vi "Main_Marvin Remake.vi"() -> ()   [LabVIEW 2017]
uses:
  Marvin ATP Remake 6.5.18 - Copy/PCAN_Driver/ControlCAN.llb/DevType.ctl
  Marvin ATP Remake 1.5.18/PCAN_Driver/ControlCAN.llb/CAN Channel.ctl
  Marvin ATP Remake 6.5.18 - Copy/PCAN_Driver/ControlCAN.llb/VCI_INIT_CONFIG.ctl
  Marvin ATP Remake 6.5.18 - Copy/PCAN_Driver/ControlCAN.llb/InitFlag.ctl
  Marvin ATP Remake 6.5.18 - Copy/PCAN_Driver/ControlCAN.llb/Fliter.ctl
  Marvin ATP Remake 6.5.18 - Copy/PCAN_Driver/ControlCAN.llb/Mode.ctl
  <vilib>/Utility/miscctls.llb/LVRowAndColumnTypeDef.ctl
  <vilib>/Utility/sysdir.llb/System Directory Type.ctl
  <vilib>/Utility/config.llb/Read Key (String).vi
  <vilib>/Utility/config.llb/Write Key (String).vi
  <vilib>/Utility/cursorutil.llb/Set Cursor (Icon Pict).vi
  Marvin CAN Bus 3.5.18/PCAN_Driver/ControlCAN.lvlib
  <vilib>/Utility/config.llb/NI_LVConfig.lvlib
panel:
  out "DSP Board S/N":string
  out "POWER Board S/N":string caption="DRIVER Board S/N"
  out "TesterVersion":string
  out "ClosePanel":bool=TRUE
  out "UUT SN Report":string
  out "Automation":bool
  out "Test Failed":bool
  out "AuxiOFFResult":bool
  out "AuxiONResult":bool
  out "SensCalResult":bool
  out "VisualInspectionResult":bool
  out "BurnResult":bool
  out "BurnSpeed":bool
  out "BurnTemp":bool
  out "BurnDC":bool
  out "TempControlResult":bool
  out "MotorTempResult":bool
  out "StopTimeResult":bool
  out "SpeedResult":bool=TRUE
  out "VenableDirectionResult":bool
  out "VenableResult":bool
  out "ComTestResult":bool=TRUE
  out "UUT SoftwareVer":string
  out "Next SN":i32
  in  "SetSN":bool
  out "Current SN":i32
  out "Cal":dbl
  out "AO[1]Meas":dbl
  out "FullSpeed2 Speed":dbl
  out "FullSpeed2 Current":dbl
  out "FullSpeed1 Current":dbl
  out "FullSpeed1 Speed":dbl
  out "MaxBurnInTempVal":dbl
  in  "Stop Burn-in":bool
  out "VISA Tester":refnum<visa-resource-name>
  out "UUT":u8
  out "CAN Status":bool
  in  "Channel 2":T1 caption="Channel" items=["Channel 1", "Channel 2"]
  out "Config_CANAT":T7 {"DevType" items=["USB-CAN"=3, "USB-CAN2"=4]; "CanIndex" items=["通道1", "通道2"]; "VCI_INIT_CONFIG"."Fliter" items=["接收所有类型"=3, "只接收标准帧"=4, "只接收扩展帧"=7]; "VCI_INIT_CONFIG"."Mode" items=["正常工作", "自测模式（环回）", "仅侦听模式"]; "VCI_INIT_CONFIG"."InitFlag" items=["使用Flash参数", "使用界面设置参数"]}
  out "Array":u64[][](array[numeric]) format="%016x"
  out "Motor Phase Current RMS":dbl
  out "Ambient Temperature":dbl
  out "Speed error":bool
  out "Commutation err":bool
  out "Under voltage/Over voltage":bool
  out "Derated drive temp":bool
  out "Motor Over temperature":bool
  out "Motor Sensor temp Fauilre":bool
  out "Drive Over temperature":bool
  out "Drive Sensor temp Failure":bool
  out "Ambient Over temp":bool
  out "Ambient Sensor temp":bool
  out "DC Voltage":dbl
  out "DC Current":dbl
  out "Power transistor Heat sink Temp.":dbl
  out "Motor Stator Temp.":dbl
  out "Motor Speed RPM":dbl
  out "ECS State":u16
  out "UUT":string="EBAY"
  in  "Logger Path":path
  in  "Report":bool
  in  "Start":bool
  in  "ATR":string[][](table)=[["Test Communication", "-", "-", "-", "-", ""], ["Set S/N", "-", "-", "-", "-", ""], ["Set Board Number", "-", "-", "-", "-", ""], [" ", "", "", "", "", ""], ["Test Communication", "-", "-", "-", "-", ""], ["Get S/N", "-", "-", "-", "", ""], ["Get Board Number", "-", "-", "-", "", ""], ["Get FW", "-", "-", "-", "", ""], ["Enable Motor", "", "", "", "", ""], ["Small position command", "", "", "", "", ""], ["Measure delta", "", "", "", "", ""], ["Velocity command", "", "", "", "", ""]]
  in  "Settings":bool
  in  "Refresh Button":bool
  out "Status":bool
  in  "VISA Marvin":refnum<visa-resource-name>="COM6"
  in  "Serial Com":bool
  in  "Help Button":bool
  out "Pannel User Message":string
  in  "Stop Button":bool
  # "Marvin"
  # "REDLER TECHNOLOGIES LTD"
  # "ver 1.2p"
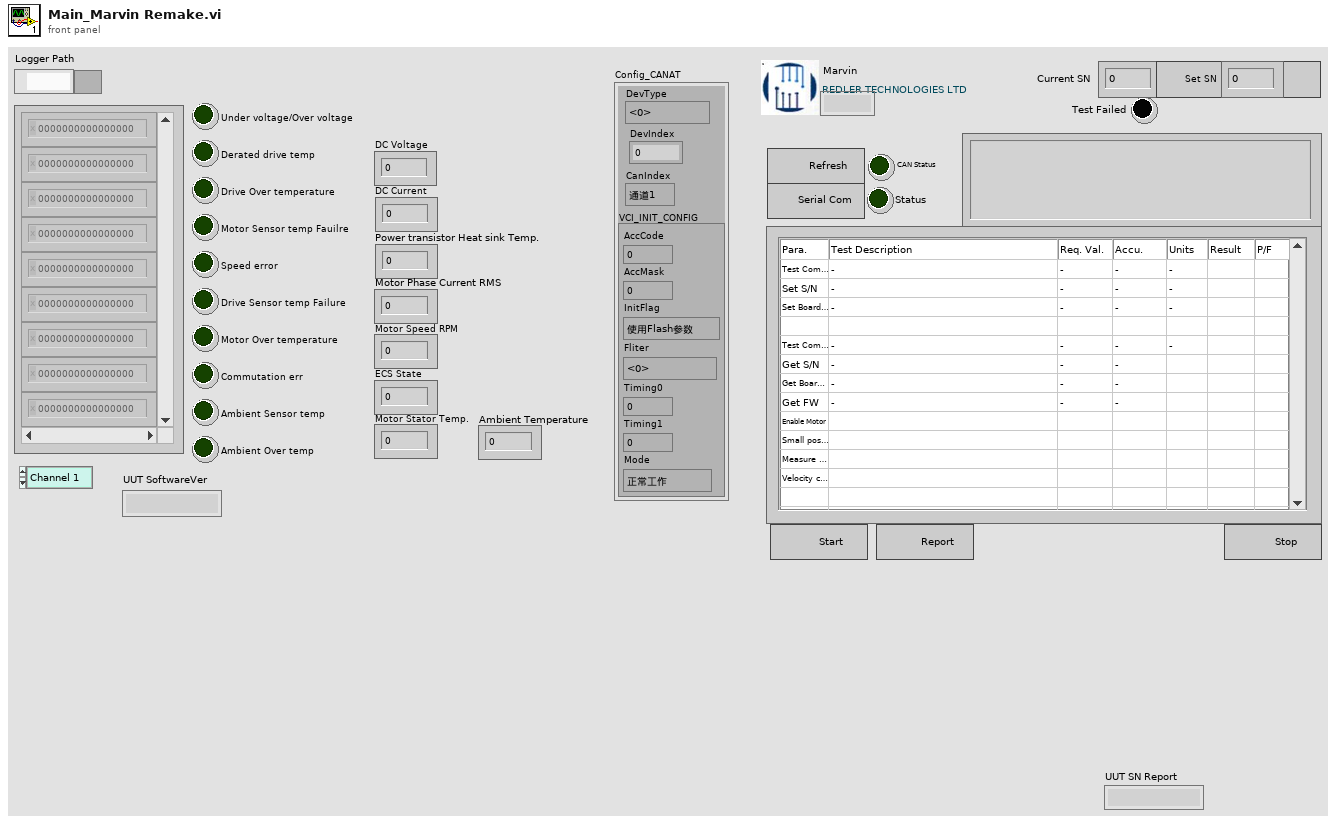
[diagram p1: front panel]
types:
  T1 = typedef "ControlCAN.lvlib/CAN Channel.ctl" = u32
  T2 = typedef "ControlCAN.lvlib/DevType.ctl" = u32
  T3 = typedef "ControlCAN.lvlib/VCI_INIT_CONFIG.ctl" = cluster{"AccCode":u32, "AccMask":u32, "InitFlag":T4, "Fliter":T5, "Timing0":u8, "Timing1":u8, "Mode":T6}
  T4 = typedef "ControlCAN.lvlib/InitFlag.ctl" = u32
  T5 = typedef "ControlCAN.lvlib/Fliter.ctl" = u8
  T6 = typedef "ControlCAN.lvlib/Mode.ctl" = u8
  T7 = cluster{"DevType":T2, "DevIndex":u32, "CanIndex":T1, "VCI_INIT_CONFIG":T3}
  T8 = cluster{"VISA":refnum<visa-resource-name>, "Array Test":enum16{"Auxiliary", "Temp Sens Cal", "Com Test", "Enable Test", "Speed Command", "Stop Time", "Temp Control", "Burn in", "Visual Inspec", "Empty"}[]}
  T9 = cluster{"ID":u32, "MSGTYPE":u8, "LEN":u8, "aDATA":u8[]}[]
  T10 = enum16{"Erase ATR Table", "Stop", "MainProgram", "Initialize"}
  T11 = typedef "NI_LVConfig.lvlib/Config Data RefNum.ctl" = refnum<k1>
  T12 = enum16{"K15", "K16", "K17", "Venable", "Firmeware", "Fan", "Power", "120C", "110C", "100C", "90C", "80C", "70C", "60C", "50C", "40C", "30C", "25C", "20C", "10C", "0C"}
  T13 = enum16{"Stop", "Result", "FullSpeed2", "MD[1]=1", "FullSpeed1", "MD[1]=0"}
  T14 = enum8{"Term1", "Term2", "Current", "Fan", "TempCPU"}
  T15 = enum16{"Stop", "AO[1]=Meas.", "TA[5]", "AO[1]=0", "Start"}
  T16 = enum16{"Stop", "BurnIn", "Ambient Temp", "MotorSpeed", "DC Current Measure", "Start"}
  T17 = enum16{"Auxiliary", "Temp Sens Cal", "Com Test", "Enable Test", "Speed Command", "Stop Time", "Temp Control", "Burn in", "Visual Inspec", "Empty"}[]
  T18 = enum16{"K15", "K16", "K17", "Venable", "Firmeware", "Fan", "Power", "120C", "110C", "100C", "90C", "80C", "70C", "60C", "50C", "40C", "30C", "25C", "20C", "10C", "0C"}[]
  T19 = enum32{"6000", "11500", "15100", "11500-2", "6000-2"}[]
  T20 = enum8{"Enabled", "Disabled", "Disabled and Grayed Out"}
  T21 = typedef "LVRowAndColumnTypeDef.ctl" = cluster{"Row":i32, "Column":i32}
  T22 = enum32{"Invalid", "Standard", "Closed", "Hidden", "Minimized", "Maximized"}
  T23 = cluster{"ID":u32, "MSGTYPE":u8, "LEN":u8, "aDATA":u8[]}
  T24 = enum16{"Auxiliary", "Temp Sens Cal", "Com Test", "Enable Test", "Speed Command", "Stop Time", "Temp Control", "Burn in", "Visual Inspec", "Empty"}
  T25 = enum16{"open", "replace", "create", "open or create", "replace or create", "replace or create with confirmation"}
  T26 = typedef "ControlCAN.lvlib/VCI_CAN_OBJ.ctl" = cluster{"ID":u32, "TimeStamp":u32, "TimeFlag":u8, "SendType":u8, "RemoteFlag":u8, "ExternFlag":u8, "DataLen":u8, "Data":u8[], "Reserved":u8[]}
  T27 = cluster{"Type":enum16{"接收", "发送"}, "Channel":T1, "Time":timestamp, "VCI_CAN_OBJ":T26}[]
  T28 = cluster{"Type":enum16{"接收", "发送"}, "Channel":T1, "Time":timestamp, "VCI_CAN_OBJ":T26}
  T29 = typedef "LVPoint32TypeDef.ctl" = cluster{"Horizontal":i32, "Vertical":i32}
  T30 = enum8{"Term1", "Term2", "Current", "Fan", "TempCPU"}[]
  T31 = typedef "System Directory Type.ctl" = i32
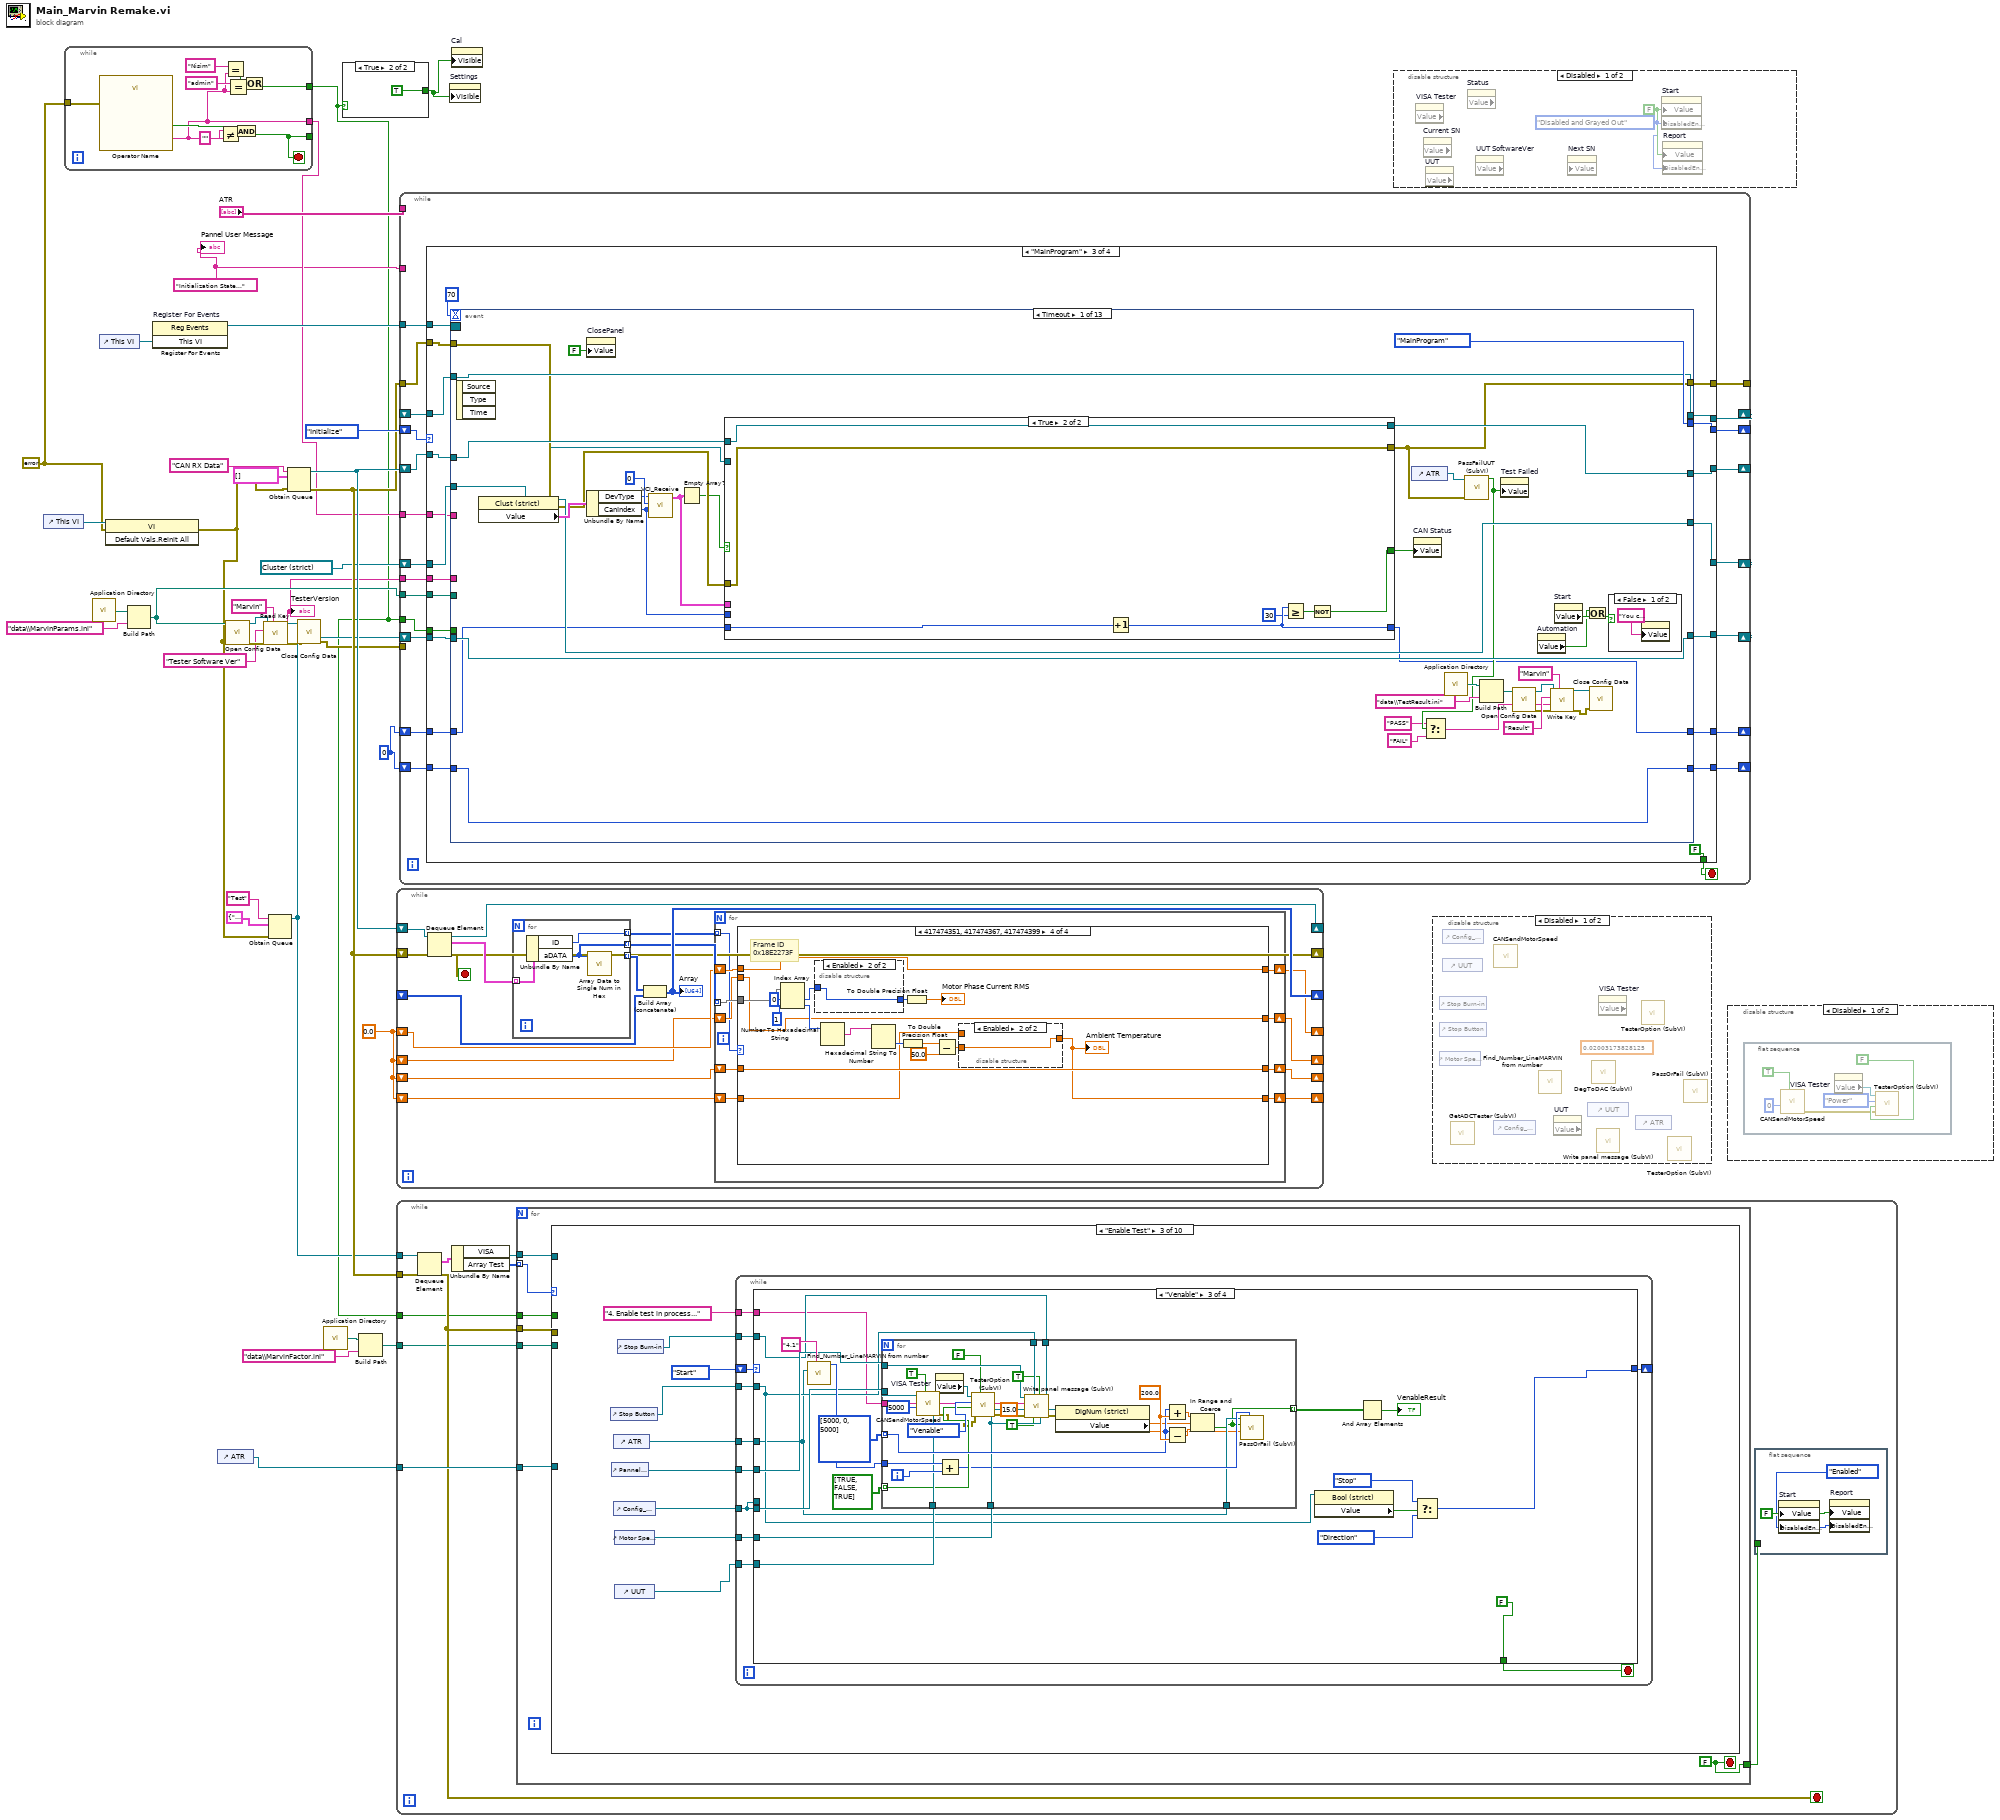
[diagram p0: block diagram]
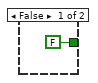
[diagram p2: hidden frame]
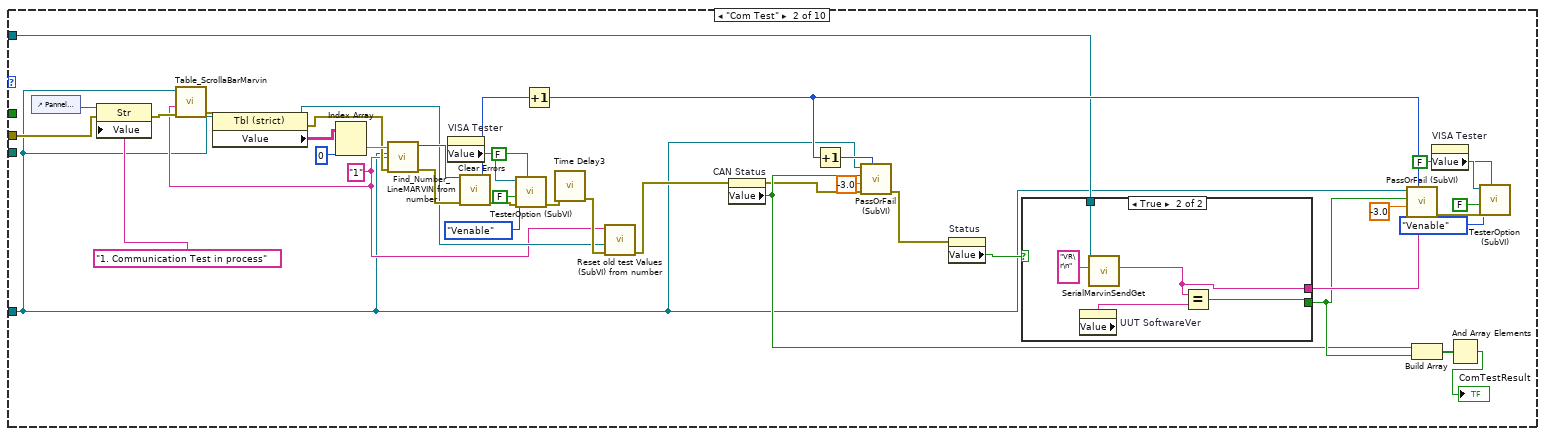
[diagram p7: hidden frame]
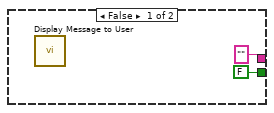
[diagram p8: hidden frame]
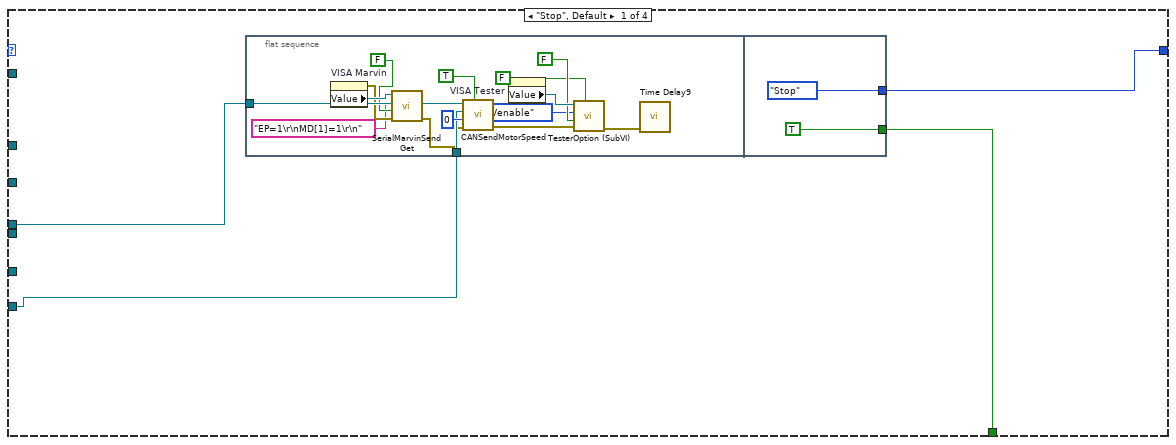
[diagram p9: hidden frame]
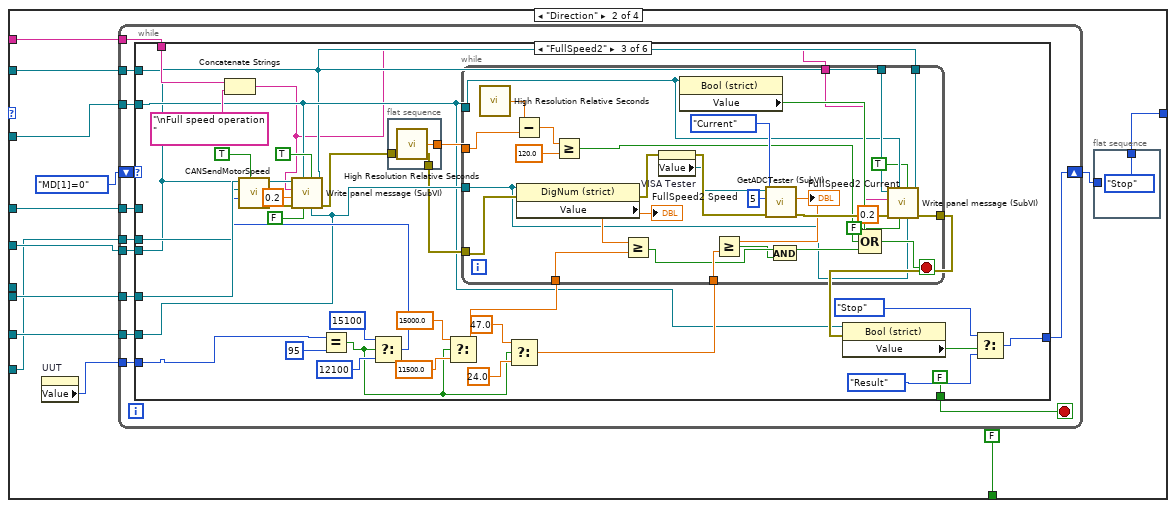
[diagram p10: hidden frame]
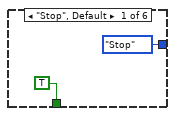
[diagram p11: hidden frame]
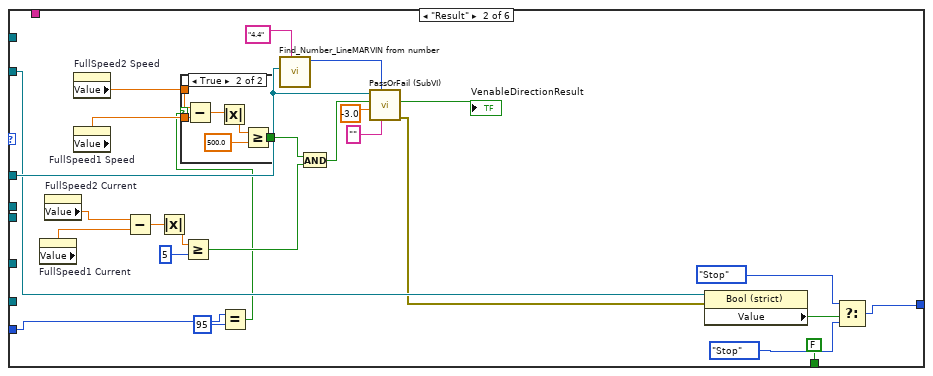
[diagram p12: hidden frame]
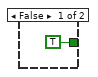
[diagram p13: hidden frame]
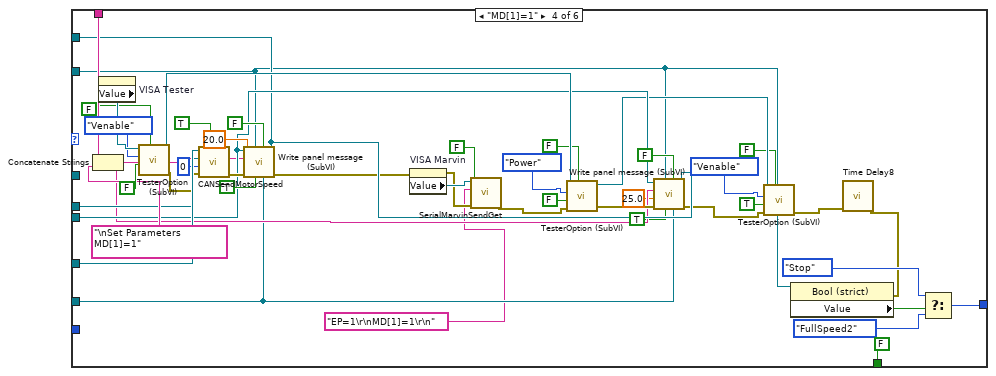
[diagram p14: hidden frame]
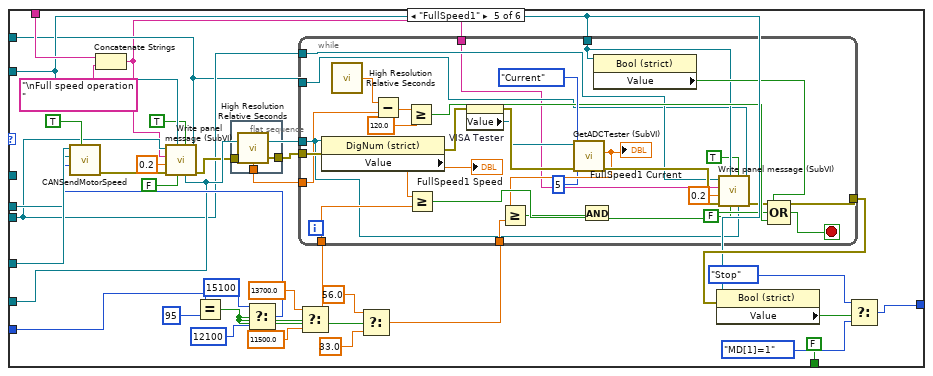
[diagram p15: hidden frame]
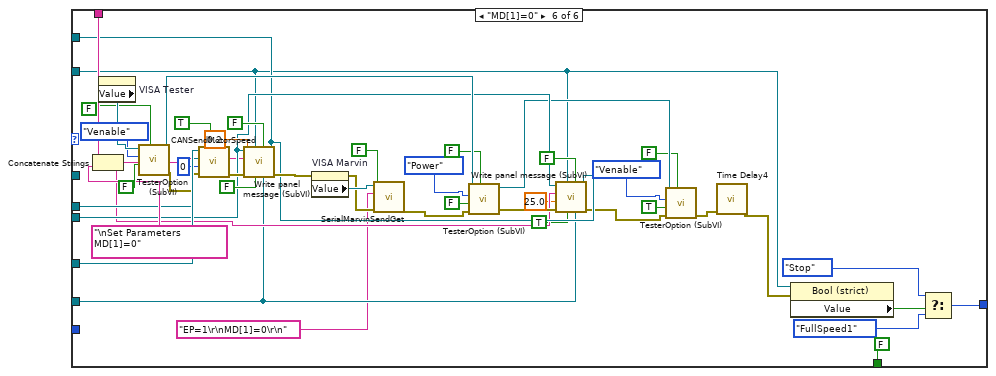
[diagram p16: hidden frame]
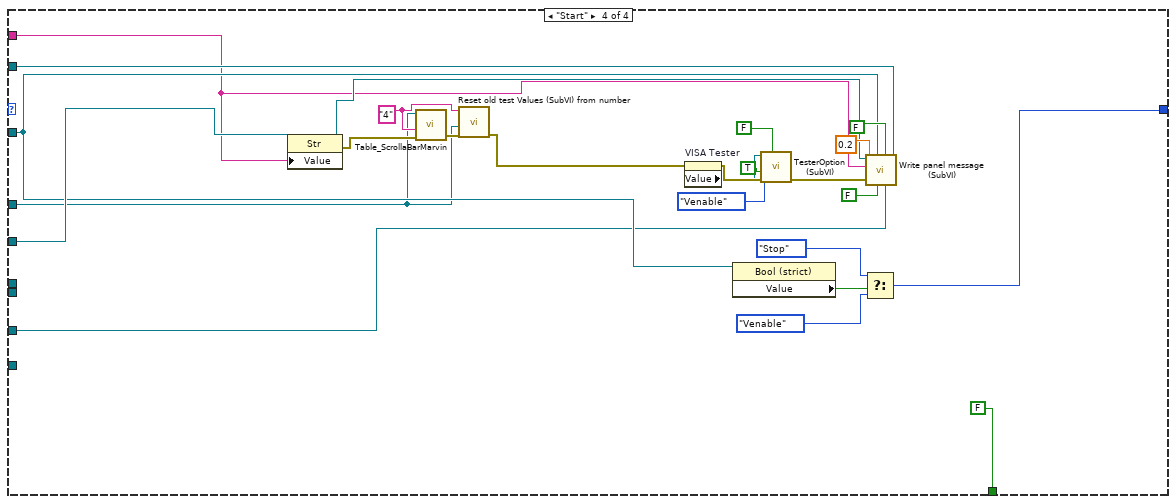
[diagram p17: hidden frame]
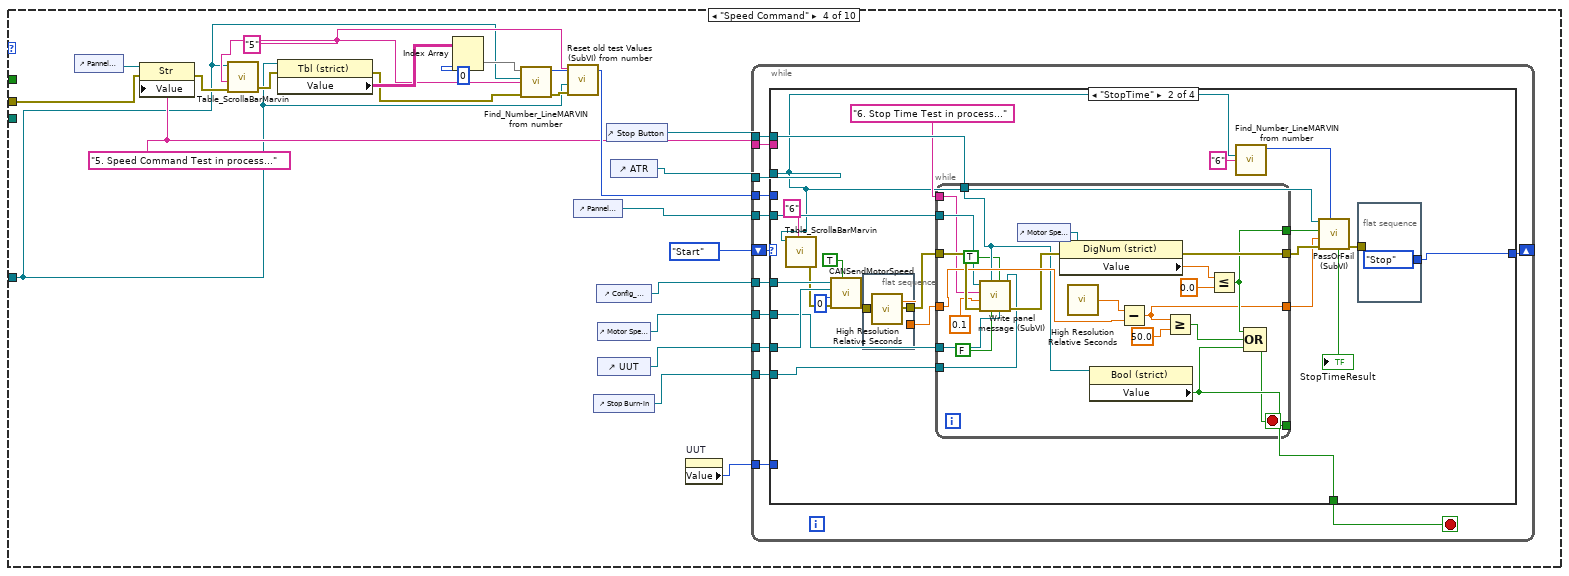
[diagram p18: hidden frame]
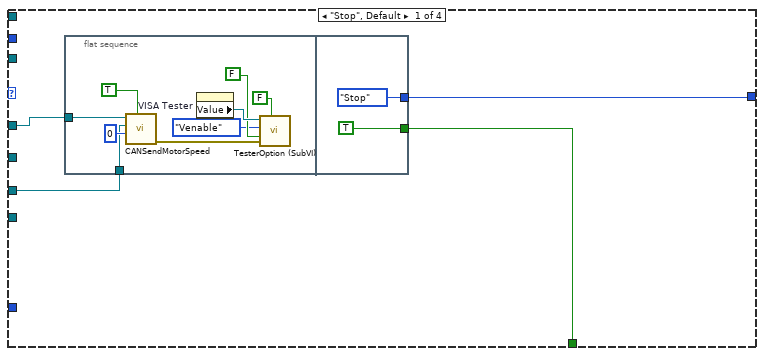
[diagram p19: hidden frame]
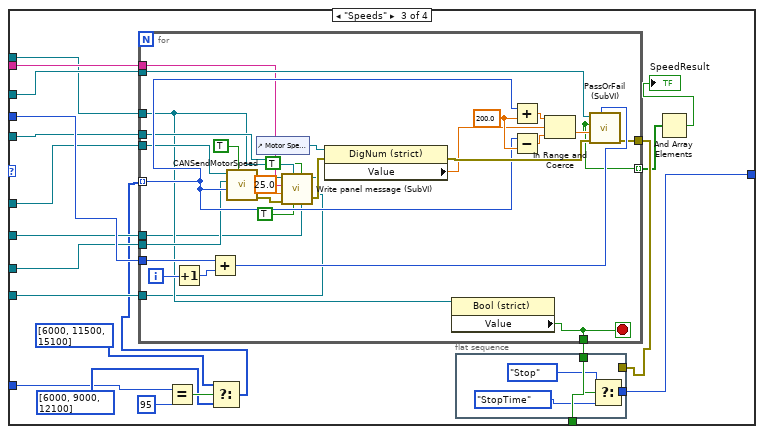
[diagram p20: hidden frame]
diagram:
  w19 = "Initialization State..."
  w1 = 0
  w26 = 0.0
  w4 = errorcluster {"status"=FALSE, "code"=0, "source"=""} ("error in (no error)")
  n1 = control-ref of="This VI"() -> (w5:refnum<vi>)
  n2 = while {
    tunnel: [w44] -> _
    tunnel: [w40] -> w21
    tunnel: [w41] -> w2
    tunnel: w4 -> [w37]
    stop <- w44 stop-if-true
    n3 = call "Operator Name"("error in (no error)"=w37) -> ("Operator Name"=w40:string, "OK"=w45:bool)  [unwired: 16 in, 1 out]
    n4 = Not Equal?(x=w40, y="") -> (x != y?=w46:bool)
    n5 = Equal?(x="Nisim", y=w40) -> (x = y?=w38:bool)
    n6 = Equal?(x="admin", y=w40) -> (x = y?=w42:bool)
    n7 = And(x=w45, y=w46) -> (x .and. y?=w44:bool)
    n8 = Or(x=w38, y=w42) -> (x .or. y?=w41:bool)
  }
  n9 = call <vilib>:"Application Directory.vi"() -> ("Application Directory"=w25:path)
  n10 = control-ref of="This VI"() -> (w23:refnum<vi>)
  n11 = invoke class="VI" method="Default Vals.Reinit All"(reference=w5, error in=w4) -> (error out=w3:errorcluster)  [unwired: 1 in, 2 out]
  n12 = Build Path(base path=w25, name or relative path="data\\MarvinParams.ini") -> (appended path=w8:path)
  n13 = register-events "Register For Events"(w23) -> (reference out=w22:refnum<event-registration>)  [unwired: 2 in, 1 out]
  n14 = control-ref of="ATR"() -> (w18:refnum<vi>)
  n15 = call <vilib>:"Open Config Data.vi"("error in (no error)"=w3, "configuration file path"=w8) -> ("error out"=w14:errorcluster, "refnum"=w13:T11)  [unwired: 1 in, 7 out]
  n16 = call-poly <vilib>:"Read Key.vi"("section"="Marvin", "error in (no error)"=w14, "key"="Tester Software Ver", "refnum"=w13) -> ("error out"=w11:errorcluster, "value"=w6:string, "refnum out"=w10:T11)  [unwired: 2 in, 3 out]
  "TesterVersion" <- w6
  n17 = Obtain Queue(name (unnamed)="Test", element data type=T8 {"VISA"="COM1", "Array Test"=[]}, error in (no error)=w3) -> (queue out=w30:refnum<queue>)  [unwired: 2 in, 2 out]
  n18 = Obtain Queue(name (unnamed)="CAN RX Data", element data type=T9 [], error in (no error)=w3) -> (queue out=w33:refnum<queue>, error out=w31:errorcluster)  [unwired: 2 in, 1 out]
  n19 = call <vilib>:"Close Config Data.vi"("error in (no error)"=w11, "refnum"=w10) -> ("error out"=w9:errorcluster)  [unwired: 8 in, 1 out]
  n20 = call <vilib>:"Application Directory.vi"() -> ("Application Directory"=w16:path)
  n21 = case shown="True" w2 {
    tunnel: [FALSE TRUE] -> w20
    frame False {
    }
    frame True {
    }
  }
  n22 = Build Path(base path=w16, name or relative path="data\\MarvinFactor.ini") -> (appended path=w15:path)
  n23 = while {
    shift-right: [w65] -> _
    shift-left: w33 -> [w67]
    shift-right: [w63] -> _
    shift-left: _ -> [w64]
    shift-right: [w59] -> _
    shift-left: w31 -> [w59]
    shift-right: [w57] -> _
    shift-left: w26 -> [w58]
    shift-right: [w56] -> _
    shift-left: w26 -> [w55]
    shift-right: [w54] -> _
    shift-left: w26 -> [w53]
    shift-right: [w52] -> _
    shift-left: w26 -> [w51]
    stop <- w66 stop-if-true
    n24 = Dequeue Element(queue=w67, error in (no error)=w59) -> (queue out=w65:refnum<queue>, element=w60:T9, error out=w66:errorcluster)  [unwired: 1 in, 1 out]
    n25 = for {
      tunnel: [w217] -> w62 mode=indexing
      tunnel: w60 -> [w216] mode=indexing
      tunnel: [w215] -> w61 mode=indexing
      tunnel: [w214] -> w50 mode=indexing
      n26 = Unbundle By Name(w216) -> ("ID"=w214:u32, "aDATA"=w215:u8[])
      n27 = call "Array Data to Single Num in Hex.vi"("aDATA"=w215) -> ("Numeric"=w217:u64)  [unwired: 10 in]
    }
    n28 = Build Array (concatenate)(w62, w64) -> (w63:u64[][])
    "Array" <- w63
    n29 = for {
      tunnel: w61 -> [w77] mode=indexing
      shift-right: [w75] -> w57
      shift-left: w58 -> [w76]
      shift-right: [w74] -> w56
      shift-left: w55 -> [w73]
      shift-right: [w72] -> w54
      shift-left: w53 -> [w71]
      shift-right: [w70] -> w52
      shift-left: w51 -> [w69]
      tunnel: w50 -> [w68] mode=indexing
      n30 = case shown="417474351, 417474367, 417474399" w68 {
        tunnel: w77 -> [w110 _ w166 w202]
        tunnel: w76 -> [w86 w151 w155 w191]
        tunnel: [w85 w151 w155 w191] -> w75
        tunnel: [w83 w150 w154 w190] -> w74
        tunnel: w73 -> [w82 w150 w154 w190]
        tunnel: [w80 w149 w153 w189] -> w72
        tunnel: w71 -> [w79 w149 w153 w189]
        tunnel: [w78 w148 w152 w187] -> w70
        tunnel: w69 -> [w78 w148 w152 w186]
        frame 417408815, 417408831, 417408863 {
          # "Frame ID\n0x18E1273F"
          n31 = Index Array(array=w110, index #1=0 ("index"), index #2=1 ("index"), index #3=2 ("index"), index #4=3 ("index"), index #5=4 ("index"), index #6=5 ("index"), index #7=6 ("index"), index #8=7 ("index")) -> (element #1=w94:u8, element #2=w96:u8, element #3=w97:u8, element #4=w101:u8, element #5=w104:u8, element #6=w108:u8, element #7=w109:u8, element #8=w107:u8)
          n32 = Number To Hexadecimal String(2:w107) -> (0:w121:string)  [unwired: 1 in]
          n33 = Join Numbers(hi=w109, lo=w108) -> ((hi.lo)=w128:u16)
          n34 = Join Numbers(hi=w97, lo=w96) -> ((hi.lo)=w98:u16)
          n35 = Number To Hexadecimal String(2:w104) -> (0:w105:string)  [unwired: 1 in]
          n36 = Number To Hexadecimal String(2:w128) -> (0:w127:string)  [unwired: 1 in]
          n37 = Number To Hexadecimal String(2:w94) -> (0:w95:string)  [unwired: 1 in]
          n38 = Number To Hexadecimal String(2:w98) -> (0:w99:string)  [unwired: 1 in]
          n39 = Number To Hexadecimal String(2:w101) -> (0:w102:string)  [unwired: 1 in]
          n40 = Hexadecimal String To Number(string=w121) -> (number=w120:u32)  [unwired: 2 in, 1 out]
          n41 = To Double Precision Float(number=w120) -> (double precision float=→"DC Current":dbl)
          n42 = Hexadecimal String To Number(string=w105) -> (number=w106:u32)  [unwired: 2 in, 1 out]
          n43 = Hexadecimal String To Number(string=w127) -> (number=w126:u32)  [unwired: 2 in, 1 out]
          n44 = Hexadecimal String To Number(string=w95) -> (number=w92:u32)  [unwired: 2 in, 1 out]
          n45 = Hexadecimal String To Number(string=w99) -> (number=w100:u32)  [unwired: 2 in, 1 out]
          n46 = Hexadecimal String To Number(string=w102) -> (number=w103:u32)  [unwired: 2 in, 1 out]
          n47 = To Double Precision Float(number=u32 10 ("y")) -> (double precision float=w124:dbl)
          n48 = To Double Precision Float(number=w126) -> (double precision float=w123:dbl)
          n49 = To Double Precision Float(number=w106) -> (double precision float=w89:dbl)
          n50 = To Double Precision Float(number=w100) -> (double precision float=w87:dbl)
          n51 = To Double Precision Float(number=w103) -> (double precision float=w91:dbl)
          n52 = Divide(x=w123, y=w124) -> (x/y=→"DC Voltage":dbl)
          n53 = To Unsigned Word Integer(number=w92) -> (unsigned 16bit integer=→"ECS State":u16)
          n54 = disable-structure shown="Enabled" {
            disable-tunnel: w87 -> [w146 w147]
            disable-tunnel: w86 -> [w145 _]
            disable-tunnel: [w143 w147] -> w85
            frame Disabled {
              n55 = call "Filter (SubVI).vi"("Delta"=5000.0, "NewVal"=w146, "OldVal"=w145) -> ("Val"=w143:dbl)  [unwired: 8 in]
            }
            frame Enabled {
            }
          }
          "Motor Speed RPM" <- w85
          n56 = Subtract(x=w89, y=50.0 ("x")) -> (x-y=w81:dbl)
          n57 = Subtract(x=w91, y=50.0 ("x")) -> (x-y=w84:dbl)
          n58 = disable-structure shown="Enabled" {
            disable-tunnel: w81 -> [w133 w135]
            disable-tunnel: [w130 w135] -> w80
            disable-tunnel: w79 -> [w129 _]
            frame Disabled {
              n59 = Less Than 0?(x=w133) -> (x < 0?=w134:bool)
              n60 = Select(t=w129, s=w134, f=w133) -> (s? t:f=w132:dbl)
              n61 = call "Filter (SubVI).vi"("Delta"=100.0, "NewVal"=w132, "OldVal"=w129) -> ("Val"=w130:dbl)  [unwired: 8 in]
            }
            frame Enabled {
            }
          }
          "Power transistor Heat sink Temp." <- w80
          n62 = disable-structure shown="Enabled" {
            disable-tunnel: w84 -> [w139 w142]
            disable-tunnel: [w138 w142] -> w83
            disable-tunnel: w82 -> [w137 _]
            frame Disabled {
              n63 = Less Than 0?(x=w139) -> (x < 0?=w141:bool)
              n64 = Select(t=w137, s=w141, f=w139) -> (s? t:f=w140:dbl)
              n65 = call "Filter (SubVI).vi"("Delta"=130.0, "NewVal"=w140, "OldVal"=w137) -> ("Val"=w138:dbl)  [unwired: 8 in]
            }
            frame Enabled {
            }
          }
          "Motor Stator Temp." <- w83
        }
        frame Default {
        }
        frame 417539887, 417539903, 417539935 {
          # "Framde ID\n0x18E3273F"
          n66 = control-ref of="UUT"() -> (w156:refnum<vi>)
          n67 = property on="Property Node" class="DigNum (strict)"(reference=w156) -> ("Value"=w157:u8)  [unwired: 1 in, 2 out]
          n68 = Index Array(array=w166, index #1=0 ("index"), index #2=1 ("index")) -> (element #1=w164:u8, element #2=w159:u8)
          n69 = Number To Boolean Array(number=w164) -> (Boolean array=w163:bool[])
          n70 = Number To Boolean Array(number=w159) -> (Boolean array=w161:bool[])
          n71 = Boolean To (0,1)(Boolean=w161) -> (0, 1=w158:i16[])
          n72 = Boolean To (0,1)(Boolean=w163) -> (0, 1=w162:i16[])
          n73 = case shown="95" w157 {
            tunnel: w158 -> [_ w167]
            frame 0, Default {
            }
            frame 95 {
              n74 = for {
                tunnel: w167 -> [w172] mode=indexing
                i -> [w168]
                stop <- w170 stop-if-true
                n75 = Not Equal To 0?(x=w172) -> (x != 0?=w171:bool)
                n76 = case shown="0, Default" w168 {
                  tunnel: w171 -> [w173 w174]
                  frame 0, Default {
                    "Ambient Sensor temp" <- w173
                  }
                  frame 1 {
                    "Ambient Over temp" <- w174
                  }
                }
                n77 = Equal?(x=w168, y=1.0) -> (x = y?=w170:bool)
              }
            }
          }
          n78 = for {
            tunnel: w162 -> [w176] mode=indexing
            i -> [w177]
            n79 = Not Equal To 0?(x=w176) -> (x != 0?=w175:bool)
            n80 = case shown="2" w177 {
              tunnel: w175 -> [w178 w179 w180 w181 w182 w183 w184 w185]
              frame 0, Default {
                "Drive Sensor temp Failure" <- w178
              }
              frame 1 {
                "Drive Over temperature" <- w179
              }
              frame 2 {
                "Motor Sensor temp Fauilre" <- w180
              }
              frame 3 {
                "Motor Over temperature" <- w181
              }
              frame 4 {
                "Derated drive temp" <- w182
              }
              frame 5 {
                "Under voltage/Over voltage" <- w183
              }
              frame 6 {
                "Commutation err" <- w184
              }
              frame 7 {
                "Speed error" <- w185
              }
            }
          }
        }
        frame 417474351, 417474367, 417474399 {
          # "Frame ID\n0x18E2273F"
          n81 = Index Array(array=w202, index #1=0 ("index"), index #2=1 ("index")) -> (element #1=w199:u8, element #2=w196:u8)
          n82 = disable-structure shown="Enabled" {
            disable-tunnel: [w212 w213] -> w200
            disable-tunnel: w199 -> [w211 w213]
            frame Disabled {
              n83 = Number To Hexadecimal String(2:w211) -> (0:w210:string)  [unwired: 1 in]
              n84 = Hexadecimal String To Number(string=w210) -> (number=w212:u32)  [unwired: 2 in, 1 out]
            }
            frame Enabled {
            }
          }
          n85 = Number To Hexadecimal String(2:w196) -> (0:w194:string)  [unwired: 1 in]
          n86 = Hexadecimal String To Number(string=w194) -> (number=w195:u32)  [unwired: 2 in, 1 out]
          n87 = To Double Precision Float(number=w195) -> (double precision float=w193:dbl)
          n88 = To Double Precision Float(number=w200) -> (double precision float=→"Motor Phase Current RMS":dbl)
          n89 = Subtract(x=w193, y=50.0) -> (x-y=w188:dbl)
          n90 = disable-structure shown="Enabled" {
            disable-tunnel: w188 -> [w207 w209]
            disable-tunnel: [w204 w209] -> w187
            disable-tunnel: w186 -> [w203 _]
            frame Disabled {
              n91 = Less Than 0?(x=w207) -> (x < 0?=w208:bool)
              n92 = Select(t=w203, s=w208, f=w207) -> (s? t:f=w206:dbl)
              n93 = call "Filter (SubVI).vi"("Delta"=65.0, "NewVal"=w206, "OldVal"=w203) -> ("Val"=w204:dbl)  [unwired: 8 in]
            }
            frame Enabled {
            }
          }
          "Ambient Temperature" <- w187
        }
      }
    }
  }
  n94 = while {
    tunnel: w18 -> [w227]
    tunnel: w31 -> [w225]
    tunnel: w30 -> [w226]
    tunnel: w15 -> [w219]
    tunnel: w2 -> [w218]
    stop <- w221 stop-if-true
    n95 = Dequeue Element(queue=w226, error in (no error)=w225) -> (element=w224:T8, error out=w221:errorcluster)  [unwired: 1 in, 2 out]
    n96 = Unbundle By Name(w224) -> ("VISA"=w223:refnum<visa-resource-name>, "Array Test"=w222:T17)
    n97 = for {
      tunnel: w222 -> [w233] mode=indexing
      tunnel: w223 -> [w236]
      tunnel: w227 -> [w235]
      tunnel: w221 -> [w234]
      tunnel: [w232] -> w220
      tunnel: w219 -> [w231]
      tunnel: w218 -> [w230]
      stop <- w232 stop-if-true
      w232 = FALSE
      n98 = case shown="\"Enable Test\"" w233 {
        tunnel: w236 -> [_ w261 _ _ w849 _ _ _ w1451 _]
        tunnel: w235 -> [_ w237 _ w684 w845 w993 _ w1424 w1446 w1657]
        tunnel: w234 -> [_ w265 _ w699 w855 w1005 _ w1412 w1456 w1669]
        tunnel: w231 -> [_ _ _ _ _ w1007 _ _ _ _]
        tunnel: w230 -> [_ _ _ _ _ _ w1173 _ _ _]
        frame "Empty", Default {
        }
        frame "Com Test" {
          w244 = "1" ("Test Paragraph")
          n99 = control-ref of="Pannel User Message"() -> (w266:refnum<vi>)
          n100 = property class="Str"(reference=w266, error in=w265, "Value"="1. Communication Test in process") -> (error out=w264:errorcluster)  [unwired: 1 out]
          n101 = call "Table_ScrollaBarMarvin.vi"("error in"=w264, "Line to focus"=w244, "TableIn"=w237) -> ("error out"=w267:errorcluster)  [unwired: 1 in, 2 out]
          n102 = property class="Tbl (strict)"(reference=w237, error in=w267) -> (reference out=w245:refnum<vi>, error out=w274:errorcluster, "Value"=w275:string[][])
          n103 = Index Array(array=w275, index (col)=0 ("disabled index (col)")) -> (element=w276:string[])  [unwired: 1 in]
          n104 = call "Find_Number_LineMARVIN from number.vi"("Test Paragraph"=w244, "error in"=w274, "TableIn"=w237, "Row Headers[]"=w276) -> ("error out"=w272:errorcluster, "Line number"=w271:i32)  [unwired: 1 in, 2 out]
          n105 = property on="VISA Tester" class="VISAName"() -> ("Value"=w255:refnum<visa-resource-name>)  [unwired: 2 in, 2 out]
          n106 = call <vilib>:"Clear Errors.vi"("error in (no error)"=w272) -> ("error out"=w257:errorcluster)  [unwired: 5 in, 1 out]
          n107 = call "TesterOption (SubVI).vi"("2 Options"=FALSE, "error in (no error)"=w257, "On/Off"=FALSE, "Tester Option"=T12."Venable", "VISA Refnum in"=w255) -> ("error out"=w256:errorcluster)  [unwired: 5 in, 1 out]
          n108 = Increment(x=w271) -> (x+1=w270:i32)
          n109 = call "Time Delay3"("error in (no error)"=w256) -> ("error out"=w268:errorcluster)  [unwired: 10 in]
          n110 = call "Reset old test Values (SubVI) from number.vi"("error in"=w268, "Atr in"=w245, "Test Paragraph"=w244) -> ("error out"=w239:errorcluster)  [unwired: 8 in]
          n111 = property on="CAN Status" class="Bool (strict)"(error in=w239) -> (error out=w238:errorcluster, "Value"=w240:bool)  [unwired: 1 in, 1 out]
          n112 = Increment(x=w270) -> (x+1=w269:i32)
          n113 = call "PassOrFail (SubVI).vi"("index (row)"=w269, "error in (no error)"=w238, "Data in"=-3.0, "Pass?Fail"=w240, "Table in"=w237) -> ("error out"=w260:errorcluster)  [unwired: 6 in]
          n114 = property on="Status" class="Bool (strict)"(error in=w260) -> ("Value"=w262:bool)  [unwired: 1 in, 2 out]
          n115 = case shown="True" w262 {
            tunnel: w261 -> [_ w283]
            tunnel: [FALSE w280] -> w242
            tunnel: ["" ("read buffer") w279] -> w259
            frame False {
              n116 = call "Display Message to User"() -> ()  [unwired: 10 in, 2 out]
            }
            frame True {
              n117 = property on="UUT SoftwareVer" class="Str"() -> ("Value"=w281:string)  [unwired: 2 in, 2 out]
              n118 = call "SerialMarvinSendGet.vi"("write buffer"="VR\r\n", "VISA resource name"=w283) -> ("read buffer"=w279:string)  [unwired: 8 in, 1 out]
              n119 = Equal?(x=w279, y=w281) -> (x = y?=w280:bool)
            }
          }
          n120 = call "PassOrFail (SubVI).vi"("String Res"=w259, "index (row)"=w270, "Data in"=-3.0, "Pass?Fail"=w242, "Table in"=w237) -> ("error out"=w251:errorcluster)  [unwired: 6 in]
          n121 = Build Array(w240, w242) -> (w243:bool[])
          n122 = property on="VISA Tester" class="VISAName"() -> ("Value"=w250:refnum<visa-resource-name>)  [unwired: 2 in, 2 out]
          n123 = And Array Elements(Boolean array=w243) -> (logical AND=→"ComTestResult":bool)
          n124 = call "TesterOption (SubVI).vi"("2 Options"=FALSE, "error in (no error)"=w251, "On/Off"=FALSE, "Tester Option"=T12."Venable", "VISA Refnum in"=w250) -> ()  [unwired: 5 in, 2 out]
        }
        frame "Enable Test" {
          n125 = control-ref of="Stop Button"() -> (w286:refnum<vi>)
          n126 = control-ref of="Pannel User Message"() -> (w288:refnum<vi>)
          n127 = control-ref of="ATR"() -> (w287:refnum<vi>)
          n128 = control-ref of="Config_CANAT"() -> (w289:refnum<vi>)
          n129 = control-ref of="Motor Speed RPM"() -> (w290:refnum<vi>)
          n130 = control-ref of="UUT"() -> (w291:refnum<vi>)
          n131 = control-ref of="Stop Burn-in"() -> (w292:refnum<vi>)
          n132 = while {
            shift-right: [w297] -> _
            shift-left: enum16{"Stop", "Direction", "Venable", "Start"}."Start" -> [w303]
            tunnel: w286 -> [w302]
            tunnel: w287 -> [w301]
            tunnel: w288 -> [w300]
            tunnel: w289 -> [w293]
            tunnel: w290 -> [w299]
            tunnel: w291 -> [w294]
            tunnel: w292 -> [w296]
            tunnel: "4. Enable test in process..." ("Strin") -> [w295]
            stop <- w298 stop-if-true
            n133 = case shown="\"Venable\"" w303 {
              tunnel: w302 -> [_ w335 w616 w664]
              tunnel: w301 -> [_ w330 w614 w659]
              tunnel: w300 -> [_ w333 w618 w670]
              tunnel: w293 -> [_ w336 w621 _]
              tunnel: w299 -> [_ w332 w619 w662]
              tunnel: w294 -> [w304 w326 w620 _]
              tunnel: [w307 FALSE FALSE FALSE] -> w298
              tunnel: [w305 w329 w615 w668] -> w297
              tunnel: w296 -> [_ w334 w617 w663]
              tunnel: w295 -> [_ w331 w613 w661]
              tunnel: w293 -> [w306 _ _ _]
              frame "Stop", Default {
                n134 = flat-sequence {
                  tunnel: w304 -> [w318]
                  tunnel: w306 -> [w317]
                  tunnel: [TRUE] -> w307
                  tunnel: [enum16{"Stop", "Direction", "Venable", "Start"}."Stop"] -> w305
                  frame #0 {
                    n135 = property on="VISA Marvin" class="VISAName"() -> (error out=w311:errorcluster, "Value"=w312:refnum<visa-resource-name>)  [unwired: 2 in, 1 out]
                    n136 = call "SerialMarvinSendGet.vi"("error in (no error)"=w311, "Clear Log"=FALSE, "write buffer"="EP=1\r\nMD[1]=1\r\n", "VISA resource name"=w312) -> ("error out"=w308:errorcluster)  [unwired: 6 in, 1 out]
                    n137 = call "CANSendMotorSpeed.vi"("Remote"=TRUE, "error in (no error)"=w308, "Motor Speed RPM"=u16 0, "UUT"=w318, "CAN Cluster in"=w317) -> ("error out"=w321:errorcluster)  [unwired: 6 in]
                    n138 = property on="VISA Tester" class="VISAName"() -> ("Value"=w322:refnum<visa-resource-name>)  [unwired: 2 in, 2 out]
                    n139 = call "TesterOption (SubVI).vi"("2 Options"=FALSE, "error in (no error)"=w321, "On/Off"=FALSE, "Tester Option"=T12."Venable", "VISA Refnum in"=w322) -> ("error out"=w313:errorcluster)  [unwired: 5 in, 1 out]
                    n140 = call "Time Delay9"("error in (no error)"=w313) -> ()  [unwired: 10 in, 1 out]
                  }
                  frame #1 {
                  }
                }
              }
              frame "Direction" {
                n141 = property on="UUT" class="DigNum (strict)"() -> ("Value"=w325:u8)  [unwired: 2 in, 2 out]
                n142 = while {
                  shift-right: [w349] -> w328
                  shift-left: T13."MD[1]=0" -> [w350]
                  tunnel: w336 -> [w347]
                  tunnel: w326 -> [w346]
                  tunnel: w335 -> [w345]
                  tunnel: w334 -> [w344]
                  tunnel: w333 -> [w343]
                  tunnel: w332 -> [w342]
                  tunnel: w331 -> [w341]
                  tunnel: w330 -> [w340]
                  tunnel: w325 -> [w339]
                  stop <- w348 stop-if-true
                  n143 = case shown="\"FullSpeed2\"" w350 {
                    tunnel: [T13."Stop" w374 w416 w496 w529 w609] -> w349
                    tunnel: [TRUE FALSE FALSE FALSE FALSE FALSE] -> w348
                    tunnel: w347 -> [_ _ w414 w490 w527 w603]
                    tunnel: w346 -> [_ _ w410 w469 w523 w581]
                    tunnel: w345 -> [_ w361 w389 w460 w505 w571]
                    tunnel: w344 -> [_ _ w387 w470 w503 w582]
                    tunnel: w343 -> [_ _ w388 w471 w504 w583]
                    tunnel: w342 -> [_ _ w405 w458 w519 w577]
                    tunnel: w341 -> [_ _ w400 w479 w517 w591]
                    tunnel: w340 -> [_ w365 _ _ _ _]
                    tunnel: w339 -> [_ w353 w385 _ w498 _]
                    frame "Stop", Default {
                    }
                    frame "Result" {
                      n144 = property on="FullSpeed1 Current" class="DigNum (strict)"() -> ("Value"=w369:dbl)  [unwired: 2 in, 2 out]
                      n145 = property on="FullSpeed2 Current" class="DigNum (strict)"() -> ("Value"=w370:dbl)  [unwired: 2 in, 2 out]
                      n146 = property on="FullSpeed2 Speed" class="DigNum (strict)"() -> ("Value"=w372:dbl)  [unwired: 2 in, 2 out]
                      n147 = property on="FullSpeed1 Speed" class="DigNum (strict)"() -> ("Value"=w371:dbl)  [unwired: 2 in, 2 out]
                      n148 = Subtract(x=w370, y=w369) -> (x-y=w368:dbl)
                      n149 = Absolute Value(x=w368) -> (abs(x)=w357:dbl)
                      n150 = Greater Or Equal?(x=w357, y=u32 5) -> (x >= y?=w363:bool)
                      n151 = Equal?(x=w353, y=u8 95) -> (x = y?=w355:bool)
                      n152 = case shown="True" w355 {
                        tunnel: w372 -> [_ w383]
                        tunnel: w371 -> [_ w382]
                        tunnel: [TRUE w379] -> w364
                        frame False {
                        }
                        frame True {
                          n153 = Subtract(x=w383, y=w382) -> (x-y=w384:dbl)
                          n154 = Absolute Value(x=w384) -> (abs(x)=w381:dbl)
                          n155 = Greater Or Equal?(x=w381, y=500.0) -> (x >= y?=w379:bool)
                        }
                      }
                      n156 = call "Find_Number_LineMARVIN from number.vi"("Test Paragraph"="4.4", "TableIn"=w365) -> ("Line number"=w362:i32)  [unwired: 3 in, 3 out]
                      n157 = And(x=w364, y=w363) -> (x .and. y?=w354:bool)
                      "VenableDirectionResult" <- w354
                      n158 = call "PassOrFail (SubVI).vi"("String Res"="", "index (row)"=w362, "Data in"=-3.0, "Pass?Fail"=w354, "Table in"=w365) -> ("error out"=w360:errorcluster)  [unwired: 6 in]
                      n159 = property class="Bool (strict)"(reference=w361, error in=w360) -> ("Value"=w377:bool)  [unwired: 2 out]
                      n160 = Select(t=T13."Stop", s=w377, f=T13."Stop") -> (s? t:f=w374:T13)
                    }
                    frame "FullSpeed2" {
                      n161 = Concatenate Strings(w400, "\nFull speed operation " ("string")) -> (w386:string)
                      n162 = Equal?(x=w385, y=u8 95) -> (x = y?=w395:bool)
                      n163 = Select(t=u16 15100, s=w395, f=u16 12100 ("y")) -> (s? t:f=w409:u16)
                      n164 = call "CANSendMotorSpeed.vi"("Remote"=TRUE, "Motor Speed RPM"=w409, "UUT"=w410, "CAN Cluster in"=w414) -> ("error out"=w407:errorcluster)  [unwired: 7 in]
                      n165 = call "Write panel message (SubVI).vi"("Stop BurnIn"=w387, 4:"rpm"=w405, 5:"rpm"=TRUE ("rpm"), "PrintTime"=FALSE, "Stop"=w389, "error in (no error)"=w407, "Time to wait"=0.2, "Strin"=w386, "String in"=w388) -> ("error out"=w392:errorcluster)  [unwired: 2 in]
                      n166 = flat-sequence {
                        tunnel: w392 -> [w421]
                        tunnel: [w421] -> w391
                        tunnel: [w420] -> w390
                        frame #0 {
                          n167 = call <vilib>:"High Resolution Relative Seconds.vi"() -> ("relative seconds"=w420:dbl)
                        }
                      }
                      n168 = Select(t=15000.0, s=w395, f=11500.0) -> (s? t:f=w394:dbl)
                      n169 = Select(t=47.0, s=w395, f=24.0) -> (s? t:f=w393:dbl)
                      n170 = while {
                        tunnel: w405 -> [w423]
                        tunnel: w391 -> [w451]
                        tunnel: [w431] -> w402
                        tunnel: w394 -> [w444]
                        tunnel: w393 -> [w443]
                        tunnel: w390 -> [w439]
                        tunnel: w389 -> [w429]
                        tunnel: w388 -> [w430]
                        tunnel: w387 -> [w427]
                        tunnel: w386 -> [w426]
                        stop <- w441 stop-if-true
                        n171 = call <vilib>:"High Resolution Relative Seconds.vi"() -> ("relative seconds"=w440:dbl)
                        n172 = Subtract(x=w440, y=w439) -> (x-y=w438:dbl)
                        n173 = property class="DigNum (strict)"(reference=w423, error in=w451) -> (error out=w450:errorcluster, "Value"=w445:dbl)  [unwired: 1 out]
                        "FullSpeed2 Speed" <- w445
                        n174 = Greater Or Equal?(x=w438, y=120.0) -> (x >= y?=w436:bool)
                        n175 = Greater Or Equal?(x=w445, y=w444) -> (x >= y?=w435:bool)
                        n176 = property on="VISA Tester" class="VISAName"(error in=w450) -> (error out=w449:errorcluster, "Value"=w448:refnum<visa-resource-name>)  [unwired: 1 in, 1 out]
                        n177 = property class="Bool (strict)"(reference=w429) -> ("Value"=w434:bool)  [unwired: 1 in, 2 out]
                        n178 = call "GetADCTester (SubVI).vi"("error in (no error)"=w449, "GetADCTester"=T14."Current", "TimeToGet"=5, "VISA Refnum in"=w448) -> ("error out"=w446:errorcluster, "ADCValOutput Single"=w442:dbl)  [unwired: 5 in, 1 out]
                        "FullSpeed2 Current" <- w442
                        n179 = Greater Or Equal?(x=w442, y=w443) -> (x >= y?=w432:bool)
                        n180 = And(x=w435, y=w432) -> (x .and. y?=w433:bool)
                        n181 = Compound Arithmetic op=OR(w434, w436, w433) -> (w441:bool)
                        n182 = call "Write panel message (SubVI).vi"("Stop BurnIn"=w427, 4:"rpm"=w423, 5:"rpm"=TRUE ("rpm"), "PrintTime"=FALSE, "Stop"=w429, "error in (no error)"=w446, "Time to wait"=0.2, "Strin"=w426, "String in"=w430) -> ("error out"=w431:errorcluster)  [unwired: 2 in]
                      }
                      n183 = property class="Bool (strict)"(reference=w389, error in=w402) -> ("Value"=w419:bool)  [unwired: 2 out]
                      n184 = Select(t=T13."Stop", s=w419, f=T13."Result") -> (s? t:f=w416:T13)
                    }
                    frame "MD[1]=1" {
                      n185 = Concatenate Strings(w479, "\nSet Parameters MD[1]=1" ("Strin")) -> (w468:string)
                      n186 = property on="VISA Tester" class="VISAName"() -> ("Value"=w484:refnum<visa-resource-name>)  [unwired: 2 in, 2 out]
                      n187 = call "TesterOption (SubVI).vi"("2 Options"=FALSE, "On/Off"=FALSE, "Tester Option"=T12."Venable", "VISA Refnum in"=w484) -> ("error out"=w485:errorcluster, "VISA Refnum out"=w475:refnum<visa-resource-name>)  [unwired: 6 in]
                      n188 = call "CANSendMotorSpeed.vi"("Remote"=TRUE, "error in (no error)"=w485, "Motor Speed RPM"=u16 0, "UUT"=w469, "CAN Cluster in"=w490) -> ("error out"=w487:errorcluster)  [unwired: 6 in]
                      n189 = call "Write panel message (SubVI).vi"("Stop BurnIn"=w470, 4:"rpm"=w458, 5:"rpm"=FALSE ("rpm"), "PrintTime"=TRUE, "Stop"=w460, "error in (no error)"=w487, "Time to wait"=20.0, "Strin"=w468, "String in"=w471) -> ("error out"=w457:errorcluster)  [unwired: 2 in]
                      n190 = property on="VISA Marvin" class="VISAName"(error in=w457) -> (error out=w486:errorcluster, "Value"=w492:refnum<visa-resource-name>)  [unwired: 1 in, 1 out]
                      n191 = call "SerialMarvinSendGet.vi"("error in (no error)"=w486, "Clear Log"=FALSE, "write buffer"="EP=1\r\nMD[1]=1\r\n", "VISA resource name"=w492) -> ("error out"=w474:errorcluster)  [unwired: 6 in, 1 out]
                      n192 = call "TesterOption (SubVI).vi"("2 Options"=FALSE, "error in (no error)"=w474, "On/Off"=FALSE, "Tester Option"=T12."Power", "VISA Refnum in"=w475) -> ("error out"=w472:errorcluster, "VISA Refnum out"=w461:refnum<visa-resource-name>)  [unwired: 5 in]
                      n193 = call "Write panel message (SubVI).vi"("Stop BurnIn"=w470, 4:"rpm"=w458, 5:"rpm"=FALSE ("rpm"), "PrintTime"=TRUE, "Stop"=w460, "error in (no error)"=w472, "Time to wait"=25.0, "Strin"=w468, "String in"=w471) -> ("error out"=w462:errorcluster)  [unwired: 2 in]
                      n194 = call "TesterOption (SubVI).vi"("2 Options"=FALSE, "error in (no error)"=w462, "On/Off"=TRUE, "Tester Option"=T12."Venable", "VISA Refnum in"=w461) -> ("error out"=w459:errorcluster)  [unwired: 5 in, 1 out]
                      n195 = call "Time Delay8"("error in (no error)"=w459) -> ("error out"=w455:errorcluster)  [unwired: 10 in]
                      n196 = property class="Bool (strict)"(reference=w460, error in=w455) -> ("Value"=w497:bool)  [unwired: 2 out]
                      n197 = Select(t=T13."Stop", s=w497, f=T13."FullSpeed2") -> (s? t:f=w496:T13)
                    }
                    frame "FullSpeed1" {
                      n198 = Concatenate Strings(w517, "\nFull speed operation " ("string")) -> (w502:string)
                      n199 = Equal?(x=w498, y=u8 95) -> (x = y?=w515:bool)
                      n200 = flat-sequence {
                        tunnel: w508 -> [w534]
                        tunnel: [w534] -> w507
                        tunnel: [w533] -> w506
                        frame #0 {
                          n201 = call <vilib>:"High Resolution Relative Seconds.vi"() -> ("relative seconds"=w533:dbl)
                        }
                      }
                      n202 = Select(t=u16 15100, s=w515, f=u16 12100 ("y")) -> (s? t:f=w522:u16)
                      n203 = call "CANSendMotorSpeed.vi"("Remote"=TRUE, "Motor Speed RPM"=w522, "UUT"=w523, "CAN Cluster in"=w527) -> ("error out"=w520:errorcluster)  [unwired: 7 in]
                      n204 = call "Write panel message (SubVI).vi"("Stop BurnIn"=w503, 4:"rpm"=w519, 5:"rpm"=TRUE ("rpm"), "PrintTime"=FALSE, "Stop"=w505, "error in (no error)"=w520, "Time to wait"=0.2, "Strin"=w502, "String in"=w504) -> ("error out"=w508:errorcluster)  [unwired: 2 in]
                      n205 = Select(t=13700.0, s=w515, f=11500.0) -> (s? t:f=w510:dbl)
                      n206 = Select(t=56.0, s=w515, f=33.0) -> (s? t:f=w509:dbl)
                      n207 = while {
                        tunnel: w519 -> [w536]
                        tunnel: w507 -> [w564]
                        tunnel: [w544] -> w518
                        tunnel: w510 -> [w556]
                        tunnel: w509 -> [w553]
                        tunnel: w506 -> [w551]
                        tunnel: w505 -> [w542]
                        tunnel: w504 -> [w543]
                        tunnel: w503 -> [w540]
                        tunnel: w502 -> [w539]
                        stop <- w558 stop-if-true
                        n208 = property class="DigNum (strict)"(reference=w536, error in=w564) -> (error out=w563:errorcluster, "Value"=w557:dbl)  [unwired: 1 out]
                        "FullSpeed1 Speed" <- w557
                        n209 = call <vilib>:"High Resolution Relative Seconds.vi"() -> ("relative seconds"=w552:dbl)
                        n210 = Subtract(x=w552, y=w551) -> (x-y=w550:dbl)
                        n211 = Greater Or Equal?(x=w550, y=120.0) -> (x >= y?=w548:bool)
                        n212 = Greater Or Equal?(x=w557, y=w556) -> (x >= y?=w555:bool)
                        n213 = property on="VISA Tester" class="VISAName"(error in=w563) -> (error out=w562:errorcluster, "Value"=w561:refnum<visa-resource-name>)  [unwired: 1 in, 1 out]
                        n214 = call "GetADCTester (SubVI).vi"("error in (no error)"=w562, "GetADCTester"=T14."Current", "TimeToGet"=5, "VISA Refnum in"=w561) -> ("error out"=w559:errorcluster, "ADCValOutput Single"=w554:dbl)  [unwired: 5 in, 1 out]
                        "FullSpeed1 Current" <- w554
                        n215 = Greater Or Equal?(x=w554, y=w553) -> (x >= y?=w545:bool)
                        n216 = And(x=w545, y=w555) -> (x .and. y?=w546:bool)
                        n217 = property class="Bool (strict)"(reference=w542) -> ("Value"=w547:bool)  [unwired: 1 in, 2 out]
                        n218 = call "Write panel message (SubVI).vi"("Stop BurnIn"=w540, 4:"rpm"=w536, 5:"rpm"=TRUE ("rpm"), "PrintTime"=FALSE, "Stop"=w542, "error in (no error)"=w559, "Time to wait"=0.2, "Strin"=w539, "String in"=w543) -> ("error out"=w544:errorcluster)  [unwired: 2 in]
                        n219 = Compound Arithmetic op=OR(w547, w546, w548) -> (w558:bool)
                      }
                      n220 = property class="Bool (strict)"(reference=w505, error in=w518) -> ("Value"=w532:bool)  [unwired: 2 out]
                      n221 = Select(t=T13."Stop", s=w532, f=T13."MD[1]=1") -> (s? t:f=w529:T13)
                    }
                    frame "MD[1]=0" {
                      n222 = Concatenate Strings(w591, "\nSet Parameters MD[1]=0" ("Strin")) -> (w580:string)
                      n223 = property on="VISA Tester" class="VISAName"() -> ("Value"=w597:refnum<visa-resource-name>)  [unwired: 2 in, 2 out]
                      n224 = call "TesterOption (SubVI).vi"("2 Options"=FALSE, "On/Off"=FALSE, "Tester Option"=T12."Venable", "VISA Refnum in"=w597) -> ("error out"=w598:errorcluster, "VISA Refnum out"=w587:refnum<visa-resource-name>)  [unwired: 6 in]
                      n225 = call "CANSendMotorSpeed.vi"("Remote"=TRUE, "error in (no error)"=w598, "Motor Speed RPM"=u16 0, "UUT"=w581, "CAN Cluster in"=w603) -> ("error out"=w600:errorcluster)  [unwired: 6 in]
                      n226 = call "Write panel message (SubVI).vi"("Stop BurnIn"=w582, 4:"rpm"=w577, 5:"rpm"=FALSE ("rpm"), "PrintTime"=FALSE, "Stop"=w571, "error in (no error)"=w600, "Time to wait"=0.2, "Strin"=w580, "String in"=w583) -> ("error out"=w594:errorcluster)  [unwired: 2 in]
                      n227 = property on="VISA Marvin" class="VISAName"(error in=w594) -> (error out=w599:errorcluster, "Value"=w605:refnum<visa-resource-name>)  [unwired: 1 in, 1 out]
                      n228 = call "SerialMarvinSendGet.vi"("error in (no error)"=w599, "Clear Log"=FALSE, "write buffer"="EP=1\r\nMD[1]=0\r\n", "VISA resource name"=w605) -> ("error out"=w586:errorcluster)  [unwired: 6 in, 1 out]
                      n229 = call "TesterOption (SubVI).vi"("2 Options"=FALSE, "error in (no error)"=w586, "On/Off"=FALSE, "Tester Option"=T12."Power", "VISA Refnum in"=w587) -> ("error out"=w584:errorcluster, "VISA Refnum out"=w572:refnum<visa-resource-name>)  [unwired: 5 in]
                      n230 = call "Write panel message (SubVI).vi"("Stop BurnIn"=w582, 4:"rpm"=w577, 5:"rpm"=FALSE ("rpm"), "PrintTime"=TRUE, "Stop"=w571, "error in (no error)"=w584, "Time to wait"=25.0, "Strin"=w580, "String in"=w583) -> ("error out"=w573:errorcluster)  [unwired: 2 in]
                      n231 = call "TesterOption (SubVI).vi"("2 Options"=FALSE, "error in (no error)"=w573, "On/Off"=TRUE, "Tester Option"=T12."Venable", "VISA Refnum in"=w572) -> ("error out"=w570:errorcluster)  [unwired: 5 in, 1 out]
                      n232 = call "Time Delay4"("error in (no error)"=w570) -> ("error out"=w566:errorcluster)  [unwired: 10 in]
                      n233 = property class="Bool (strict)"(reference=w571, error in=w566) -> ("Value"=w610:bool)  [unwired: 2 out]
                      n234 = Select(t=T13."Stop", s=w610, f=T13."FullSpeed1") -> (s? t:f=w609:T13)
                    }
                  }
                }
                n235 = flat-sequence {
                  tunnel: [enum16{"Stop", "Direction", "Venable", "Start"}."Stop"] -> w329
                  tunnel: w328 -> [_]
                  frame #0 {
                  }
                }
              }
              frame "Venable" {
                n236 = call "Find_Number_LineMARVIN from number.vi"("Test Paragraph"="4.1", "TableIn"=w614) -> ("Line number"=w622:i32)  [unwired: 3 in, 3 out]
                n237 = for {
                  tunnel: u16[] [5000, 0, 5000] -> [w652] mode=indexing
                  tunnel: bool[] [TRUE, FALSE, TRUE] -> [w647] mode=indexing
                  tunnel: w622 -> [w653]
                  tunnel: w621 -> [w651]
                  tunnel: w620 -> [w650]
                  tunnel: w619 -> [w638]
                  tunnel: w618 -> [w642]
                  tunnel: w616 -> [w641]
                  tunnel: w617 -> [w640]
                  tunnel: w614 -> [w634]
                  tunnel: w613 -> [w632]
                  tunnel: [w631] -> w612 mode=indexing
                  i -> [w654]
                  w656 = 200.0 ("y")
                  n238 = call "CANSendMotorSpeed.vi"("Remote"=TRUE, "Motor Speed RPM"=u16 5000, "UUT"=w650, "CAN Cluster in"=w651) -> ("error out"=w646:errorcluster)  [unwired: 7 in]
                  n239 = property on="VISA Tester" class="VISAName"() -> ("Value"=w645:refnum<visa-resource-name>)  [unwired: 2 in, 2 out]
                  n240 = Add(x=w653, y=w654) -> (x+y=w635:i32)
                  n241 = call "TesterOption (SubVI).vi"("2 Options"=FALSE, "error in (no error)"=w646, "On/Off"=w647, "Tester Option"=T12."Venable", "VISA Refnum in"=w645) -> ("error out"=w644:errorcluster)  [unwired: 5 in, 1 out]
                  n242 = call "Write panel message (SubVI).vi"("Stop BurnIn"=w640, 4:"rpm"=w638, 5:"rpm"=TRUE ("rpm"), "PrintTime"=TRUE, "Stop"=w641, "error in (no error)"=w644, "Time to wait"=15.0, "Strin"=w632, "String in"=w642) -> ("error out"=w643:errorcluster)  [unwired: 2 in]
                  n243 = property class="DigNum (strict)"(reference=w638, error in=w643) -> ("Value"=w633:dbl)  [unwired: 2 out]
                  n244 = Add(x=w652, y=w656) -> (x+y=w658:dbl)
                  n245 = Subtract(x=w652, y=w656) -> (x-y=w657:dbl)
                  n246 = In Range and Coerce(upper limit=w658, x=w633, lower limit=w657) -> (In Range?=w631:bool)  [unwired: 1 out]
                  n247 = call "PassOrFail (SubVI).vi"("index (row)"=w635, "Data in"=w633, "Pass?Fail"=w631, "Table in"=w634) -> ()  [unwired: 7 in, 1 out]
                }
                n248 = property class="Bool (strict)"(reference=w616) -> ("Value"=w629:bool)  [unwired: 1 in, 2 out]
                n249 = And Array Elements(Boolean array=w612) -> (logical AND=→"VenableResult":bool)
                n250 = Select(t=enum16{"Stop", "Direction", "Venable", "Start"}."Stop", s=w629, f=enum16{"Stop", "Direction", "Venable", "Start"}."Direction") -> (s? t:f=w615:enum16{"Stop", "Direction", "Venable", "Start"})
              }
              frame "Start" {
                w678 = "4" ("Test Paragraph")
                n251 = property class="Str"(reference=w670, "Value"=w661) -> (reference out=w679:refnum<vi>, error out=w667:errorcluster)  [unwired: 1 in]
                n252 = call "Table_ScrollaBarMarvin.vi"("error in"=w667, "Line to focus"=w678, "TableIn"=w659) -> ("error out"=w675:errorcluster)  [unwired: 1 in, 2 out]
                n253 = call "Reset old test Values (SubVI) from number.vi"("error in"=w675, "Atr in"=w659, "Test Paragraph"=w678) -> ("error out"=w674:errorcluster)  [unwired: 8 in]
                n254 = property on="VISA Tester" class="VISAName"(error in=w674) -> (error out=w673:errorcluster, "Value"=w672:refnum<visa-resource-name>)  [unwired: 1 in, 1 out]
                n255 = property class="Bool (strict)"(reference=w664) -> ("Value"=w683:bool)  [unwired: 1 in, 2 out]
                n256 = call "TesterOption (SubVI).vi"("2 Options"=FALSE, "error in (no error)"=w673, "On/Off"=TRUE, "Tester Option"=T12."Venable", "VISA Refnum in"=w672) -> ("error out"=w671:errorcluster)  [unwired: 5 in, 1 out]
                n257 = Select(t=enum16{"Stop", "Direction", "Venable", "Start"}."Stop", s=w683, f=enum16{"Stop", "Direction", "Venable", "Start"}."Venable") -> (s? t:f=w668:enum16{"Stop", "Direction", "Venable", "Start"})
                n258 = call "Write panel message (SubVI).vi"("Stop BurnIn"=w663, 4:"rpm"=w662, 5:"rpm"=FALSE ("rpm"), "PrintTime"=FALSE, "Stop"=w664, "error in (no error)"=w671, "Time to wait"=0.2, "Strin"=w661, "String in"=w679) -> ()  [unwired: 2 in, 1 out]
              }
            }
          }
        }
        frame "Speed Command" {
          w688 = "5. Speed Command Test in process..." ("Value")
          w685 = "5" ("Test Paragraph")
          n259 = control-ref of="Pannel User Message"() -> (w700:refnum<vi>)
          n260 = property class="Str"(reference=w700, error in=w699, "Value"=w688) -> (error out=w698:errorcluster)  [unwired: 1 out]
          n261 = call "Table_ScrollaBarMarvin.vi"("error in"=w698, "Line to focus"=w685, "TableIn"=w684) -> ("error out"=w701:errorcluster)  [unwired: 1 in, 2 out]
          n262 = property class="Tbl (strict)"(reference=w684, error in=w701) -> (error out=w703:errorcluster, "Value"=w704:string[][])  [unwired: 1 out]
          n263 = Index Array(array=w704, index (col)=0 ("disabled index (col)")) -> (element=w705:string[])  [unwired: 1 in]
          n264 = call "Find_Number_LineMARVIN from number.vi"("Test Paragraph"=w685, "error in"=w703, "TableIn"=w684, "Row Headers[]"=w705) -> ("error out"=w686:errorcluster, "Line number"=w689:i32)  [unwired: 1 in, 2 out]
          n265 = call "Reset old test Values (SubVI) from number.vi"("error in"=w686, "Atr in"=w684, "Test Paragraph"=w685) -> ()  [unwired: 8 in, 1 out]
          n266 = control-ref of="Pannel User Message"() -> (w693:refnum<vi>)
          n267 = control-ref of="Stop Burn-in"() -> (w697:refnum<vi>)
          n268 = control-ref of="Config_CANAT"() -> (w694:refnum<vi>)
          n269 = control-ref of="Motor Speed RPM"() -> (w695:refnum<vi>)
          n270 = control-ref of="UUT"() -> (w696:refnum<vi>)
          n271 = control-ref of="Stop Button"() -> (w691:refnum<vi>)
          n272 = control-ref of="ATR"() -> (w692:refnum<vi>)
          n273 = property on="UUT" class="DigNum (strict)"() -> ("Value"=w687:u8)  [unwired: 2 in, 2 out]
          n274 = while {
            shift-right: [w717] -> _
            shift-left: enum16{"Stop", "StopTime", "Speeds", "Start"}."Start" -> [w718]
            tunnel: w691 -> [w716]
            tunnel: w692 -> [w715]
            tunnel: w693 -> [w714]
            tunnel: w694 -> [w713]
            tunnel: w695 -> [w712]
            tunnel: w696 -> [w711]
            tunnel: w697 -> [w710]
            tunnel: w689 -> [w709]
            tunnel: w688 -> [w708]
            tunnel: w687 -> [w706]
            stop <- w707 stop-if-true
            n275 = case shown="\"StopTime\"" w718 {
              tunnel: [w722 w751 w792 w836] -> w717
              tunnel: w716 -> [_ w746 w796 w834]
              tunnel: w715 -> [_ w734 w800 _]
              tunnel: w714 -> [_ w747 w797 _]
              tunnel: w713 -> [w720 w749 w799 _]
              tunnel: w712 -> [_ w744 w794 _]
              tunnel: w711 -> [w721 w748 w791 _]
              tunnel: w710 -> [_ w745 w795 _]
              tunnel: w709 -> [_ _ w801 _]
              tunnel: w708 -> [_ _ w798 _]
              tunnel: [w719 w750 w793 FALSE ("Value")] -> w707
              tunnel: w706 -> [_ _ w784 _]
              frame "Stop", Default {
                n276 = flat-sequence {
                  tunnel: w721 -> [w725]
                  tunnel: w720 -> [w724]
                  tunnel: [enum16{"Stop", "StopTime", "Speeds", "Start"}."Stop"] -> w722
                  tunnel: [TRUE] -> w719
                  frame #0 {
                    n277 = call "CANSendMotorSpeed.vi"("Remote"=TRUE, "Motor Speed RPM"=u16 0, "UUT"=w725, "CAN Cluster in"=w724) -> ("error out"=w730:errorcluster)  [unwired: 7 in]
                    n278 = property on="VISA Tester" class="VISAName"() -> ("Value"=w731:refnum<visa-resource-name>)  [unwired: 2 in, 2 out]
                    n279 = call "TesterOption (SubVI).vi"("2 Options"=FALSE, "error in (no error)"=w730, "On/Off"=FALSE, "Tester Option"=T12."Venable", "VISA Refnum in"=w731) -> ()  [unwired: 5 in, 2 out]
                  }
                  frame #1 {
                  }
                }
              }
              frame "StopTime" {
                n280 = call "Table_ScrollaBarMarvin.vi"("Line to focus"="6", "TableIn"=w734) -> ("error out"=w737:errorcluster)  [unwired: 2 in, 2 out]
                n281 = call "CANSendMotorSpeed.vi"("Remote"=TRUE, "error in (no error)"=w737, "Motor Speed RPM"=u16 0, "UUT"=w748, "CAN Cluster in"=w749) -> ("error out"=w755:errorcluster)  [unwired: 6 in]
                n282 = flat-sequence {
                  tunnel: [w781] -> w754
                  tunnel: w755 -> [w780]
                  tunnel: [w780] -> w756
                  frame #0 {
                    n283 = call <vilib>:"High Resolution Relative Seconds.vi"() -> ("relative seconds"=w781:dbl)
                  }
                }
                n284 = while {
                  tunnel: [w776] -> w750
                  tunnel: w747 -> [w774]
                  tunnel: w746 -> [w773]
                  tunnel: w745 -> [w771]
                  tunnel: w744 -> [w770]
                  tunnel: "6. Stop Time Test in process..." ("Value") -> [w758]
                  tunnel: [w766] -> w735
                  tunnel: w756 -> [w778]
                  tunnel: [w767] -> w742
                  tunnel: w754 -> [w777]
                  tunnel: [w765] -> w738
                  stop <- w757 stop-if-true
                  n285 = call "Write panel message (SubVI).vi"("Stop BurnIn"=w771, 4:"rpm"=w770, 5:"rpm"=TRUE ("rpm"), "PrintTime"=FALSE, "Stop"=w773, "error in (no error)"=w778, "Time to wait"=0.1, "Strin"=w758, "String in"=w774) -> ("error out"=w775:errorcluster)  [unwired: 2 in]
                  n286 = control-ref of="Motor Speed RPM"() -> (w764:refnum<vi>)
                  n287 = property class="DigNum (strict)"(reference=w764, error in=w775) -> (error out=w767:errorcluster, "Value"=w763:dbl)  [unwired: 1 out]
                  n288 = call <vilib>:"High Resolution Relative Seconds.vi"() -> ("relative seconds"=w761:dbl)
                  n289 = property class="Bool (strict)"(reference=w773) -> ("Value"=w776:bool)  [unwired: 1 in, 2 out]
                  n290 = Subtract(x=w761, y=w777) -> (x-y=w765:dbl)
                  n291 = Greater Or Equal?(x=w765, y=50.0) -> (x >= y?=w759:bool)
                  n292 = Less Or Equal?(x=w763, y=0.0) -> (x <= y?=w766:bool)
                  n293 = Compound Arithmetic op=OR(w766, w759, w776) -> (w757:bool)
                }
                "StopTimeResult" <- w735
                n294 = call "Find_Number_LineMARVIN from number.vi"("Test Paragraph"="6", "TableIn"=w734) -> ("Line number"=w739:i32)  [unwired: 3 in, 3 out]
                n295 = call "PassOrFail (SubVI).vi"("index (row)"=w739, "error in (no error)"=w742, "Data in"=w738, "Pass?Fail"=w735, "Table in"=w734) -> ("error out"=w741:errorcluster)  [unwired: 6 in]
                n296 = flat-sequence {
                  tunnel: [enum16{"Stop", "StopTime", "Speeds", "Start"}."Stop"] -> w751
                  tunnel: w741 -> [_]
                  frame #0 {
                  }
                }
              }
              frame "Speeds" {
                n297 = Equal?(x=w784, y=u8 95) -> (x = y?=w789:bool)
                n298 = Select(t=u16[] [6000, 11500, 15100], s=w789, f=u16[] [6000, 9000, 12100]) -> (s? t:f=w786:u16[])
                n299 = for {
                  tunnel: w786 -> [w827] mode=indexing
                  tunnel: w801 -> [w820]
                  tunnel: w800 -> [w819]
                  tunnel: w791 -> [w818]
                  tunnel: w799 -> [w817]
                  tunnel: w798 -> [w816]
                  tunnel: w797 -> [w815]
                  tunnel: w796 -> [w814]
                  tunnel: w795 -> [w812]
                  tunnel: w794 -> [w810]
                  tunnel: [w808] -> w793
                  tunnel: [w807] -> w785
                  tunnel: [w806] -> w783 mode=indexing
                  i -> [w826]
                  stop <- w808 stop-if-true
                  w828 = 200.0 ("y")
                  n300 = Increment(x=w826) -> (x+1=w825:i32)
                  n301 = Add(x=w820, y=w825) -> (x+y=w821:i32)
                  n302 = call "CANSendMotorSpeed.vi"("Remote"=TRUE, "Motor Speed RPM"=w827, "UUT"=w818, "CAN Cluster in"=w817) -> ("error out"=w832:errorcluster)  [unwired: 7 in]
                  n303 = control-ref of="Motor Speed RPM"() -> (w833:refnum<vi>)
                  n304 = call "Write panel message (SubVI).vi"("Stop BurnIn"=w812, 4:"rpm"=w810, 5:"rpm"=TRUE ("rpm"), "PrintTime"=TRUE, "Stop"=w814, "error in (no error)"=w832, "Time to wait"=25.0 ("Delay Time (sec)"), "Strin"=w816, "String in"=w815) -> ("error out"=w824:errorcluster)  [unwired: 2 in]
                  n305 = property class="DigNum (strict)"(reference=w833, error in=w824) -> (error out=w831:errorcluster, "Value"=w809:dbl)  [unwired: 1 out]
                  n306 = property class="Bool (strict)"(reference=w814) -> ("Value"=w808:bool)  [unwired: 1 in, 2 out]
                  n307 = Add(x=w827, y=w828) -> (x+y=w830:dbl)
                  n308 = Subtract(x=w827, y=w828) -> (x-y=w829:dbl)
                  n309 = In Range and Coerce(upper limit=w830, x=w809, lower limit=w829) -> (In Range?=w806:bool)  [unwired: 1 out]
                  n310 = call "PassOrFail (SubVI).vi"("index (row)"=w821, "error in (no error)"=w831, "Data in"=w809, "Pass?Fail"=w806, "Table in"=w819) -> ("error out"=w807:errorcluster)  [unwired: 6 in]
                }
                n311 = flat-sequence {
                  tunnel: w793 -> [w805]
                  tunnel: [w803] -> w792
                  tunnel: w785 -> [_]
                  frame #0 {
                    n312 = Select(t=enum16{"Stop", "StopTime", "Speeds", "Start"}."Stop", s=w805, f=enum16{"Stop", "StopTime", "Speeds", "Start"}."StopTime") -> (s? t:f=w803:enum16{"Stop", "StopTime", "Speeds", "Start"})
                  }
                }
                n313 = And Array Elements(Boolean array=w783) -> (logical AND=→"SpeedResult":bool)
              }
              frame "Start" {
                n314 = property on="VISA Tester" class="VISAName"() -> ("Value"=w844:refnum<visa-resource-name>)  [unwired: 2 in, 2 out]
                n315 = call "TesterOption (SubVI).vi"("2 Options"=FALSE, "On/Off"=TRUE, "Tester Option"=T12."Venable", "VISA Refnum in"=w844) -> ("error out"=w835:errorcluster)  [unwired: 6 in, 1 out]
                n316 = property class="Bool (strict)"(reference=w834, error in=w835) -> ("Value"=w840:bool)  [unwired: 2 out]
                n317 = Select(t=enum16{"Stop", "StopTime", "Speeds", "Start"}."Stop", s=w840, f=enum16{"Stop", "StopTime", "Speeds", "Start"}."Speeds") -> (s? t:f=w836:enum16{"Stop", "StopTime", "Speeds", "Start"})
              }
            }
          }
        }
        frame "Stop Time" {
          w848 = "3. Motor Temperature test in process..." ("Value")
          w846 = "3" ("Test Paragraph")
          n318 = control-ref of="Pannel User Message"() -> (w856:refnum<vi>)
          n319 = property class="Str"(reference=w856, error in=w855, "Value"=w848) -> (error out=w854:errorcluster)  [unwired: 1 out]
          n320 = call "Table_ScrollaBarMarvin.vi"("error in"=w854, "Line to focus"=w846, "TableIn"=w845) -> ("error out"=w858:errorcluster)  [unwired: 1 in, 2 out]
          n321 = property class="Tbl (strict)"(reference=w845, error in=w858) -> (reference out=w851:refnum<vi>, error out=w860:errorcluster, "Value"=w861:string[][])
          n322 = Index Array(array=w861, index (col)=0 ("disabled index (col)")) -> (element=w862:string[])  [unwired: 1 in]
          n323 = call "Find_Number_LineMARVIN from number.vi"("Test Paragraph"=w846, "error in"=w860, "TableIn"=w845, "Row Headers[]"=w862) -> ("error out"=w857:errorcluster, "Line number"=w850:i32)  [unwired: 1 in, 2 out]
          n324 = call "Reset old test Values (SubVI) from number.vi"("error in"=w857, "Atr in"=w845, "Test Paragraph"=w846) -> ("error out"=w847:errorcluster)  [unwired: 8 in]
          n325 = property on="Status" class="Bool (strict)"(error in=w847) -> (error out=w852:errorcluster, "Value"=w853:bool)  [unwired: 1 in, 1 out]
          n326 = case shown="True" w853 {
            selector: w853 -> [w866 _]
            tunnel: w852 -> [w868 _]
            tunnel: w851 -> [w865 _]
            tunnel: w850 -> [w864 w871]
            tunnel: w849 -> [_ w876]
            tunnel: w848 -> [_ w872]
            frame False {
              n327 = flat-sequence {
                tunnel: w868 -> [w869]
                tunnel: [w869] -> w867
                frame #0 {
                  n328 = One Button Dialog(message="Please establish RS connection.") -> ()  [unwired: 1 in, 1 out]
                }
              }
              n329 = Increment(x=w864) -> (x+1=w863:i32)
              n330 = call "PassOrFail (SubVI).vi"("index (row)"=w863, "error in (no error)"=w867, "Pass?Fail"=w866, "Table in"=w865) -> ()  [unwired: 7 in, 1 out]
            }
            frame True {
              n331 = control-ref of="Stop Burn-in"() -> (w878:refnum<vi>)
              n332 = control-ref of="Pannel User Message"() -> (w880:refnum<vi>)
              n333 = control-ref of="Config_CANAT"() -> (w874:refnum<vi>)
              n334 = control-ref of="ATR"() -> (w881:refnum<vi>)
              n335 = control-ref of="Motor Speed RPM"() -> (w882:refnum<vi>)
              n336 = control-ref of="UUT"() -> (w873:refnum<vi>)
              n337 = control-ref of="Stop Button"() -> (w879:refnum<vi>)
              n338 = property on="VISA Tester" class="VISAName"() -> ("Value"=w875:refnum<visa-resource-name>)  [unwired: 2 in, 2 out]
              n339 = while {
                shift-right: [w886] -> _
                shift-left: T15."Start" -> [w896]
                tunnel: w878 -> [w895]
                tunnel: w879 -> [w894]
                tunnel: w880 -> [w893]
                tunnel: w881 -> [w892]
                tunnel: w882 -> [w891]
                tunnel: w876 -> [w890]
                tunnel: w875 -> [w889]
                tunnel: w874 -> [w888]
                tunnel: w873 -> [w887]
                tunnel: w872 -> [w884]
                tunnel: w871 -> [w883]
                stop <- w885 stop-if-true
                n340 = case shown="\"Start\"" w896 {
                  tunnel: w895 -> [_ w919 w978]
                  tunnel: w894 -> [_ w911 w980]
                  tunnel: w893 -> [_ w920 w982]
                  tunnel: w892 -> [_ w909 _]
                  tunnel: w891 -> [_ w918 w977]
                  tunnel: w890 -> [_ w923 _]
                  tunnel: w889 -> [w899 w922 w971]
                  tunnel: w888 -> [_ _ w988]
                  tunnel: w887 -> [_ _ w987]
                  tunnel: [w897 w912 w973] -> w886
                  tunnel: [w898 FALSE FALSE] -> w885
                  tunnel: w884 -> [_ w921 _]
                  tunnel: w883 -> [_ w908 _]
                  frame "Stop", Default {
                    n341 = flat-sequence {
                      tunnel: w899 -> [w900]
                      tunnel: [TRUE] -> w898
                      tunnel: [T15."Stop"] -> w897
                      frame #0 {
                        n342 = call "TesterOption (SubVI).vi"("2 Options"=FALSE, "On/Off"=FALSE, "Tester Option"=T12."Venable", "VISA Refnum in"=w900) -> ()  [unwired: 6 in, 2 out]
                      }
                      frame #1 {
                      }
                    }
                  }
                  frame "TA[5]" {
                    w924 = T18 [enum."60C", enum."90C", enum."120C"] items=["K15", "K16", "K17", "Venable", "Firmeware", "Fan", "Power", "120C", "110C", "100C", "90C", "80C", "70C", "60C", "50C", "40C", "30C", "25C", "20C", "10C", "0C"]
                    n343 = for {
                      tunnel: w924 -> [w948] mode=indexing
                      tunnel: w923 -> [w947]
                      tunnel: w922 -> [w946]
                      tunnel: w921 -> [w945]
                      tunnel: w920 -> [w944]
                      tunnel: w911 -> [w943]
                      tunnel: w919 -> [w942]
                      tunnel: w918 -> [w941]
                      tunnel: dbl[] [60.0, 90.0, 120.0] -> [w931] mode=indexing
                      tunnel: [w930] -> w910
                      tunnel: w909 -> [w937]
                      tunnel: w908 -> [w936]
                      tunnel: [w925] -> w907 mode=indexing
                      i -> [w934]
                      w929 = 3.0 ("y")
                      n344 = for {
                        N: 5 -> [_]
                        tunnel: w948 -> [w950]
                        tunnel: w947 -> [w966]
                        tunnel: w946 -> [w962]
                        tunnel: w945 -> [w960]
                        tunnel: w944 -> [w959]
                        tunnel: w943 -> [w958]
                        tunnel: w942 -> [w956]
                        tunnel: w941 -> [w953]
                        tunnel: [w952] -> w940 mode=indexing
                        tunnel: [w951] -> w938
                        n345 = call "TesterOption (SubVI).vi"("2 Options"=FALSE, "On/Off"=TRUE, "Tester Option"=w950, "VISA Refnum in"=w962) -> ("error out"=w963:errorcluster)  [unwired: 6 in, 1 out]
                        n346 = call "Write panel message (SubVI).vi"("Stop BurnIn"=w956, 4:"rpm"=w953, 5:"rpm"=FALSE ("rpm"), "PrintTime"=FALSE, "Stop"=w958, "error in (no error)"=w963, "Time to wait"=1.0, "Strin"=w960, "String in"=w959) -> ("error out"=w961:errorcluster)  [unwired: 2 in]
                        n347 = call "SerialMarvinSendGet.vi"("error in (no error)"=w961, "write buffer"="TA[2]\r\n", "VISA resource name"=w966) -> ("error out"=w951:errorcluster, "read buffer"=w964:string)  [unwired: 7 in]
                        n348 = Fract/Exp String To Number(string=w964) -> (number=w952:dbl)  [unwired: 3 in, 1 out]
                      }
                      n349 = Increment(x=w934) -> (x+1=w933:i32)
                      n350 = Add Array Elements(numeric array=w940) -> (sum=w939:dbl)
                      n351 = Add(x=w931, y=w929) -> (x+y=w928:dbl)
                      n352 = Subtract(x=w931, y=w929) -> (x-y=w927:dbl)
                      n353 = Divide(x=w939, y=5.0) -> (x/y=w926:dbl)
                      n354 = In Range and Coerce(upper limit=w928, x=w926, lower limit=w927) -> (In Range?=w925:bool)  [unwired: 1 out]
                      n355 = Add(x=w936, y=w933) -> (x+y=w935:i32)
                      n356 = call "PassOrFail (SubVI).vi"("index (row)"=w935, "error in (no error)"=w938, "Data in"=w926, "Pass?Fail"=w925, "Table in"=w937) -> ("error out"=w930:errorcluster)  [unwired: 6 in]
                    }
                    n357 = property class="Bool (strict)"(reference=w911, error in=w910) -> ("Value"=w916:bool)  [unwired: 2 out]
                    n358 = Select(t=T15."Stop", s=w916, f=T15."Stop") -> (s? t:f=w912:T15)
                    n359 = And Array Elements(Boolean array=w907) -> (logical AND=→"MotorTempResult":bool)
                  }
                  frame "Start" {
                    n360 = call "Write panel message (SubVI).vi"("Stop BurnIn"=w978, 4:"rpm"=w977, 5:"rpm"=FALSE ("rpm"), "PrintTime"=FALSE, "Stop"=w980, "Time to wait"=0.1, "Strin"="3. Motor Temperature test in process...\nInitialization state...", "String in"=w982) -> ("error out"=w983:errorcluster)  [unwired: 3 in]
                    n361 = call "TesterOption (SubVI).vi"("2 Options"=FALSE, "error in (no error)"=w983, "On/Off"=FALSE, "Tester Option"=T12."Venable", "VISA Refnum in"=w971) -> ("error out"=w985:errorcluster)  [unwired: 5 in, 1 out]
                    n362 = call "CANSendMotorSpeed.vi"("Remote"=TRUE, "error in (no error)"=w985, "Motor Speed RPM"=u16 0, "UUT"=w987, "CAN Cluster in"=w988) -> ("error out"=w970:errorcluster)  [unwired: 6 in]
                    n363 = property class="Bool (strict)"(reference=w980, error in=w970) -> ("Value"=w992:bool)  [unwired: 2 out]
                    n364 = Select(t=T15."Stop", s=w992, f=T15."TA[5]") -> (s? t:f=w973:T15)
                  }
                }
              }
            }
          }
        }
        frame "Temp Control" {
          w1011 = "7. Temperature control test in process..." ("Value")
          w1009 = "7" ("Test Paragraph")
          n365 = control-ref of="Pannel User Message"() -> (w1022:refnum<vi>)
          n366 = call <vilib>:"Open Config Data.vi"("error in (no error)"=w1005, "create file if necessary (T)"=FALSE, "configuration file path"=w1007) -> ("error out"=w1008:errorcluster, "refnum"=w1004:T11)  [unwired: 7 out]
          n367 = property class="Str"(reference=w1022, error in=w1005, "Value"=w1011) -> (error out=w1021:errorcluster)  [unwired: 1 out]
          n368 = call-poly <vilib>:"Read Key.vi"("section"="Marvin", "error in (no error)"=w1008, "default value"="10", "key"="Temp Algorithm", "refnum"=w1004) -> ("error out"=w1000:errorcluster, "value"=w998:string, "refnum out"=w999:T11)  [unwired: 1 in, 3 out]
          n369 = Decimal String To Number(string=w998) -> (number=w996:i32)  [unwired: 2 in, 1 out]
          n370 = Less Or Equal To 0?(x=w996) -> (x <= 0?=w997:bool)
          n371 = Select(t=10, s=w997, f=w996) -> (s? t:f=w995:i32)
          n372 = call <vilib>:"Close Config Data.vi"("error in (no error)"=w1000, "refnum"=w999) -> ()  [unwired: 8 in, 2 out]
          n373 = control-ref of="Pannel User Message"() -> (w1016:refnum<vi>)
          n374 = control-ref of="Motor Speed RPM"() -> (w1014:refnum<vi>)
          n375 = control-ref of="Stop Button"() -> (w1018:refnum<vi>)
          n376 = control-ref of="ATR"() -> (w1017:refnum<vi>)
          n377 = control-ref of="Config_CANAT"() -> (w1015:refnum<vi>)
          n378 = control-ref of="UUT"() -> (w1013:refnum<vi>)
          n379 = control-ref of="Stop Burn-in"() -> (w1012:refnum<vi>)
          n380 = call "Table_ScrollaBarMarvin.vi"("error in"=w1021, "Line to focus"=w1009, "TableIn"=w993) -> ("error out"=w1020:errorcluster)  [unwired: 1 in, 2 out]
          n381 = call "Reset old test Values (SubVI) from number.vi"("error in"=w1020, "Atr in"=w993, "Test Paragraph"=w1009) -> ("error out"=w1010:errorcluster)  [unwired: 8 in]
          n382 = while {
            tunnel: w1010 -> [w1035]
            shift-right: [w1033] -> _
            shift-left: enum16{"Stop", "Algorithm", "Start"}."Start" -> [w1034]
            tunnel: w1018 -> [w1032]
            tunnel: w1017 -> [w1031]
            tunnel: w1016 -> [w1030]
            tunnel: w1015 -> [w1029]
            tunnel: w1014 -> [w1028]
            tunnel: w1013 -> [w1027]
            tunnel: w1012 -> [w1025]
            tunnel: w1011 -> [w1024]
            tunnel: w995 -> [w1023]
            stop <- w1026 stop-if-true
            n383 = case shown="\"Algorithm\"" w1034 {
              tunnel: w1035 -> [_ _ w1172]
              tunnel: [w1036 w1057 w1161] -> w1033
              tunnel: w1032 -> [_ w1068 w1165]
              tunnel: w1031 -> [_ w1064 _]
              tunnel: w1030 -> [_ w1069 _]
              tunnel: w1029 -> [w1039 _ w1146]
              tunnel: w1028 -> [_ w1065 _]
              tunnel: w1027 -> [w1038 _ w1145]
              tunnel: [w1037 FALSE FALSE] -> w1026
              tunnel: w1025 -> [_ w1067 _]
              tunnel: w1024 -> [_ w1066 _]
              tunnel: w1023 -> [_ w1051 _]
              frame "Stop", Default {
                n384 = flat-sequence {
                  tunnel: w1039 -> [w1044]
                  tunnel: w1038 -> [w1042]
                  tunnel: [TRUE] -> w1037
                  tunnel: [enum16{"Stop", "Algorithm", "Start"}."Stop"] -> w1036
                  frame #0 {
                    n385 = call "CANSendMotorSpeed.vi"("Remote"=TRUE, "Motor Speed RPM"=u16 0, "UUT"=w1042, "CAN Cluster in"=w1044) -> ("error out"=w1040:errorcluster)  [unwired: 7 in]
                    n386 = property on="VISA Tester" class="VISAName"() -> ("Value"=w1048:refnum<visa-resource-name>)  [unwired: 2 in, 2 out]
                    n387 = call "TesterOption (SubVI).vi"("2 Options"=FALSE, "error in (no error)"=w1040, "On/Off"=FALSE, "Tester Option"=T12."Venable", "VISA Refnum in"=w1048) -> ()  [unwired: 5 in, 2 out]
                  }
                  frame #1 {
                  }
                  frame #2 {
                  }
                }
              }
              frame "Algorithm" {
                w1052 = T19 [enum."6000", enum."11500", enum."15100", enum."11500-2", enum."6000-2"] items=["6000", "11500", "15100", "11500-2", "6000-2"]
                # "Speed Goal"
                # "Speed Ind"
                # "Temp Goal"
                # "50 Deg"
                n388 = for {
                  tunnel: w1069 -> [w1097]
                  tunnel: w1068 -> [w1096]
                  tunnel: w1067 -> [w1095]
                  tunnel: w1066 -> [w1094]
                  tunnel: w1065 -> [w1093]
                  tunnel: w1064 -> [w1080]
                  tunnel: string[] ["7.1", "7.3", "7.5", "7.7", "7.9"] -> [w1078] mode=indexing
                  shift-right: [w1090] -> _
                  shift-left: 1202.0 ("Rt") -> [w1091]
                  tunnel: dbl[] [68.0, 68.0, 88.0, 80.0, 60.0] -> [w1089] mode=indexing
                  tunnel: dbl[] [6000.0, 11500.0, 15100.0, 11500.0, 6000.0] -> [w1088] mode=indexing
                  tunnel: dbl[] [6000.0, 6400.0, 11700.0, 14600.0, 11000.0] -> [w1087] mode=indexing
                  tunnel: [w1076] -> w1058
                  tunnel: [w1075] -> w1054 mode=indexing
                  tunnel: [w1074] -> w1055 mode=indexing
                  tunnel: w1052 -> [w1073] mode=indexing
                  tunnel: w1051 -> [w1072]
                  stop <- w1092 stop-if-true
                  n389 = call <vilib>:"High Resolution Relative Seconds.vi"() -> ("relative seconds"=w1086:dbl)
                  n390 = while {
                    tunnel: w1097 -> [w1126]
                    tunnel: w1096 -> [w1118]
                    tunnel: w1095 -> [w1125]
                    tunnel: w1094 -> [w1104]
                    tunnel: w1093 -> [w1127]
                    shift-right: [w1123] -> w1090
                    shift-left: w1091 -> [w1122]
                    tunnel: w1073 -> [w1124]
                    tunnel: w1089 -> [w1121]
                    tunnel: w1088 -> [w1120]
                    tunnel: w1087 -> [w1119]
                    tunnel: w1086 -> [w1115]
                    tunnel: [w1110] -> w1081
                    tunnel: [w1109] -> w1074
                    tunnel: [w1108] -> w1079
                    tunnel: [w1107] -> w1075
                    tunnel: [w1106] -> w1077
                    tunnel: w1072 -> [w1098]
                    stop <- w1116 stop-if-true
                    n391 = call "DegToDAC (SubVI).vi"("R2"=0.0, "Rt"=w1122) -> ("error out"=w1134:errorcluster, "output array"=w1135:u8[])  [unwired: 8 in]
                    n392 = call <vilib>:"High Resolution Relative Seconds.vi"() -> ("relative seconds"=w1114:dbl)
                    n393 = property on="VISA Tester" class="VISAName"() -> ("Value"=w1137:refnum<visa-resource-name>)  [unwired: 2 in, 2 out]
                    n394 = Byte Array To String(unsigned byte array=w1135) -> (string=w1136:string)
                    n395 = Subtract(x=w1115, y=w1114) -> (x-y=w1113:dbl)
                    n396 = VISA Write(VISA resource name=w1137, write buffer=w1136, error in (no error)=w1134) -> (error out=w1133:errorcluster)  [unwired: 2 out]
                    n397 = Greater Or Equal?(x=w1113, y=120.0) -> (x >= y?=w1111:bool)
                    n398 = call <vilib>:"Clear Errors.vi"("error in (no error)"=w1133) -> ("error out"=w1132:errorcluster)  [unwired: 5 in, 1 out]
                    n399 = control-ref of="Ambient Temperature"() -> (w1105:refnum<vi>)
                    n400 = property class="DigNum (strict)"(reference=w1105) -> ("Value"=w1103:dbl)  [unwired: 1 in, 2 out]
                    n401 = property class="Bool (strict)"(reference=w1118) -> ("Value"=w1117:bool)  [unwired: 1 in, 2 out]
                    n402 = Number To Fractional String(number=w1103, precision (6)=i16 2) -> (F-format string=w1100:string)  [unwired: 2 in]
                    n403 = Concatenate Strings(w1104, "\nAmbient  Temp. [C]: " ("string"), w1100) -> (w1099:string)
                    n404 = call "Write panel message (SubVI).vi"("Stop BurnIn"=w1125, 4:"rpm"=w1127, 5:"rpm"=TRUE ("rpm"), "PrintTime"=TRUE, "Stop"=w1118, "error in (no error)"=w1132, "Time to wait"=3.0, "Strin"=w1099, "String in"=w1126) -> ("error out"=w1131:errorcluster)  [unwired: 2 in]
                    n405 = call "TempAlgoTest (SubVI).vi"("Temp"=w1105, "Speed Ind"=w1119, "Motor Speed RPM"=w1127, "Round"=w1124, "Temp Up In"=w1122, "error in (no error)"=w1131, "String in"=w1126, "Temp Goal"=w1121, "Stop"=w1118, "Speed Goal"=w1120, "Stop BurnIn"=w1125, "AD Resistor Step"=w1098, "Strin"=w1099) -> (14:"Speed Pass/Fail"=w1109:bool, "Temp  Pass/Fail"=w1108:dbl, "Temp Up Out"=w1123:dbl, 17:"Speed Pass/Fail"=w1110:dbl, "Temp Pass/Fail"=w1107:bool, "error out"=w1106:errorcluster)  [unwired: 1 in]
                    n406 = Compound Arithmetic op=OR(w1111, w1109, w1117) -> (w1116:bool)
                  }
                  n407 = property class="Bool (strict)"(reference=w1096) -> ("Value"=w1092:bool)  [unwired: 1 in, 2 out]
                  n408 = call "Find_Number_LineMARVIN from number.vi"("Test Paragraph"=w1078, "error in"=w1077, "TableIn"=w1080) -> ("error out"=w1082:errorcluster, "Line number"=w1085:i32)  [unwired: 2 in, 2 out]
                  n409 = Increment(x=w1085) -> (x+1=w1084:i32)
                  n410 = call "PassOrFail (SubVI).vi"("index (row)"=w1084, "error in (no error)"=w1082, "Data in"=w1079, "Pass?Fail"=w1075, "Table in"=w1080) -> ("error out"=w1083:errorcluster)  [unwired: 6 in]
                  n411 = call "PassOrFail (SubVI).vi"("index (row)"=w1085, "error in (no error)"=w1083, "Data in"=w1081, "Pass?Fail"=w1074, "Table in"=w1080) -> ("error out"=w1076:errorcluster)  [unwired: 6 in]
                }
                n412 = Build Array (concatenate)(w1055, w1054) -> (w1056:bool[])
                n413 = flat-sequence {
                  tunnel: w1058 -> [_]
                  tunnel: [enum16{"Stop", "Algorithm", "Start"}."Stop"] -> w1057
                  frame #0 {
                  }
                }
                n414 = And Array Elements(Boolean array=w1056) -> (logical AND=→"TempControlResult":bool)
              }
              frame "Start" {
                n415 = call <vilib>:"Clear Errors.vi"("error in (no error)"=w1172) -> ("error out"=w1147:errorcluster)  [unwired: 5 in, 1 out]
                n416 = call "CANSendMotorSpeed.vi"("Remote"=TRUE, "error in (no error)"=w1147, "Motor Speed RPM"=u16 0, "UUT"=w1145, "CAN Cluster in"=w1146) -> ("error out"=w1142:errorcluster)  [unwired: 6 in]
                n417 = call "Time Delay15"("error in (no error)"=w1142) -> ("error out"=w1141:errorcluster)  [unwired: 10 in]
                n418 = call "DegToDAC (SubVI).vi"("error in (no error)"=w1141, "R2"=0.0, "Rt"=1202.0) -> ("error out"=w1152:errorcluster, "output array"=w1153:u8[])  [unwired: 7 in]
                n419 = property on="VISA Tester" class="VISAName"() -> ("Value"=w1155:refnum<visa-resource-name>)  [unwired: 2 in, 2 out]
                n420 = Byte Array To String(unsigned byte array=w1153) -> (string=w1154:string)
                n421 = VISA Write(VISA resource name=w1155, write buffer=w1154, error in (no error)=w1152) -> (error out=w1144:errorcluster)  [unwired: 2 out]
                n422 = call "Time Delay16"("error in (no error)"=w1144) -> ("error out"=w1143:errorcluster)  [unwired: 10 in]
                n423 = property on="VISA Tester" class="VISAName"() -> ("Value"=w1171:refnum<visa-resource-name>)  [unwired: 2 in, 2 out]
                n424 = call "TesterOption (SubVI).vi"("On/Off 2"=TRUE, "Tester Option 2"=T12."Venable", "2 Options"=TRUE, "error in (no error)"=w1143, "On/Off"=TRUE, "Tester Option"=T12."K16", "VISA Refnum in"=w1171) -> ("error out"=w1157:errorcluster)  [unwired: 3 in, 1 out]
                n425 = call "Time Delay12"("error in (no error)"=w1157) -> ("error out"=w1156:errorcluster)  [unwired: 10 in]
                n426 = call "CANSendMotorSpeed.vi"("Remote"=FALSE, "error in (no error)"=w1156, "Motor Speed RPM"=u16 0, "UUT"=w1145, "CAN Cluster in"=w1146) -> ("error out"=w1140:errorcluster)  [unwired: 6 in]
                n427 = call "Time Delay17"("error in (no error)"=w1140) -> ("error out"=w1139:errorcluster)  [unwired: 10 in]
                n428 = property class="Bool (strict)"(reference=w1165, error in=w1139) -> ("Value"=w1164:bool)  [unwired: 2 out]
                n429 = Select(t=enum16{"Stop", "Algorithm", "Start"}."Stop", s=w1164, f=enum16{"Stop", "Algorithm", "Start"}."Algorithm") -> (s? t:f=w1161:enum16{"Stop", "Algorithm", "Start"})
              }
            }
          }
        }
        frame "Burn in" {
          n430 = control-ref of="Stop Button"() -> (w1177:refnum<vi>)
          n431 = control-ref of="Pannel User Message"() -> (w1180:refnum<vi>)
          n432 = control-ref of="ATR"() -> (w1176:refnum<vi>)
          n433 = control-ref of="Config_CANAT"() -> (w1179:refnum<vi>)
          n434 = control-ref of="UUT"() -> (w1178:refnum<vi>)
          n435 = control-ref of="Stop Burn-in"() -> (w1175:refnum<vi>)
          n436 = property on="UUT" class="DigNum (strict)"() -> ("Value"=w1174:u8)  [unwired: 2 in, 2 out]
          n437 = while {
            tunnel: w1180 -> [w1192]
            tunnel: w1176 -> [w1191]
            tunnel: w1179 -> [w1190]
            tunnel: w1178 -> [w1189]
            tunnel: w1177 -> [w1188]
            shift-right: [w1187] -> _
            shift-left: T16."Start" -> [w1194]
            shift-right: [w1193] -> _
            shift-left: _ -> [w1185]
            tunnel: w1175 -> [w1184]
            tunnel: w1174 -> [w1183]
            tunnel: w1173 -> [w1182]
            stop <- w1186 stop-if-true
            n438 = case shown="\"DC Current Measure\"" w1194 {
              tunnel: [w1197 w1233 w1300 w1329 w1362 w1398] -> w1193
              tunnel: w1192 -> [_ w1225 _ _ _ w1397]
              tunnel: w1191 -> [_ w1228 w1273 w1316 w1348 w1370]
              tunnel: w1190 -> [_ w1224 _ _ _ w1396]
              tunnel: w1189 -> [_ w1221 _ _ _ w1376]
              tunnel: w1188 -> [_ _ w1302 w1331 w1366 w1390]
              tunnel: [w1195 T16."Stop" w1303 w1332 w1367 w1386] -> w1187
              tunnel: [w1196 FALSE FALSE FALSE FALSE FALSE] -> w1186
              tunnel: w1185 -> [w1197 w1233 w1300 w1329 w1362 _]
              tunnel: w1184 -> [_ _ _ _ _ w1381]
              tunnel: w1183 -> [_ w1213 w1264 w1308 w1340 w1375]
              tunnel: w1182 -> [_ w1206 _ _ _ _]
              frame "Stop", Default {
                n439 = flat-sequence {
                  tunnel: [TRUE] -> w1196
                  tunnel: [T16."Stop"] -> w1195
                  frame #0 {
                    n440 = property on="VISA Tester" class="VISAName"() -> ("Value"=w1202:refnum<visa-resource-name>)  [unwired: 2 in, 2 out]
                    n441 = call "TesterOption (SubVI).vi"("2 Options"=FALSE, "On/Off"=FALSE, "Tester Option"=T12."Venable", "VISA Refnum in"=w1202) -> ("error out"=w1199:errorcluster)  [unwired: 6 in, 1 out]
                    n442 = property on="Stop Burn-in" class="Bool (strict)"(error in=w1199, "Visible"=FALSE) -> ()  [unwired: 1 in, 2 out]
                  }
                  frame #1 {
                  }
                }
              }
              frame "BurnIn" {
                w1217 = FALSE ("Stop Burn-in")
                n443 = control-ref of="Motor Speed RPM"() -> (w1227:refnum<vi>)
                n444 = control-ref of="Stop Button"() -> (w1226:refnum<vi>)
                n445 = property on="Stop Burn-in" class="Bool (strict)"("Visible"=w1206) -> (error out=w1229:errorcluster)  [unwired: 2 in, 1 out]
                n446 = Equal?(x=w1213, y=u8 95) -> (x = y?=w1210:bool)
                n447 = Select(t="8. " ("Test Paragraph"), s=w1210, f="7. " ("Test Paragraph")) -> (s? t:f=w1209:string)
                n448 = Select(t="8.4" ("Test Paragraph"), s=w1210, f="7.4" ("Test Paragraph")) -> (s? t:f=w1214:string)
                n449 = call "Find_Number_LineMARVIN from number.vi"("Test Paragraph"=w1214, "error in"=w1229, "TableIn"=w1228) -> ("error out"=w1231:errorcluster, "Line number"=w1232:i32)  [unwired: 2 in, 2 out]
                n450 = Select(t=u16 15100, s=w1210, f=u16 12100 ("y")) -> (s? t:f=w1219:u16)
                n451 = for {
                  tunnel: w1231 -> [w1252]
                  tunnel: dbl[] [600.0, 600.0, 600.0] -> [w1256] mode=indexing
                  tunnel: w1232 -> [w1261]
                  tunnel: w1228 -> [w1251]
                  tunnel: w1227 -> [w1250]
                  tunnel: w1226 -> [w1249]
                  tunnel: w1225 -> [w1248]
                  tunnel: w1224 -> [w1244]
                  tunnel: w1221 -> [w1243]
                  tunnel: w1219 -> [w1242]
                  tunnel: [w1240] -> w1218
                  tunnel: w1209 -> [w1237]
                  tunnel: [w1236] -> w1208 mode=indexing
                  i -> [w1258]
                  n452 = call "CANSendMotorSpeed.vi"("Remote"=TRUE, "error in (no error)"=w1252, "Motor Speed RPM"=w1242, "UUT"=w1243, "CAN Cluster in"=w1244) -> ("error out"=w1246:errorcluster)  [unwired: 6 in]
                  n453 = control-ref of="Stop Burn-in"() -> (w1247:refnum<vi>)
                  n454 = Concatenate Strings(w1237, "Burn-in test in process..." ("Strin")) -> (w1238:string)
                  n455 = Add(x=w1261, y=w1258) -> (x+y=w1257:i32)
                  n456 = call "Write panel message (SubVI).vi"("Stop BurnIn"=w1247, 4:"rpm"=w1250, 5:"rpm"=TRUE ("rpm"), "PrintTime"=TRUE, "Stop"=w1249, "error in (no error)"=w1246, "Time to wait"=w1256, "Strin"=w1238, "String in"=w1248) -> ("error out"=w1253:errorcluster)  [unwired: 2 in]
                  n457 = control-ref of="Power transistor Heat sink Temp."() -> (w1262:refnum<vi>)
                  n458 = property on="MaxBurnInTempVal" class="DigNum (strict)"() -> ("Value"=w1260:dbl)  [unwired: 2 in, 2 out]
                  n459 = property class="DigNum (strict)"(reference=w1262, error in=w1253) -> (error out=w1241:errorcluster, "Value"=w1259:dbl)  [unwired: 1 out]
                  n460 = Less Or Equal?(x=w1259, y=w1260) -> (x <= y?=w1236:bool)
                  n461 = call "PassOrFail (SubVI).vi"("index (row)"=w1257, "error in (no error)"=w1241, "Data in"=w1259, "Pass?Fail"=w1236, "Table in"=w1251) -> ("error out"=w1240:errorcluster)  [unwired: 6 in]
                }
                n462 = And Array Elements(Boolean array=w1208) -> (logical AND=→"BurnResult":bool)
                n463 = property on="Stop Burn-in" class="Bool (strict)"(error in=w1218, "Value"=w1217, "Visible"=w1217) -> ()  [unwired: 1 in, 2 out]
              }
              frame "Ambient Temp" {
                w1278 = 2 ("disabled index (col)")
                n464 = control-ref of="Power transistor Heat sink Temp."() -> (w1288:refnum<vi>)
                n465 = Equal?(x=w1264, y=u8 95) -> (x = y?=w1267:bool)
                n466 = Select(t="8.3" ("Test Paragraph"), s=w1267, f="7.3" ("Test Paragraph")) -> (s? t:f=w1265:string)
                n467 = call "Find_Number_LineMARVIN from number.vi"("Test Paragraph"=w1265, "TableIn"=w1273) -> ("error out"=w1299:errorcluster, "Line number"=w1279:i32)  [unwired: 3 in, 2 out]
                n468 = property class="DigNum (strict)"(reference=w1288, error in=w1299) -> (error out=w1290:errorcluster, "Value"=w1280:dbl)  [unwired: 1 out]
                n469 = Select(t=25.0 ("y"), s=w1267, f=25.0 ("y")) -> (s? t:f=w1289:dbl)
                n470 = Select(t=13.0 ("y"), s=w1267, f=13.0) -> (s? t:f=w1291:dbl)
                n471 = Add(x=w1289, y=w1291) -> (x+y=w1298:dbl)
                n472 = Subtract(x=w1289, y=w1291) -> (x-y=w1297:dbl)
                n473 = In Range and Coerce(upper limit=w1298, x=w1280, lower limit=w1297) -> (In Range?=w1263:bool)  [unwired: 1 out]
                "BurnTemp" <- w1263
                n474 = call "PassOrFail (SubVI).vi"("index (row)"=w1279, "error in (no error)"=w1290, "Data in"=w1280, "Pass?Fail"=w1263, "Table in"=w1273) -> ("error out"=w1270:errorcluster)  [unwired: 6 in]
                n475 = property class="Tbl (strict)"(reference=w1273, error in=w1270) -> (reference out=w1272:refnum<vi>, error out=w1287:errorcluster, "Value"=w1286:string[][])
                n476 = Add(x=w1280, y=25.0) -> (x+y=w1271:dbl)
                "MaxBurnInTempVal" <- w1271
                n477 = Number To Fractional String(number=w1271, precision (6)=i16 0) -> (F-format string=w1285:string)  [unwired: 2 in]
                n478 = Concatenate Strings("< " ("string"), w1285) -> (w1274:string)
                n479 = Increment(x=w1279) -> (x+1=w1277:i32)
                n480 = Increment(x=w1277) -> (x+1=w1276:i32)
                n481 = Increment(x=w1276) -> (x+1=w1275:i32)
                n482 = Replace Array Subset(array=w1286, new element #1=w1274, index (row) #1=w1277, index (col) #1=w1278, new element #2=w1274, index (row) #2=w1276, index (col) #2=w1278, new element #3=w1274, index (row) #3=w1275, index (col) #3=w1278) -> (w1284:string[][])
                n483 = property class="Tbl (strict)"(reference=w1272, error in=w1287, "Value"=w1284) -> (error out=w1269:errorcluster)  [unwired: 1 out]
                n484 = property class="Bool (strict)"(reference=w1302, error in=w1269) -> ("Value"=w1306:bool)  [unwired: 2 out]
                n485 = Select(t=T16."Stop", s=w1306, f=T16."BurnIn") -> (s? t:f=w1303:T16)
              }
              frame "MotorSpeed" {
                n486 = control-ref of="Motor Speed RPM"() -> (w1314:refnum<vi>)
                n487 = Equal?(x=w1308, y=u8 95) -> (x = y?=w1311:bool)
                n488 = Select(t="8.2" ("Test Paragraph"), s=w1311, f="7.2" ("Test Paragraph")) -> (s? t:f=w1309:string)
                n489 = call "Find_Number_LineMARVIN from number.vi"("Test Paragraph"=w1309, "TableIn"=w1316) -> ("error out"=w1328:errorcluster, "Line number"=w1319:i32)  [unwired: 3 in, 2 out]
                n490 = property class="DigNum (strict)"(reference=w1314, error in=w1328) -> (error out=w1317:errorcluster, "Value"=w1318:dbl)  [unwired: 1 out]
                n491 = Select(t=15100.0 ("y"), s=w1311, f=12100.0 ("y")) -> (s? t:f=w1315:dbl)
                n492 = Select(t=200.0 ("y"), s=w1311, f=200.0) -> (s? t:f=w1320:dbl)
                n493 = Add(x=w1315, y=w1320) -> (x+y=w1327:dbl)
                n494 = Subtract(x=w1315, y=w1320) -> (x-y=w1326:dbl)
                n495 = In Range and Coerce(upper limit=w1327, x=w1318, lower limit=w1326) -> (In Range?=w1307:bool)  [unwired: 1 out]
                "BurnSpeed" <- w1307
                n496 = call "PassOrFail (SubVI).vi"("index (row)"=w1319, "error in (no error)"=w1317, "Data in"=w1318, "Pass?Fail"=w1307, "Table in"=w1316) -> ("error out"=w1313:errorcluster)  [unwired: 6 in]
                n497 = property class="Bool (strict)"(reference=w1331, error in=w1313) -> ("Value"=w1335:bool)  [unwired: 2 out]
                n498 = Select(t=T16."Stop", s=w1335, f=T16."Ambient Temp") -> (s? t:f=w1332:T16)
              }
              frame "DC Current Measure" {
                n499 = property on="VISA Tester" class="VISAName"() -> (error out=w1360:errorcluster, "Value"=w1364:refnum<visa-resource-name>)  [unwired: 2 in, 1 out]
                n500 = call "GetADCTester (SubVI).vi"("error in (no error)"=w1360, "GetADCTester"=T14."Current", "TimeToGet"=10, "VISA Refnum in"=w1364) -> ("error out"=w1361:errorcluster, "ADCValOutput Single"=w1347:dbl)  [unwired: 5 in, 1 out]
                n501 = Equal?(x=w1340, y=u8 95) -> (x = y?=w1344:bool)
                n502 = Select(t="8.1" ("Test Paragraph"), s=w1344, f="7.1" ("Test Paragraph")) -> (s? t:f=w1342:string)
                n503 = call "Find_Number_LineMARVIN from number.vi"("Test Paragraph"=w1342, "error in"=w1361, "TableIn"=w1348) -> ("error out"=w1359:errorcluster, "Line number"=w1349:i32)  [unwired: 2 in, 2 out]
                n504 = Select(t=50.0 ("y"), s=w1344, f=28.0 ("y")) -> (s? t:f=w1351:dbl)
                n505 = Select(t=5.0 ("y"), s=w1344, f=3.0) -> (s? t:f=w1350:dbl)
                n506 = Add(x=w1351, y=w1350) -> (x+y=w1358:dbl)
                n507 = Subtract(x=w1351, y=w1350) -> (x-y=w1357:dbl)
                n508 = In Range and Coerce(upper limit=w1358, x=w1347, lower limit=w1357) -> (In Range?=w1338:bool)  [unwired: 1 out]
                "BurnDC" <- w1338
                n509 = call "PassOrFail (SubVI).vi"("index (row)"=w1349, "error in (no error)"=w1359, "Data in"=w1347, "Pass?Fail"=w1338, "Table in"=w1348) -> ("error out"=w1346:errorcluster)  [unwired: 6 in]
                n510 = property class="Bool (strict)"(reference=w1366, error in=w1346) -> ("Value"=w1337:bool)  [unwired: 2 out]
                n511 = Not(x=w1338) -> (.not. x?=w1336:bool)
                n512 = Or(x=w1336, y=w1337) -> (x .or. y?=w1339:bool)
                n513 = Select(t=T16."Stop", s=w1339, f=T16."MotorSpeed") -> (s? t:f=w1367:T16)
              }
              frame "Start" {
                n514 = Equal?(x=w1375, y=u8 95) -> (x = y?=w1377:bool)
                n515 = Select(t="8" ("Test Paragraph"), s=w1377, f="7" ("Test Paragraph")) -> (s? t:f=w1372:string)
                n516 = Concatenate Strings(w1372, ". Burn-in test in process...\nFull Speed Operation" ("Value")) -> (w1371:string)
                n517 = property class="Str"(reference=w1397, "Value"=w1371) -> (reference out=w1394:refnum<vi>, error out=w1380:errorcluster)  [unwired: 1 in]
                n518 = call "Find_Number_LineMARVIN from number.vi"("Test Paragraph"=w1372, "error in"=w1380, "TableIn"=w1370) -> ("error out"=w1404:errorcluster, "Line number"=w1405:i32)  [unwired: 2 in, 2 out]
                n519 = Select(t=u16 15100 ("y"), s=w1377, f=u16 12100 ("y")) -> (s? t:f=w1411:u16)
                n520 = call "Table_ScrollaBarMarvin.vi"("error in"=w1404, "Line to focus"=w1372, "TableIn"=w1370) -> ("error out"=w1406:errorcluster)  [unwired: 1 in, 2 out]
                n521 = call "Reset old test Values (SubVI) from number.vi"("error in"=w1406, "Atr in"=w1370, "Test Paragraph"=w1372) -> ("error out"=w1407:errorcluster)  [unwired: 8 in]
                n522 = Increment(x=w1405) -> (x+1=w1398:i32)
                n523 = property on="VISA Tester" class="VISAName"(error in=w1407) -> (error out=w1408:errorcluster, "Value"=w1409:refnum<visa-resource-name>)  [unwired: 1 in, 1 out]
                n524 = call "TesterOption (SubVI).vi"("2 Options"=FALSE, "error in (no error)"=w1408, "On/Off"=TRUE, "Tester Option"=T12."Venable", "VISA Refnum in"=w1409) -> ("error out"=w1410:errorcluster)  [unwired: 5 in, 1 out]
                n525 = call "CANSendMotorSpeed.vi"("Remote"=TRUE, "error in (no error)"=w1410, "Motor Speed RPM"=w1411, "UUT"=w1376, "CAN Cluster in"=w1396) -> ("error out"=w1395:errorcluster)  [unwired: 6 in]
                n526 = control-ref of="Motor Speed RPM"() -> (w1384:refnum<vi>)
                n527 = call "Write panel message (SubVI).vi"("Stop BurnIn"=w1381, 4:"rpm"=w1384, 5:"rpm"=TRUE ("rpm"), "PrintTime"=TRUE, "Stop"=w1390, "error in (no error)"=w1395, "Time to wait"=50.0, "Strin"=w1371, "String in"=w1394) -> ("error out"=w1383:errorcluster)  [unwired: 2 in]
                n528 = property class="Bool (strict)"(reference=w1390, error in=w1383) -> ("Value"=w1389:bool)  [unwired: 2 out]
                n529 = Select(t=T16."Stop", s=w1389, f=T16."DC Current Measure") -> (s? t:f=w1386:T16)
              }
            }
          }
        }
        frame "Visual Inspec" {
          n530 = property on="VISA Tester" class="VISAName"() -> ("Value"=w1423:refnum<visa-resource-name>)  [unwired: 2 in, 2 out]
          n531 = call "TesterOption (SubVI).vi"("2 Options"=FALSE, "error in (no error)"=w1412, "On/Off"=FALSE, "Tester Option"=T12."Venable", "VISA Refnum in"=w1423) -> ("error out"=w1419:errorcluster)  [unwired: 5 in, 1 out]
          n532 = local read "UUT"() -> (w1415:u8)
          n533 = Equal?(x=w1415, y=u8 95) -> (x = y?=w1416:bool)
          n534 = case shown="False" w1416 {
            tunnel: w1424 -> [w1428 w1437]
            tunnel: w1419 -> [w1427 w1436]
            tunnel: [w1429 w1440] -> w1418
            tunnel: [w1430 w1439] -> w1414
            frame False {
              # "AHU"
              n535 = for {
                tunnel: string[] ["8.1", "8.2", "9.1", "10.1", "10.2", "10.3", "10.4", "11", "12.1", "13.1", "13.2", "14.1", "14.2", "14.3", "15.1", "16", "17"] ("Array 3") -> [w1434] mode=indexing
                tunnel: w1428 -> [w1433]
                tunnel: w1427 -> [w1432]
                tunnel: [w1431] -> w1426
                n536 = call "Reset old test Values (SubVI) from number.vi"("error in"=w1432, "Atr in"=w1433, "Test Paragraph"=w1434) -> ("error out"=w1431:errorcluster)  [unwired: 8 in]
              }
              n537 = call "VisualInspectionAHUold.vi"("error in (no error)"=w1426, "TableRef"=w1428) -> ("error out"=w1430:errorcluster, "VisualInspectionResult"=w1429:bool)  [unwired: 8 in]
            }
            frame True {
              # "EBAY"
              n538 = for {
                tunnel: string[] ["10.1", "10.2", "11.1", "12.1", "12.2", "12.3", "12.4", "13", "14.1", "15.1", "15.2", "16.1", "16.2", "16.3", "17.1", "18", "19"] ("Array 4") -> [w1444] mode=indexing
                tunnel: w1437 -> [w1443]
                tunnel: w1436 -> [w1442]
                tunnel: [w1441] -> w1435
                n539 = call "Reset old test Values (SubVI) from number.vi"("error in"=w1442, "Atr in"=w1443, "Test Paragraph"=w1444) -> ("error out"=w1441:errorcluster)  [unwired: 8 in]
              }
              n540 = call "VisualInspectionEBAYold.vi"("error in (no error)"=w1435, "TableRef"=w1437) -> ("error out"=w1439:errorcluster, "VisualInspectionResult"=w1440:bool)  [unwired: 8 in]
            }
          }
          "VisualInspectionResult" <- w1418
          n541 = property on="Automation" class="Bool (strict)"(error in=w1414) -> ("Value"=w1413:bool)  [unwired: 1 in, 2 out]
          n542 = case shown="True" w1413 {
            frame False {
            }
            frame True {
              w1445 = TRUE ("Value (Signaling)")
              n543 = property on="SetSN" class="Bool (strict)"("Val(Sgnl)"=w1445, "Value"=w1445) -> ()  [unwired: 2 in, 2 out]
            }
          }
        }
        frame "Temp Sens Cal" {
          w1450 = "2. Temperature sensor calibration test in process..." ("Value")
          w1448 = "2" ("Test Paragraph")
          n544 = control-ref of="Pannel User Message"() -> (w1457:refnum<vi>)
          n545 = property class="Str"(reference=w1457, error in=w1456, "Value"=w1450) -> (error out=w1455:errorcluster)  [unwired: 1 out]
          n546 = call "Table_ScrollaBarMarvin.vi"("error in"=w1455, "Line to focus"=w1448, "TableIn"=w1446) -> ("error out"=w1459:errorcluster)  [unwired: 1 in, 2 out]
          n547 = property class="Tbl (strict)"(reference=w1446, error in=w1459) -> (reference out=w1447:refnum<vi>, error out=w1461:errorcluster, "Value"=w1462:string[][])
          n548 = Index Array(array=w1462, index (col)=0 ("disabled index (col)")) -> (element=w1463:string[])  [unwired: 1 in]
          n549 = call "Find_Number_LineMARVIN from number.vi"("Test Paragraph"=w1448, "error in"=w1461, "TableIn"=w1446, "Row Headers[]"=w1463) -> ("error out"=w1458:errorcluster, "Line number"=w1452:i32)  [unwired: 1 in, 2 out]
          n550 = property on="Status" class="Bool (strict)"(error in=w1458) -> (error out=w1453:errorcluster, "Value"=w1454:bool)  [unwired: 1 in, 1 out]
          n551 = call "Reset old test Values (SubVI) from number.vi"("error in"=w1453, "Atr in"=w1447, "Test Paragraph"=w1448) -> ("error out"=w1449:errorcluster)  [unwired: 8 in]
          n552 = case shown="True" w1454 {
            selector: w1454 -> [w1467 _]
            tunnel: w1449 -> [w1469 _]
            tunnel: w1447 -> [w1466 _]
            tunnel: w1452 -> [w1465 _]
            tunnel: w1451 -> [_ w1476]
            tunnel: w1450 -> [_ w1472]
            frame False {
              n553 = flat-sequence {
                tunnel: w1469 -> [w1470]
                tunnel: [w1470] -> w1468
                frame #0 {
                  n554 = One Button Dialog(message="Please establish RS connection.") -> ()  [unwired: 1 in, 1 out]
                }
              }
              n555 = Increment(x=w1465) -> (x+1=w1464:i32)
              n556 = call "PassOrFail (SubVI).vi"("index (row)"=w1464, "error in (no error)"=w1468, "Pass?Fail"=w1467, "Table in"=w1466) -> ()  [unwired: 7 in, 1 out]
            }
            frame True {
              n557 = control-ref of="Stop Burn-in"() -> (w1478:refnum<vi>)
              n558 = control-ref of="Pannel User Message"() -> (w1480:refnum<vi>)
              n559 = control-ref of="Config_CANAT"() -> (w1474:refnum<vi>)
              n560 = control-ref of="ATR"() -> (w1481:refnum<vi>)
              n561 = control-ref of="Motor Speed RPM"() -> (w1482:refnum<vi>)
              n562 = control-ref of="UUT"() -> (w1473:refnum<vi>)
              n563 = control-ref of="Stop Button"() -> (w1479:refnum<vi>)
              n564 = property on="VISA Tester" class="VISAName"() -> ("Value"=w1475:refnum<visa-resource-name>)  [unwired: 2 in, 2 out]
              n565 = while {
                shift-right: [w1485] -> _
                shift-left: T15."Start" -> [w1495]
                tunnel: w1478 -> [w1494]
                tunnel: w1479 -> [w1493]
                tunnel: w1480 -> [w1492]
                tunnel: w1481 -> [w1491]
                tunnel: w1482 -> [w1490]
                tunnel: w1476 -> [w1489]
                tunnel: w1475 -> [w1488]
                tunnel: w1474 -> [w1487]
                tunnel: w1473 -> [w1486]
                tunnel: w1472 -> [w1483]
                stop <- w1484 stop-if-true
                n566 = case shown="\"AO[1]=Meas.\"" w1495 {
                  tunnel: w1494 -> [_ w1530 w1557 w1612 w1642]
                  tunnel: w1493 -> [_ w1531 w1549 w1598 w1644]
                  tunnel: w1492 -> [_ w1528 w1558 w1610 w1646]
                  tunnel: w1491 -> [_ w1508 _ _ _]
                  tunnel: w1490 -> [_ w1532 w1556 w1613 w1641]
                  tunnel: w1489 -> [_ w1541 w1561 w1622 w1638]
                  tunnel: w1488 -> [w1498 w1537 w1560 w1618 w1626]
                  tunnel: w1487 -> [_ _ _ _ w1652]
                  tunnel: w1486 -> [_ _ _ _ w1651]
                  tunnel: [w1496 w1517 w1550 w1601 w1629] -> w1485
                  tunnel: [w1497 FALSE FALSE FALSE FALSE] -> w1484
                  tunnel: w1483 -> [_ _ w1559 _ _]
                  frame "Stop", Default {
                    n567 = flat-sequence {
                      tunnel: w1498 -> [w1499]
                      tunnel: [TRUE] -> w1497
                      tunnel: [T15."Stop"] -> w1496
                      frame #0 {
                        n568 = call "TesterOption (SubVI).vi"("2 Options"=FALSE, "On/Off"=FALSE, "Tester Option"=T12."Venable", "VISA Refnum in"=w1499) -> ()  [unwired: 6 in, 2 out]
                      }
                      frame #1 {
                      }
                    }
                  }
                  frame "AO[1]=Meas." {
                    n569 = property on="AO[1]Meas" class="DigNum (strict)"() -> ("Value"=w1511:dbl)  [unwired: 2 in, 2 out]
                    n570 = Number To Fractional String(number=w1511) -> (F-format string=w1519:string)  [unwired: 3 in]
                    n571 = Search and Replace String(input string="EP=1\r\nAO[1]=0\r\n" ("write buffer"), search string="0", replace string=w1519) -> (result string=w1518:string)  [unwired: 5 in, 3 out]
                    n572 = call "SerialMarvinSendGet.vi"("Clear Log"=FALSE, "write buffer"=w1518, "VISA resource name"=w1541) -> ("error out"=w1536:errorcluster)  [unwired: 7 in, 1 out]
                    n573 = call "TesterOption (SubVI).vi"("2 Options"=FALSE, "error in (no error)"=w1536, "On/Off"=FALSE, "Tester Option"=T12."Power", "VISA Refnum in"=w1537) -> ("error out"=w1535:errorcluster, "VISA Refnum out"=w1522:refnum<visa-resource-name>)  [unwired: 5 in]
                    n574 = call "Write panel message (SubVI).vi"("Stop BurnIn"=w1530, 4:"rpm"=w1532, 5:"rpm"=FALSE ("rpm"), "PrintTime"=TRUE, "Stop"=w1531, "error in (no error)"=w1535, "Time to wait"=20.0, "Strin"="2. Temperature sensor calibration test in process...\nSet Parameters...", "String in"=w1528) -> ("error out"=w1523:errorcluster)  [unwired: 2 in]
                    n575 = call "TesterOption (SubVI).vi"("2 Options"=FALSE, "error in (no error)"=w1523, "On/Off"=FALSE, "Tester Option"=T12."Venable", "VISA Refnum in"=w1522) -> ("error out"=w1516:errorcluster)  [unwired: 5 in, 1 out]
                    n576 = flat-sequence {
                      tunnel: [T15."Stop"] -> w1517
                      tunnel: w1509 -> [_]
                      frame #0 {
                      }
                    }
                    n577 = In Range and Coerce(upper limit=0.1, x=w1511, lower limit=-0.1) -> (In Range?=w1506:bool)  [unwired: 1 out]
                    "SensCalResult" <- w1506
                    n578 = call "Find_Number_LineMARVIN from number.vi"("Test Paragraph"="2.1", "error in"=w1516, "TableIn"=w1508) -> ("error out"=w1510:errorcluster, "Line number"=w1514:i32)  [unwired: 2 in, 2 out]
                    n579 = call "PassOrFail (SubVI).vi"("Test#"="2", "index (row)"=w1514, "error in (no error)"=w1510, "Data in"=w1511, "Pass?Fail"=w1506, "Table in"=w1508) -> ("error out"=w1509:errorcluster)  [unwired: 5 in]
                  }
                  frame "TA[5]" {
                    w1562 = T18 [enum."50C", enum."80C", enum."100C", enum."120C"] items=["K15", "K16", "K17", "Venable", "Firmeware", "Fan", "Power", "120C", "110C", "100C", "90C", "80C", "70C", "60C", "50C", "40C", "30C", "25C", "20C", "10C", "0C"]
                    n580 = for {
                      tunnel: w1562 -> [w1577] mode=indexing
                      tunnel: w1561 -> [w1576]
                      tunnel: w1560 -> [w1575]
                      tunnel: w1559 -> [w1574]
                      tunnel: w1558 -> [w1573]
                      tunnel: w1549 -> [w1572]
                      tunnel: w1557 -> [w1571]
                      tunnel: w1556 -> [w1570]
                      tunnel: dbl[] [0.59774, 0.65238, 0.68545, 0.71584] -> [w1565] mode=indexing
                      tunnel: [w1564] -> w1545 mode=indexing
                      tunnel: [w1563] -> w1548
                      n581 = for {
                        N: 5 -> [_]
                        tunnel: w1577 -> [w1595]
                        tunnel: w1576 -> [w1594]
                        tunnel: w1575 -> [w1590]
                        tunnel: w1574 -> [w1588]
                        tunnel: w1573 -> [w1587]
                        tunnel: w1572 -> [w1586]
                        tunnel: w1571 -> [w1584]
                        tunnel: w1570 -> [w1581]
                        tunnel: [w1580] -> w1569 mode=indexing
                        tunnel: [w1579] -> w1563
                        n582 = call "TesterOption (SubVI).vi"("2 Options"=FALSE, "On/Off"=TRUE, "Tester Option"=w1595, "VISA Refnum in"=w1590) -> ("error out"=w1591:errorcluster)  [unwired: 6 in, 1 out]
                        n583 = call "Write panel message (SubVI).vi"("Stop BurnIn"=w1584, 4:"rpm"=w1581, 5:"rpm"=FALSE ("rpm"), "PrintTime"=FALSE, "Stop"=w1586, "error in (no error)"=w1591, "Time to wait"=1.0, "Strin"=w1588, "String in"=w1587) -> ("error out"=w1589:errorcluster)  [unwired: 2 in]
                        n584 = call "SerialMarvinSendGet.vi"("error in (no error)"=w1589, "write buffer"="TA[5]\r\n", "VISA resource name"=w1594) -> ("error out"=w1579:errorcluster, "read buffer"=w1592:string)  [unwired: 7 in]
                        n585 = Fract/Exp String To Number(string=w1592) -> (number=w1580:dbl)  [unwired: 3 in, 1 out]
                      }
                      n586 = Add Array Elements(numeric array=w1569) -> (sum=w1568:dbl)
                      n587 = Divide(x=w1568, y=5.0) -> (x/y=w1566:dbl)
                      n588 = Subtract(x=w1566, y=w1565) -> (x-y=w1564:dbl)
                    }
                    n589 = property class="Bool (strict)"(reference=w1549, error in=w1548) -> ("Value"=w1554:bool)  [unwired: 2 out]
                    n590 = Select(t=T15."Stop", s=w1554, f=T15."AO[1]=Meas.") -> (s? t:f=w1550:T15)
                    n591 = Array Size(array=w1545) -> (size(s)=w1544:i32)
                    n592 = Add Array Elements(numeric array=w1545) -> (sum=w1547:dbl)
                    n593 = Divide(x=w1547, y=w1544) -> (x/y=→"AO[1]Meas":dbl)
                  }
                  frame "AO[1]=0" {
                    n594 = call "SerialMarvinSendGet.vi"("write buffer"="EP=1\r\nAO[1]=0\r\n", "VISA resource name"=w1622) -> ("error out"=w1617:errorcluster)  [unwired: 8 in, 1 out]
                    n595 = call "TesterOption (SubVI).vi"("2 Options"=FALSE, "error in (no error)"=w1617, "On/Off"=FALSE, "Tester Option"=T12."Power", "VISA Refnum in"=w1618) -> ("error out"=w1616:errorcluster, "VISA Refnum out"=w1604:refnum<visa-resource-name>)  [unwired: 5 in]
                    n596 = call "Write panel message (SubVI).vi"("Stop BurnIn"=w1612, 4:"rpm"=w1613, 5:"rpm"=FALSE ("rpm"), "PrintTime"=TRUE, "Stop"=w1598, "error in (no error)"=w1616, "Time to wait"=20.0, "Strin"="2. Temperature sensor calibration test in process...\nSet Parameters...", "String in"=w1610) -> ("error out"=w1605:errorcluster)  [unwired: 2 in]
                    n597 = call "TesterOption (SubVI).vi"("2 Options"=FALSE, "error in (no error)"=w1605, "On/Off"=FALSE, "Tester Option"=T12."Venable", "VISA Refnum in"=w1604) -> ("error out"=w1599:errorcluster)  [unwired: 5 in, 1 out]
                    n598 = property class="Bool (strict)"(reference=w1598, error in=w1599) -> ("Value"=w1603:bool)  [unwired: 2 out]
                    n599 = Select(t=T15."Stop", s=w1603, f=T15."TA[5]") -> (s? t:f=w1601:T15)
                  }
                  frame "Start" {
                    n600 = call "Write panel message (SubVI).vi"("Stop BurnIn"=w1642, 4:"rpm"=w1641, 5:"rpm"=FALSE ("rpm"), "PrintTime"=FALSE, "Stop"=w1644, "Time to wait"=0.1, "Strin"="2. Temperature sensor calibration test in process...\nInitialization state...", "String in"=w1646) -> ("error out"=w1647:errorcluster)  [unwired: 3 in]
                    n601 = call "TesterOption (SubVI).vi"("2 Options"=FALSE, "error in (no error)"=w1647, "On/Off"=FALSE, "Tester Option"=T12."Venable", "VISA Refnum in"=w1626) -> ("error out"=w1649:errorcluster)  [unwired: 5 in, 1 out]
                    n602 = call "CANSendMotorSpeed.vi"("Remote"=TRUE, "error in (no error)"=w1649, "Motor Speed RPM"=u16 0, "UUT"=w1651, "CAN Cluster in"=w1652) -> ("error out"=w1636:errorcluster)  [unwired: 6 in]
                    n603 = call "SerialMarvinSendGet.vi"("error in (no error)"=w1636, "write buffer"="AO[1]\r\n", "VISA resource name"=w1638) -> ("error out"=w1625:errorcluster, "read buffer"=w1635:string)  [unwired: 7 in]
                    n604 = Equal?(x=w1635, y="0.0") -> (x = y?=w1627:bool)
                    n605 = property class="Bool (strict)"(reference=w1644, error in=w1625) -> ("Value"=w1656:bool)  [unwired: 2 out]
                    n606 = Select(t=T15."TA[5]", s=w1627, f=T15."AO[1]=0") -> (s? t:f=w1631:T15)
                    n607 = Select(t=T15."Stop", s=w1656, f=w1631) -> (s? t:f=w1629:T15)
                  }
                }
              }
            }
          }
        }
        frame "Auxiliary" {
          w1662 = "9. Auxiliary test in process..." ("Value")
          w1672 = "9" ("Test Paragraph")
          n608 = control-ref of="Pannel User Message"() -> (w1671:refnum<vi>)
          n609 = property class="Str"(reference=w1671, error in=w1669, "Value"=w1662) -> (error out=w1670:errorcluster)  [unwired: 1 out]
          n610 = call "Table_ScrollaBarMarvin.vi"("error in"=w1670, "Line to focus"=w1672, "TableIn"=w1657) -> ("error out"=w1678:errorcluster)  [unwired: 1 in, 2 out]
          n611 = property class="Tbl (strict)"(reference=w1657, error in=w1678) -> (reference out=w1658:refnum<vi>, error out=w1677:errorcluster, "Value"=w1676:string[][])
          n612 = Index Array(array=w1676, index (col)=0 ("disabled index (col)")) -> (element=w1675:string[])  [unwired: 1 in]
          n613 = call "Find_Number_LineMARVIN from number.vi"("Test Paragraph"=w1672, "error in"=w1677, "TableIn"=w1658, "Row Headers[]"=w1675) -> ("error out"=w1673:errorcluster, "Line number"=w1660:i32)  [unwired: 1 in, 2 out]
          n614 = call "Reset old test Values (SubVI) from number.vi"("error in"=w1673, "Atr in"=w1658, "Test Paragraph"=w1672) -> ("error out"=w1667:errorcluster)  [unwired: 8 in]
          n615 = property on="VISA Tester" class="VISAName"() -> ("Value"=w1661:refnum<visa-resource-name>)  [unwired: 2 in, 2 out]
          n616 = control-ref of="Stop Burn-in"() -> (w1664:refnum<vi>)
          n617 = control-ref of="Stop Button"() -> (w1665:refnum<vi>)
          n618 = control-ref of="Pannel User Message"() -> (w1666:refnum<vi>)
          n619 = control-ref of="ATR"() -> (w1659:refnum<vi>)
          n620 = control-ref of="Config_CANAT"() -> ()  [unwired: 1 out]
          n621 = control-ref of="Motor Speed RPM"() -> (w1663:refnum<vi>)
          n622 = while {
            shift-right: [w1683] -> _
            shift-left: enum16{"Stop", "CoolingON", "HotGunON", "Start"}."Start" -> [w1690]
            tunnel: w1667 -> [w1681]
            tunnel: w1666 -> [w1689]
            tunnel: w1665 -> [w1688]
            tunnel: w1664 -> [w1687]
            tunnel: w1663 -> [w1686]
            tunnel: w1662 -> [w1685]
            tunnel: w1661 -> [w1684]
            tunnel: w1660 -> [w1680]
            tunnel: w1659 -> [w1679]
            stop <- w1682 stop-if-true
            n623 = case shown="\"CoolingON\"" w1690 {
              tunnel: w1689 -> [_ w1735 w1829 w1889]
              tunnel: w1688 -> [_ w1730 w1824 w1875]
              tunnel: w1687 -> [_ w1734 w1828 w1888]
              tunnel: w1686 -> [_ w1733 w1827 w1884]
              tunnel: w1685 -> [_ w1724 w1818 w1883]
              tunnel: w1684 -> [_ w1725 w1819 w1876]
              tunnel: [w1692 w1727 w1821 w1871] -> w1683
              tunnel: [w1691 FALSE FALSE FALSE] -> w1682
              tunnel: w1681 -> [_ w1723 w1817 _]
              tunnel: w1680 -> [_ w1718 w1812 _]
              tunnel: w1679 -> [_ w1714 w1809 _]
              frame "Stop", Default {
                n624 = flat-sequence {
                  tunnel: [enum16{"Stop", "CoolingON", "HotGunON", "Start"}."Stop"] -> w1692
                  tunnel: [TRUE] -> w1691
                  frame #0 {
                    n625 = property on="VISA Tester" class="VISAName"() -> ("Value"=w1696:refnum<visa-resource-name>)  [unwired: 2 in, 2 out]
                    n626 = call "TesterOption (SubVI).vi"("2 Options"=FALSE, "On/Off"=FALSE, "Tester Option"=T12."Venable", "VISA Refnum in"=w1696) -> ()  [unwired: 6 in, 2 out]
                  }
                  frame #1 {
                  }
                }
              }
              frame "CoolingON" {
                n627 = while {
                  tunnel: w1735 -> [w1769]
                  tunnel: w1734 -> [w1768]
                  tunnel: w1733 -> [w1764]
                  tunnel: [w1761] -> w1703
                  tunnel: w1730 -> [w1752]
                  tunnel: w1725 -> [w1739]
                  tunnel: w1724 -> [w1756]
                  tunnel: w1723 -> [w1753]
                  shift-right: [w1745] -> _
                  shift-left: 0.0 -> [w1746]
                  shift-right: [w1742] -> w1702
                  shift-left: 0.0 ("Value") -> [w1744]
                  tunnel: [w1737] -> w1706
                  stop <- w1750 stop-if-true
                  n628 = control-ref of="Power transistor Heat sink Temp."() -> (w1762:refnum<vi>)
                  n629 = property class="DigNum (strict)"(reference=w1762, error in=w1753) -> (error out=w1759:errorcluster, "Value"=w1742:dbl)  [unwired: 1 out]
                  n630 = Equal?(x=w1742, y=w1744) -> (x = y?=w1743:bool)
                  n631 = Number To Fractional String(number=w1742, precision (6)=i16 2) -> (F-format string=w1755:string)  [unwired: 2 in]
                  n632 = case shown="True" w1743 {
                    tunnel: w1746 -> [_ w1789]
                    tunnel: [0.0 w1787] -> w1745
                    tunnel: [FALSE w1786] -> _
                    frame False {
                    }
                    frame True {
                      n633 = Increment(x=w1789) -> (x+1=w1787:dbl)
                      n634 = Greater Or Equal?(x=w1787, y=300.0) -> (x >= y?=w1786:bool)
                    }
                  }
                  n635 = Concatenate Strings(w1756, "\nPCB Temperature [C]: " ("string"), w1755) -> (w1754:string)
                  n636 = call "Write panel message (SubVI).vi"("Stop BurnIn"=w1768, 4:"rpm"=w1764, 5:"rpm"=FALSE ("rpm"), "PrintTime"=FALSE, "Stop"=w1752, "error in (no error)"=w1759, "Time to wait"=0.2, "Strin"=w1754, "String in"=w1769) -> ("error out"=w1758:errorcluster)  [unwired: 2 in]
                  n637 = property class="Bool (strict)"(reference=w1752) -> ("Value"=w1751:bool)  [unwired: 1 in, 2 out]
                  n638 = Less Or Equal?(x=w1742, y=52.0) -> (x <= y?=w1741:bool)
                  n639 = call "GetADCTester (SubVI).vi"("error in (no error)"=w1758, "GetADCTester"=T14."Fan", "VISA Refnum in"=w1739) -> ("error out"=w1761:errorcluster, "ADCValOutput Single"=w1748:dbl)  [unwired: 6 in, 1 out]
                  n640 = Greater?(x=w1748, y=u32 2400) -> (0:w1738:bool)
                  n641 = case shown="True" w1741 {
                    tunnel: [w1776 w1783] -> w1740
                    tunnel: w1741 -> [w1776 w1783]
                    tunnel: w1739 -> [w1774 w1781]
                    tunnel: [w1770 w1777] -> w1737
                    frame False {
                      n642 = call "Time Delay11"() -> ("error out"=w1773:errorcluster)  [unwired: 11 in]
                      n643 = call "GetADCTester (SubVI).vi"("error in (no error)"=w1773, "GetADCTester"=T14."Fan", "VISA Refnum in"=w1774) -> ("ADCValOutput Single"=w1772:dbl)  [unwired: 6 in, 2 out]
                      n644 = Greater?(x=w1772, y=2400.0) -> (0:w1770:bool)
                    }
                    frame True {
                      n645 = call "Time Delay10"() -> ("error out"=w1780:errorcluster)  [unwired: 11 in]
                      n646 = call "GetADCTester (SubVI).vi"("error in (no error)"=w1780, "GetADCTester"=T14."Fan", "VISA Refnum in"=w1781) -> ("ADCValOutput Single"=w1779:dbl)  [unwired: 6 in, 2 out]
                      n647 = Greater?(x=w1779, y=2400.0) -> (0:w1777:bool)
                    }
                  }
                  n648 = Compound Arithmetic op=OR(w1738, w1751, w1740) -> (w1750:bool)
                }
                n649 = In Range and Coerce(upper limit=58.0, x=w1702, lower limit=52.0) -> (In Range?=w1705:bool)  [unwired: 1 out]
                n650 = Build Array(w1706, w1705) -> (w1707:bool[])
                n651 = And Array Elements(Boolean array=w1707) -> (logical AND=→"AuxiOFFResult":bool)
                n652 = Add(x=w1718, y=3) -> (x+y=w1716:i32)
                n653 = call "PassOrFail (SubVI).vi"("index (row)"=w1716, "error in (no error)"=w1703, "Data in"=w1702, "Pass?Fail"=w1705, "Table in"=w1714) -> ("error out"=w1720:errorcluster)  [unwired: 6 in]
                n654 = Select(t="OFF", s=w1706, f="ON") -> (s? t:f=w1710:string)
                n655 = Increment(x=w1716) -> (x+1=w1715:i32)
                n656 = call "PassOrFail (SubVI).vi"("String Res"=w1710, "index (row)"=w1715, "error in (no error)"=w1720, "Data in"=-3.0, "Pass?Fail"=w1706, "Table in"=w1714) -> ("error out"=w1719:errorcluster)  [unwired: 5 in]
                n657 = call "TesterOption (SubVI).vi"("2 Options"=FALSE, "error in (no error)"=w1719, "On/Off"=FALSE, "Tester Option"=T12."Venable" ("Tester Option 2"), "VISA Refnum in"=w1725) -> ("error out"=w1700:errorcluster)  [unwired: 5 in, 1 out]
                n658 = call "Time Delay14"("error in (no error)"=w1700) -> ("error out"=w1699:errorcluster)  [unwired: 10 in]
                n659 = property class="Bool (strict)"(reference=w1730, error in=w1699) -> ("Value"=w1736:bool)  [unwired: 2 out]
                n660 = Select(t=enum16{"Stop", "CoolingON", "HotGunON", "Start"}."Stop", s=w1736, f=enum16{"Stop", "CoolingON", "HotGunON", "Start"}."Stop") -> (s? t:f=w1727:enum16{"Stop", "CoolingON", "HotGunON", "Start"})
              }
              frame "HotGunON" {
                n661 = while {
                  tunnel: w1829 -> [w1862]
                  tunnel: w1828 -> [w1861]
                  tunnel: w1827 -> [w1857]
                  tunnel: [w1853] -> w1799
                  tunnel: w1824 -> [w1844]
                  tunnel: w1819 -> [w1854]
                  tunnel: w1818 -> [w1848]
                  tunnel: w1817 -> [w1845]
                  shift-right: [w1837] -> _
                  shift-left: 0.0 -> [w1838]
                  shift-right: [w1834] -> _
                  shift-left: 0.0 ("Value") -> [w1835]
                  tunnel: [w1832] -> w1797
                  stop <- w1842 stop-if-true
                  n662 = control-ref of="Power transistor Heat sink Temp."() -> (w1855:refnum<vi>)
                  n663 = property class="DigNum (strict)"(reference=w1855, error in=w1845) -> (error out=w1851:errorcluster, "Value"=w1834:dbl)  [unwired: 1 out]
                  n664 = Equal?(x=w1834, y=w1835) -> (x = y?=w1833:bool)
                  n665 = Number To Fractional String(number=w1834, precision (6)=i16 2) -> (F-format string=w1847:string)  [unwired: 2 in]
                  n666 = case shown="True" w1833 {
                    tunnel: w1838 -> [_ w1868]
                    tunnel: [0.0 w1866] -> w1837
                    tunnel: [FALSE w1865] -> w1836
                    frame False {
                    }
                    frame True {
                      n667 = Increment(x=w1868) -> (x+1=w1866:dbl)
                      n668 = Greater Or Equal?(x=w1866, y=300.0) -> (x >= y?=w1865:bool)
                    }
                  }
                  n669 = Concatenate Strings(w1848, "\nPCB Temperature [C]: " ("string"), w1847) -> (w1846:string)
                  n670 = call "Write panel message (SubVI).vi"("Stop BurnIn"=w1861, 4:"rpm"=w1857, 5:"rpm"=FALSE ("rpm"), "PrintTime"=FALSE, "Stop"=w1844, "error in (no error)"=w1851, "Time to wait"=0.2, "Strin"=w1846, "String in"=w1862) -> ("error out"=w1850:errorcluster)  [unwired: 2 in]
                  n671 = property class="Bool (strict)"(reference=w1844) -> ("Value"=w1843:bool)  [unwired: 1 in, 2 out]
                  n672 = call "GetADCTester (SubVI).vi"("error in (no error)"=w1850, "GetADCTester"=T14."Fan", "VISA Refnum in"=w1854) -> ("error out"=w1853:errorcluster, "ADCValOutput Single"=w1840:dbl)  [unwired: 6 in, 1 out]
                  n673 = Greater Or Equal?(x=w1834, y=61.0) -> (x >= y?=w1831:bool)
                  n674 = Less?(x=w1840, y=u32 100) -> (x < y?=w1832:bool)
                  n675 = Compound Arithmetic op=OR(w1832, w1843, w1831, w1836) -> (w1842:bool)
                }
                n676 = control-ref of="Power transistor Heat sink Temp."() -> (w1802:refnum<vi>)
                n677 = property class="DigNum (strict)"(reference=w1802, error in=w1799) -> (error out=w1801:errorcluster, "Value"=w1800:dbl)  [unwired: 1 out]
                n678 = In Range and Coerce(upper limit=62.0, x=w1800, lower limit=58.0) -> (In Range?=w1796:bool)  [unwired: 1 out]
                n679 = Build Array(w1797, w1796) -> (w1798:bool[])
                n680 = Increment(x=w1812) -> (x+1=w1811:i32)
                n681 = call "PassOrFail (SubVI).vi"("index (row)"=w1811, "error in (no error)"=w1801, "Data in"=w1800, "Pass?Fail"=w1796, "Table in"=w1809) -> ("error out"=w1814:errorcluster)  [unwired: 6 in]
                n682 = And Array Elements(Boolean array=w1798) -> (logical AND=→"AuxiONResult":bool)
                n683 = Increment(x=w1811) -> (x+1=w1810:i32)
                n684 = Select(t="ON", s=w1797, f="OFF") -> (s? t:f=w1807:string)
                n685 = call "PassOrFail (SubVI).vi"("String Res"=w1807, "index (row)"=w1810, "error in (no error)"=w1814, "Data in"=-3.0, "Pass?Fail"=w1797, "Table in"=w1809) -> ("error out"=w1813:errorcluster)  [unwired: 5 in]
                n686 = call "TesterOption (SubVI).vi"("On/Off 2"=FALSE, "Tester Option 2"=T12."Venable", "2 Options"=TRUE, "error in (no error)"=w1813, "On/Off"=FALSE, "Tester Option"=T12."Fan", "VISA Refnum in"=w1819) -> ("error out"=w1791:errorcluster)  [unwired: 3 in, 1 out]
                n687 = call "Time Delay13"("error in (no error)"=w1791) -> ("error out"=w1790:errorcluster)  [unwired: 10 in]
                n688 = property class="Bool (strict)"(reference=w1824, error in=w1790) -> ("Value"=w1830:bool)  [unwired: 2 out]
                n689 = Select(t=enum16{"Stop", "CoolingON", "HotGunON", "Start"}."Stop", s=w1830, f=enum16{"Stop", "CoolingON", "HotGunON", "Start"}."CoolingON") -> (s? t:f=w1821:enum16{"Stop", "CoolingON", "HotGunON", "Start"})
              }
              frame "Start" {
                n690 = call "Write panel message (SubVI).vi"("Stop BurnIn"=w1888, 4:"rpm"=w1884, 5:"rpm"=FALSE ("rpm"), "PrintTime"=TRUE, "Stop"=w1875, "Time to wait"=3.0, "Strin"=w1883, "String in"=w1889) -> ("error out"=w1882:errorcluster)  [unwired: 3 in]
                n691 = call "TesterOption (SubVI).vi"("On/Off 2"=TRUE, "Tester Option 2"=T12."Fan", "2 Options"=TRUE, "error in (no error)"=w1882, "On/Off"=FALSE, "Tester Option"=T12."Venable", "VISA Refnum in"=w1876) -> ("error out"=w1874:errorcluster)  [unwired: 3 in, 1 out]
                n692 = call "Time Delay"("error in (no error)"=w1874) -> ("error out"=w1869:errorcluster)  [unwired: 10 in]
                n693 = property class="Bool (strict)"(reference=w1875, error in=w1869) -> ("Value"=w1890:bool)  [unwired: 2 out]
                n694 = Select(t=enum16{"Stop", "CoolingON", "HotGunON", "Start"}."Stop", s=w1890, f=enum16{"Stop", "CoolingON", "HotGunON", "Start"}."HotGunON") -> (s? t:f=w1871:enum16{"Stop", "CoolingON", "HotGunON", "Start"})
              }
            }
          }
        }
      }
    }
    n695 = flat-sequence {
      tunnel: w220 -> [_]
      frame #0 {
        w228 = T20."Enabled" ("Disabled")
        w229 = FALSE ("Start")
        n696 = property on="Start" class="Bool (strict)"("Value"=w229, "DisabledEnum"=w228) -> ()  [unwired: 2 in, 2 out]
        n697 = property on="Report" class="Bool (strict)"("Value"=w229, "DisabledEnum"=w228) -> ()  [unwired: 2 in, 2 out]
      }
    }
  }
  n698 = while {
    shift-right: [w1893] -> _
    shift-left: T10."Initialize" -> [w1912]
    shift-right: [w1909] -> _
    shift-left: _ -> [w1908]
    shift-right: [w1907] -> _
    shift-left: w33 -> [w1905]
    shift-right: [w1906] -> _
    shift-left: refnum<vi> refnum ("Config_CANAT") -> [w1904]
    shift-right: [w1902] -> _
    shift-left: w30 -> [w1903]
    tunnel: "ATR" -> [_]
    tunnel: w22 -> [w1901]
    tunnel: w21 -> [w1900]
    shift-right: [w1898] -> _
    shift-left: w1 -> [w1899]
    tunnel: w8 -> [w1897]
    tunnel: w2 -> [w1896]
    tunnel: w19 -> [_]
    tunnel: w31 -> [w1911]
    tunnel: [w1910] -> _
    tunnel: w9 -> [_]
    tunnel: w6 -> [w1894]
    shift-right: [w1891] -> _
    shift-left: w1 -> [w1892]
    stop <- w1895 stop-if-true
    n699 = case shown="\"MainProgram\"" w1912 {
      tunnel: [w1919 w2062 w2135 T10."Erase ATR Table"] -> w1893
      tunnel: [FALSE w2048 FALSE FALSE] -> w1895
      tunnel: [w1915 w2053 w2129 w3029] -> w1910
      tunnel: w1911 -> [_ w2073 w2133 _]
      tunnel: [w1955 refnum<visa-resource-name> refnum ("VISA resource name") w2130 w3033] -> w1909
      tunnel: w1908 -> [w1955 w2081 w2131 _]
      tunnel: [w1946 w2042 w2125 w3027] -> w1907
      tunnel: [w1945 refnum<vi> refnum ("Config_CANAT") w2126 w3030] -> w1906
      tunnel: w1905 -> [w1946 w2083 w2128 w3027]
      tunnel: w1904 -> [w1945 w2065 w2127 _]
      tunnel: w1903 -> [w1944 w2076 w2124 w3026]
      tunnel: [w1944 w2041 w2123 w3026] -> w1902
      tunnel: w1901 -> [_ _ w2122 _]
      tunnel: w1900 -> [_ _ w2121 _]
      tunnel: w1899 -> [w1941 w2067 w2120 w3023]
      tunnel: [w1941 w2067 w2119 w3023] -> w1898
      tunnel: w1897 -> [w1931 _ w2118 _]
      tunnel: w1896 -> [_ _ w2117 _]
      tunnel: w1894 -> [_ _ w2116 _]
      tunnel: w1892 -> [_ _ w2115 _]
      tunnel: [0 0 w2114 0] -> w1891
      frame "Erase ATR Table", Default {
        w1923 = T20."Enabled" ("Disabled")
        w1935 = "Marvin" ("section")
        w1942 = refnum<visa-resource-name> "COM4" ("VISA resource name")
        w1951 = FALSE ("Visible")
        n700 = property on="Serial Com" class="Bool"(error in=errorcluster {"status"=FALSE, "code"=0, "source"=""} ("error out"), "Visible"=TRUE) -> (error out=w1943:errorcluster)  [unwired: 1 in, 1 out]
        n701 = property on="VISA Marvin" class="VISAName"(error in=w1943, "Visible"=w1951, "Value"=w1942) -> (error out=w1953:errorcluster)  [unwired: 1 in, 1 out]
        n702 = property on="VISA Marvin" class="VISAName"(error in=w1943, "Value"=w1942) -> ()  [unwired: 1 in, 2 out]
        n703 = property on="Status" class="Bool (strict)"(error in=w1953, "Value"=w1951) -> (error out=w1926:errorcluster)  [unwired: 1 in, 1 out]
        n704 = call "Select UUT"("error in (no error)"=w1926) -> ("EBAY"=w1924:bool, "error out"=w1925:errorcluster)  [unwired: 17 in]
        n705 = case shown="True" w1924 {
          tunnel: [string[][] [["1", "Communication Test", "", "", "", "", ""], ["1.1", "Serial RS-232", "N/A", "-", "", "", ""], ["1.2", "CAN Bus", "N/A", "-", "", "", ""], ["", "", "", "", "", "", ""], ["2", "Temperature Sensor Calibration", "", "", "", "", ""], ["2.1", "Sensor Reading Analog Offset", "0", "+/-0.100", ".", "", ""], ["", "", "", "", "", "", ""], ["3", "Motor Termistor Input Test", "", "", "", "", ""], ["3.1", "60 Degree", "60", "+/-3.00", "°C", "", ""], ["3.2", "90 Degree", "90", "+/-3.00", "°C", "", ""], ["3.3", "120 Degree", "120", "+/-3.00", "°C", "", ""], ["", "", "", "", "", "", ""], ["4", "Enable Test", "", "", "", "", ""], ["4.1", "Fan Speed at Opened Enable ", "5000", "+/-200.0", "rpm", "", ""], ["4.2", "Fan Speed at Opened Enable ", "0", "+/-200.0", "rpm", "", ""], ["4.3", "Fan Speed at Closed Enable ", "5000", "+/-200.0", "rpm", "", ""], ["4.4", "Motor Rotation Direction", "CCW", "-", "", "", ""], ["", "", "", "", "", "", ""], ["5", "Speed Command Test", "", "", "", "", ""], ["5.1", "Fan Speed", "6000", "+/-200.0", "rpm", "", ""], ["5.2", "Fan Speed", "9000", "+/-200.0", "rpm", "", ""], ["5.3", "Fan Speed", "12100", "+/-200.0", "rpm", "", ""], ["", "", "", "", "", "", ""], ["6", "Motor Stop time", "< 50", "-", "sec", "", ""], ["", "", "", "", "", "", ""], ["7", "Burn-in Test", "", "", "", "", ""], ["7.1", "DC Input Current", "28", "+/-5.000", "A", "", ""], ["7.2", "Fan Speed", "12100", "+/-200.0", "rpm", "", ""], ["7.3", "Ambient Temperature", "25", "+/-13.00", "°C", "", ""], ["7.4", "After 10 min of operation", "", "-", "°C", "", ""], ["7.5", "After 20 min of operation", "", "-", "°C", "", ""], ["7.6", "After 30 min of operation", "", "-", "°C", "", ""], ["", "", "", "", "", "", ""], ["8", "Visual Inspection", "", "", "", "", ""], ["8.1", "Verification of Components Not Installed", "N/A", "-", "", "", ""], ["8.2", "Manufacturing Defects", "N/A", "-", "", "", ""], ["", "", "", "", "", "", ""], ["9", "Power Supply Testing", "", "", "", "", ""], ["9.1", "DC Input Current Drawn", "150", "+/-10.00", "mA", "", ""], ["", "", "", "", "", "", ""], ["10", "Power Supply Voltages", "", "", "", "", ""], ["10.1", "12V", "12.0", "+/-0.500", "V", "", ""], ["10.2", "5V", "5.0", "+/-0.200", "V", "", ""], ["10.3", "3.3V", "3.3", "+/-0.100", "V", "", ""], ["10.4", "1.8V", "1.8", "+/-0.100", "V", "", ""], ["", "", "", "", "", "", ""], ["11", "Reverse Polarity Test - DC Input Current", "< 1", "-", "mA", "", ""], ["", "", "", "", "", "", ""], ["12", "Functional Test Procedure", "", "", "", "", ""], ["12.1", "Weight Check", "3800", "+/-100.0", "gr", "", ""], ["", "", "", "", "", "", ""], ["13", "Insulation Resistance Test", "", "", "", "", ""], ["13.1", "J3.B to Chassis", "> 1M", "-", "ohms", "", ""], ["13.2", "J1.16 to Chassis", "> 100K", "-", "ohms", "", ""], ["", "", "", "", "", "", ""], ["14", "Bonding Resistance", "", "", "", "", ""], ["14.1", "J1 Body to Chassis", "< 2m", "-", "ohms", "", ""], ["14.2", "J2  Body to Chassis", "< 2m", "-", "ohms", "", ""], ["14.3", "J3  Body to Chassis", "< 2m", "-", "ohms", "", ""], ["", "", "", "", "", "", ""], ["15", "CANbus Resistance Test", "", "", "", "", ""], ["15.1", "J1.17 to J1.18", "> 10K", "-", "ohms", "", ""], ["", "", "", "", "", "", ""], ["16", "Sealing Test", "N/A", "-", "", "", ""], ["", "", "", "", "", "", ""], ["17", "Mounting Holes Test - Jig Fit", "214", "-", "mm", "", ""]] ("ArrAHU 2") string[][] [["1", "Communication Test", "", "", "", "", ""], ["1.1", "Serial RS-232", "N/A", "-", "", "", ""], ["1.2", "CAN Bus", "N/A", "-", "", "", ""], ["", "", "", "", "", "", ""], ["2", "Temperature Sensor Calibration", "", "", "", "", ""], ["2.1", "Sensor Reading Analog Offset", "0", "+/-0.100", ".", "", ""], ["", "", "", "", "", "", ""], ["3", "Motor Termistor Input Test", "", "", "", "", ""], ["3.1", "60 Degree", "60", "+/-3.00", "C", "", ""], ["3.2", "90 Degree", "90", "+/-3.00", "C", "", ""], ["3.3", "120 Degree", "120", "+/-3.00", "C", "", ""], ["", "", "", "", "", "", ""], ["4", "Enable Test", "", "", "", "", ""], ["4.1", "Fan Speed at Opened Enable ", "5000", "+/-200.0", "rpm", "", ""], ["4.2", "Fan Speed at Opened Enable ", "0", "+/-200.0", "rpm", "", ""], ["4.3", "Fan Speed at Closed Enable ", "5000", "+/-200.0", "rpm", "", ""], ["4.4", "Motor Rotation Direction", "CCW", "-", "", "", ""], ["", "", "", "", "", "", ""], ["5", "Speed Command Test", "", "", "", "", ""], ["5.1", "Fan Speed", "6000", "+/-200.0", "rpm", "", ""], ["5.2", "Fan Speed", "11500", "+/-200.0", "rpm", "", ""], ["5.3", "Fan Speed", "15100", "+/-200.0", "rpm", "", ""], ["", "", "", "", "", "", ""], ["6", "Motor Stop time", "< 50", "-", "sec", "", ""], ["", "", "", "", "", "", ""], ["7", "Temperature Control Algorithm Test", "", "", "", "", ""], ["7.1", "Tair <   68 ± 2 oC", "6000", "+/-200.0", "rpm", "", ""], ["7.2", "Measured Temp.", "", "", "°C", "", ""], ["7.3", "Tair >= 68 ± 2 oC", "11500", "+/-200.0", "rpm", "", ""], ["7.4", "Transition Temp.", "", "", "°C", "", ""], ["7.5", "Tair >= 88 ± 2 oC", "15100", "+/-400.0", "rpm", "", ""], ["7.6", "Transition Temp.", "", "", "°C", "", ""], ["7.7", "Tair <= 80 ± 2 oC", "11500", "+/-200.0", "rpm", "", ""], ["7.8", "Transition Temp.", "", "", "°C", "", ""], ["7.9", "Tair <= 60 ± 2 oC", "6000", "+/-200.0", "rpm", "", ""], ["7.10", "Transition Temp.", "", "", "°C", "", ""], ["", "", "", "", "", "", ""], ["8", "Burn-in Test", "", "", "", "", ""], ["8.1", "DC Input Current", "50", "+/-5.000", "A", "", ""], ["8.2", "Fan Speed", "15100", "+/-200.0", "rpm", "", ""], ["8.3", "Ambient Temperature", "25", "+/-13.00", "°C", "", ""], ["8.4", "After 10 min of operation", "", "-", "°C", "", ""], ["8.5", "After 20 min of operation", "", "-", "°C", "", ""], ["8.6", "After 30 min of operation", "", "-", "°C", "", ""], ["", "", "", "", "", "", ""], ["9", "Auxiliary Fan Test", "", "", "", "", ""], ["9.1", "Auxiliary Cooling Fan ON", "60", "+/-2.00", "°C", "", ""], ["9.2", "Fan status", "ON", "-", "-", "", ""], ["9.3", "Auxiliary Cooling Fan OFF", "55", "+/-3.00", "°C", "", ""], ["9.4", "Fan status", "OFF", "-", "-", "", ""], ["", "", "", "", "", "", ""], ["10", "Visual Inspection", "", "", "", "", ""], ["10.1", "Verification of Components Not Installed", "N/A", "-", "", "", ""], ["10.2", "Manufacturing Defects", "N/A", "-", "", "", ""], ["", "", "", "", "", "", ""], ["11", "Power Supply Testing", "", "", "", "", ""], ["11.1", "DC Input Current Drawn", "150", "+/-10.00", "mA", "", ""], ["", "", "", "", "", "", ""], ["12", "Power Supply Voltages", "", "", "", "", ""], ["12.1", "12V", "12.0", "+/-0.500", "V", "", ""], ["12.2", "5V", "5.0", "+/-0.200", "V", "", ""], ["12.3", "3.3V", "3.3", "+/-0.100", "V", "", ""], ["12.4", "1.8V", "1.8", "+/-0.100", "V", "", ""], ["", "", "", "", "", "", ""], ["13", "Reverse Polarity Test - DC Input Current", "< 1", "-", "mA", "", ""], ["", "", "", "", "", "", ""], ["14", "Functional Test Procedure", "", "", "", "", ""], ["14.1", "Weight Check", "4180", "+/-100.0", "gr", "", ""], ["", "", "", "", "", "", ""], ["15", "Insulation Resistance Test", "", "", "", "", ""], ["15.1", "J3.B to Chassis", "> 1M", "-", "ohms", "", ""], ["15.2", "J1.16 to Chassis", "> 100K", "-", "ohms", "", ""], ["", "", "", "", "", "", ""], ["16", "Bonding Resistance", "", "", "", "", ""], ["16.1", "J1 Body to Chassis", "< 2m", "-", "ohms", "", ""], ["16.2", "J2  Body to Chassis", "< 2m", "-", "ohms", "", ""], ["16.3", "J3  Body to Chassis", "< 2m", "-", "ohms", "", ""], ["", "", "", "", "", "", ""], ["17", "CANbus Resistance Test", "", "", "", "", ""], ["17.1", "J1.17 to J1.18", "> 10K", "-", "ohms", "", ""], ["", "", "", "", "", "", ""], ["18", "Sealing Test", "N/A", "-", "", "", ""], ["", "", "", "", "", "", ""], ["19", "Mounting Holes Test - Jig Fit", "214", "-", "mm", "", ""]] ("ArrEbay 2")] -> w1949
          tunnel: ["AHU" "EBAY"] -> w1948
          tunnel: [w2012 w2024] -> w1947
          tunnel: w1925 -> [w2013 w2024]
          tunnel: [w2008 u8 95] -> w1920
          frame False {
            (unwired) string[][] [["6.1", "Visual Inspection", "", "", "", "", ""], ["6.1.1", "Verification of Components Not Installed", "N/A", "-", "", "", ""], ["", "", "", "", "", "", ""], ["6.1.2", "Manufacturing Defects", "N/A", "-", "", "", ""], ["", "", "", "", "", "", ""], ["6.2", "Power Supply Testing", "", "", "", "", ""], ["6.2.1", "Input Current Drawn", "", "", "", "", ""], ["6.2.1.1", "DC Input Current", "< 150", "-", "mA", "", ""], ["", "", "", "", "", "", ""], ["6.2.2", "Power Supply Voltages", "", "", "", "", ""], ["6.2.2.1", "12V", "12.0", "+/-0.500", "V", "", ""], ["6.2.2.2", "5V", "5.0", "+/-0.200", "V", "", ""], ["6.2.2.3", "3.3V", "3.3", "+/-0.100", "V", "", ""], ["6.2.2.4", "1.8V", "1.8", "+/-0.100", "V", "", ""], ["", "", "", "", "", "", ""], ["7", "Functional Test Procedure", "", "", "", "", ""], ["7.1", "Weight Check", "3800", "+/-100.0", "gr", "", ""], ["", "", "", "", "", "", ""], ["7.2", "Insulation Resistance Test", "", "", "", "", ""], ["7.2.1", "J3.B to Chassis", "> 1M", "-", "W", "", ""], ["7.2.2", "J1.16 to Chassis", "> 100K", "-", "W", "", ""], ["", "", "", "", "", "", ""], ["7.2", "Bonding Resistance", "", "", "", "", ""], ["7.2.3", "J1 Body to Chassis", "< 2m", "-", "W", "", ""], ["7.2.4", "J2  Body to Chassis", "< 2m", "-", "W", "", ""], ["7.2.5", "J3  Body to Chassis", "< 2m", "-", "W", "", ""], ["", "", "", "", "", "", ""], ["7.2.1", "CANbus Resistance Test", "", "", "", "", ""], ["7.2.1.1", "J1.17 to J1.18", "> 10K", "-", "W", "", ""], ["", "", "", "", "", "", ""], ["7.3", "Sealing Test", "N/A", "-", "", "", ""], ["", "", "", "", "", "", ""], ["7.4", "Communication Test", "", "", "", "", ""], ["7.4.1", "Serial RS-232", "N/A", "-", "", "", ""], ["7.4.2", "CAN Bus", "N/A", "-", "", "", ""], ["", "", "", "", "", "", ""], ["7.5", "Performances Tests", "", "", "", "", ""], ["7.5.1", "Reverse Polarity Test", "", "", "", "", ""], ["7.5.1.1", "DC Input Current", "< 1", "-", "mA", "", ""], ["", "", "", "", "", "", ""], ["7.5.2", "Enable Test", "", "", "", "", ""], ["7.5.2.1", "Fan Speed at Opened Enable ", "5000", "+/-200.0", "rpm", "", ""], ["7.5.2.2", "Fan Speed at Opened Enable ", "0", "+/-200.0", "rpm", "", ""], ["7.5.2.3", "Fan Speed at Closed Enable ", "5000", "+/-200.0", "rpm", "", ""], ["7.5.2.4", "Motor Rotation Direction", "Counter-clockwise (Inlet)", "-", "", "", ""], ["", "", "", "", "", "", ""], ["7.5.3", "Stop Time Test ", "", "", "", "", ""], ["7.5.3.1", "Motor Stop time", "< 50", "-", "sec", "", ""], ["", "", "", "", "", "", ""], ["7.5.4", "Speed Command Test", "", "", "", "", ""], ["7.5.4.1", "Fan Speed", "6000", "+/-200.0", "rpm", "", ""], ["7.5.4.2", "Fan Speed", "9000", "+/-200.0", "rpm", "", ""], ["7.5.4.3", "Fan Speed", "12100", "+/-200.0", "rpm", "", ""], ["", "", "", "", "", "", ""], ["7.5.5", "Temperature Sensor Calibration Test", "", "", "", "", ""], ["7.5.5.1", "Sensor Reading Analog Offset", "0", "+/-0.100", ".", "", ""], ["", "", "", "", "", "", ""], ["7.5.6", "Burn-in Test", "", "", "", "", ""], ["7.5.6.1", "DC Input Current", "28", "+/-3.000", "A", "", ""], ["7.5.6.2", "Fan Speed", "12100", "+/-200.000", "rpm", "", ""], ["7.5.6.3", "Ambient Temperature", "25", "+/-13.00", "C", "", ""], ["7.5.6.4", "After 10 min of operation", "", "", "C", "", ""], ["7.5.6.5", "After 20 min of operation", "", "", "C", "", ""], ["7.5.6.6", "After 30 min of operation", "", "", "C", "", ""], ["", "", "", "", "", "", ""], ["9", "Motor Temp Test", "", "", "", "", ""], ["9.1", "60 C", "60", "+/-3.000", "C", "", ""], ["9.2", "90 C", "90", "+/-3.000", "C", "", ""], ["9.3", "120 C", "120", "+/-3.000", "C", "", ""]] ("data")
            n706 = while {
              shift-right: [w2020] -> w2012
              shift-left: w2013 -> [w2021]
              tunnel: [w2015] -> w2011
              stop <- w2019 stop-if-true
              n707 = call "AHU UUT (subVI).vi"("error in (no error)"=w2021) -> ("AHU 47"=w2016:bool, "AHU 63"=w2015:bool, "OK"=w2018:bool, "error out"=w2020:errorcluster)  [unwired: 15 in]
              n708 = Exclusive Or(1:w2016, 2:w2015) -> (0:w2017:bool)
              n709 = And(x=w2018, y=w2017) -> (x .and. y?=w2019:bool)
            }
            n710 = Select(t=u8 63, s=w2011, f=u8 47) -> (s? t:f=w2008:u8)
          }
          frame True {
            (unwired) string[][] [["6.1", "Visual Inspection", "", "", "", "", ""], ["6.1.1", "Verification of Components Not Installed", "N/A", "-", "", "", ""], ["", "", "", "", "", "", ""], ["6.1.2", "Manufacturing Defects", "N/A", "-", "", "", ""], ["", "", "", "", "", "", ""], ["6.2", "Power Supply Testing", "", "", "", "", ""], ["6.2.1", "Input Current Drawn", "", "", "", "", ""], ["6.2.1.1", "DC Input Current", "< 150", "-", "mA", "", ""], ["", "", "", "", "", "", ""], ["6.2.2", "Power Supply Voltages", "", "", "", "", ""], ["6.2.2.1", "12V", "12.0", "+/-0.500", "V", "", ""], ["6.2.2.2", "5V", "5.0", "+/-0.200", "V", "", ""], ["6.2.2.3", "3.3V", "3.3", "+/-0.100", "V", "", ""], ["6.2.2.4", "1.8V", "1.8", "+/-0.100", "V", "", ""], ["", "", "", "", "", "", ""], ["7", "Functional Test Procedure", "", "", "", "", ""], ["7.1", "Weight Check", "4180", "+/-10.00", "gr", "", ""], ["", "", "", "", "", "", ""], ["7.2", "Insulation Resistance Test", "", "", "", "", ""], ["7.2.1", "J3.B to Chassis", "> 1M", "-", "W", "", ""], ["7.2.2", "J1.16 to Chassis", "> 100K", "-", "W", "", ""], ["", "", "", "", "", "", ""], ["7.2", "Bonding Resistance", "", "", "", "", ""], ["7.2.3", "J1 Body to Chassis", "< 2m", "-", "W", "", ""], ["7.2.4", "J2  Body to Chassis", "< 2m", "-", "W", "", ""], ["7.2.5", "J3  Body to Chassis", "< 2m", "-", "W", "", ""], ["", "", "", "", "", "", ""], ["7.2.1", "CANbus Resistance Test", "", "", "", "", ""], ["7.2.1.1", "J1.17 to J1.18", "> 10K", "-", "W", "", ""], ["", "", "", "", "", "", ""], ["7.3", "Sealing Test", "N/A", "-", "", "", ""], ["", "", "", "", "", "", ""], ["7.4", "Communication Test", "", "", "", "", ""], ["7.4.1", "Serial RS-232", "N/A", "-", "", "", ""], ["7.4.2", "CAN Bus", "N/A", "-", "", "", ""], ["", "", "", "", "", "", ""], ["7.5", "Performances Tests", "", "", "", "", ""], ["7.5.1", "Reverse Polarity Test", "", "", "", "", ""], ["7.5.1.1", "DC Input Current", "< 1", "-", "mA", "", ""], ["", "", "", "", "", "", ""], ["7.5.2", "Enable Test", "", "", "", "", ""], ["7.5.2.1", "Fan Speed at Opened Enable ", "5000", "+/-200.0", "rpm", "", ""], ["7.5.2.2", "Fan Speed at Opened Enable ", "0", "+/-200.0", "rpm", "", ""], ["7.5.2.3", "Fan Speed at Closed Enable ", "5000", "+/-200.0", "rpm", "", ""], ["7.5.2.4", "Motor Rotation Direction", "Counter-clockwise (Inlet)", "-", "", "", ""], ["", "", "", "", "", "", ""], ["7.5.3", "Stop Time Test ", "", "", "", "", ""], ["7.5.3.1", "Motor Stop time", "< 50", "-", "sec", "", ""], ["", "", "", "", "", "", ""], ["7.5.4", "Speed Command Test", "", "", "", "", ""], ["7.5.4.1", "Fan Speed", "6000", "+/-200.0", "rpm", "", ""], ["7.5.4.2", "Fan Speed", "11500", "+/-200.0", "rpm", "", ""], ["7.5.4.3", "Fan Speed", "15100", "+/-200.0", "rpm", "", ""], ["", "", "", "", "", "", ""], ["7.5.5", "Temperature Sensor Calibration Test", "", "", "", "", ""], ["7.5.5.1", "Sensor Reading Analog Offset", "0", "+/-0.100", ".", "", ""], ["", "", "", "", "", "", ""], ["7.5.6", "Temperature Control Algorithm Test", "", "", "", "", ""], ["7.5.6.1", "Tair <   68 ± 2 oC", "6000", "+/-200.0", "rpm", "", ""], ["7.5.6.2", "Measured Temp.", "", "", "C", "", ""], ["7.5.6.3", "Tair >= 68 ± 2 oC", "11500", "+/-200.0", "rpm", "", ""], ["7.5.6.4", "Transition Temp.", "", "", "C", "", ""], ["7.5.6.5", "Tair >= 88 ± 2 oC", "15100", "+/-400.0", "rpm", "", ""], ["7.5.6.6", "Transition Temp.", "", "", "C", "", ""], ["7.5.6.7", "Tair <= 80 ± 2 oC", "11500", "+/-200.0", "rpm", "", ""], ["7.5.6.8", "Transition Temp.", "", "", "C", "", ""], ["7.5.6.9", "Tair <= 60 ± 2 oC", "6000", "+/-200.0", "rpm", "", ""], ["7.5.6.10", "Transition Temp.", "", "", "C", "", ""], ["", "", "", "", "", "", ""], ["7.5.7", "Burn-in Test", "", "", "", "", ""], ["7.5.7.1", "DC Input Current", "50", "+/-5.000", "A", "", ""], ["7.5.7.2", "Fan Speed", "15100", "+/-200.0", "rpm", "", ""], ["7.5.7.3", "Ambient Temperature", "25", "+/-13.00", "C", "", ""], ["7.5.7.4", "After 10 min of operation", "", "-", "C", "", ""], ["7.5.7.5", "After 20 min of operation", "", "-", "C", "", ""], ["7.5.7.6", "After 30 min of operation", "", "-", "C", "", ""], ["", "", "", "", "", "", ""], ["8", "Auxiliary", "", "", "", "", ""], ["8.1", "Auxiliary Cooling Fan ON", "60", "+/-2.00", "C", "", ""], ["8.2", "Fan status", "ON", "-", "-", "", ""], ["8.3", "Auxiliary Cooling Fan OFF", "55", "+/-2.00", "C", "", ""], ["8.4", "Fan status", "OFF", "-", "-", "", ""], ["", "", "", "", "", "", ""], ["9", "Motor Temp. Test", "", "", "", "", ""], ["9.1", "60 Degree", "60", "+/-3.00", "C", "", ""], ["9.2", "90 Degree", "90", "+/-3.00", "C", "", ""], ["9.3", "120 Degree", "120", "+/-3.00", "C", "", ""]] ("data")
          }
        }
        "UUT" <- w1948
        "UUT" <- w1920
        n711 = for {
          tunnel: w1949 -> [w2030] mode=indexing
          tunnel: w1947 -> [w2028]
          tunnel: [w2027] -> w1917
          tunnel: w1949 -> [w2026]
          i -> [w2029]
          n712 = for {
            tunnel: w2030 -> [_] mode=indexing
            tunnel: w2029 -> [w2036]
            tunnel: w2028 -> [w2033]
            tunnel: [w2032] -> w2027
            tunnel: w2026 -> [w2031]
            i -> [w2037]
            n713 = Bundle By Name(cluster=T21 {"Row"=0, "Column"=0} ("Active Cell:Active Cell"), "Row"=w2036, "Column"=w2037) -> (w2035:T21)
            n714 = control-ref of="ATR"() -> (w2034:refnum<vi>)
            n715 = property class="Tbl (strict)"(reference=w2034, error in=w2033, "Active Cell"=w2035, "Cell BG Color"=u32 16777226, "Value"=w2031) -> (error out=w2032:errorcluster)  [unwired: 1 out]
          }
        }
        n716 = case shown="95" w1920 {
          tunnel: ["AHU Software Version" ("key") "AHU Software Version" ("key") "EBAY Software Version" ("key")] -> w1937
          tunnel: ["AHU R Serial Number" ("key") "AHU L Serial Number" ("key") "EBAY Serial Number" ("key")] -> w1938
          tunnel: [2 2 1] -> w1922
          frame 63, Default {
          }
          frame 47 {
          }
          frame 95 {
          }
        }
        n717 = call <vilib>:"Open Config Data.vi"("error in (no error)"=w1917, "create file if necessary (T)"=FALSE, "configuration file path"=w1931) -> ("error out"=w1932:errorcluster, "refnum"=w1933:T11)  [unwired: 7 out]
        n718 = call-poly <vilib>:"Read Key.vi"("section"=w1935, "error in (no error)"=w1932, "key"=w1937, "refnum"=w1933) -> ("error out"=w1939:errorcluster, "value"=→"UUT SoftwareVer":string, "refnum out"=w1936:T11)  [unwired: 2 in, 3 out]
        n719 = property on="Start" class="Bool (strict)"("DisabledEnum"=w1923) -> ()  [unwired: 2 in, 2 out]
        n720 = property on="Report" class="Bool (strict)"("DisabledEnum"=w1923) -> ()  [unwired: 2 in, 2 out]
        n721 = call-poly <vilib>:"Read Key.vi"("section"=w1935, "error in (no error)"=w1939, "key"=w1938, "refnum"=w1936) -> ("error out"=w1929:errorcluster, "value"=w1927:string, "refnum out"=w1928:T11)  [unwired: 2 in, 3 out]
        n722 = call <vilib>:"Close Config Data.vi"("error in (no error)"=w1929, "refnum"=w1928) -> ("error out"=w1918:errorcluster)  [unwired: 8 in, 1 out]
        n723 = Decimal String To Number(string=w1927) -> (number=w1921:i32)  [unwired: 2 in, 1 out]
        n724 = case shown="63, Default" w1920 {
          tunnel: w1921 -> [w1975 w1988 _]
          tunnel: [w1971 w1984 T10."MainProgram"] -> w1919
          tunnel: w1918 -> [w1970 w1983 w1996]
          tunnel: [w1970 w1983 w1996] -> w1916
          tunnel: [w1969 w1982 FALSE] -> w1914
          frame 63, Default {
            n725 = Quotient & Remainder(x=w1975, y=2) -> (x-y*floor(x/y)=w1973:i32)  [unwired: 1 out]
            n726 = Equal To 0?(x=w1973) -> (x = 0?=w1972:bool)
            n727 = case shown="True" w1972 {
              tunnel: [T10."MainProgram" w1979] -> w1971
              tunnel: [FALSE w1978] -> w1969
              frame False {
              }
              frame True {
                n728 = flat-sequence {
                  tunnel: [T10."Stop"] -> w1979
                  tunnel: [TRUE] -> w1978
                  frame #0 {
                    n729 = call "Display Message to User11"() -> ()  [unwired: 10 in, 2 out]
                  }
                  frame #1 {
                  }
                }
              }
            }
          }
          frame 47 {
            n730 = Quotient & Remainder(x=w1988, y=2) -> (x-y*floor(x/y)=w1986:i32)  [unwired: 1 out]
            n731 = Not Equal To 0?(x=w1986) -> (x != 0?=w1985:bool)
            n732 = case shown="True" w1985 {
              tunnel: [T10."MainProgram" w1992] -> w1984
              tunnel: [FALSE w1991] -> w1982
              frame False {
              }
              frame True {
                n733 = flat-sequence {
                  tunnel: [T10."Stop"] -> w1992
                  tunnel: [TRUE] -> w1991
                  frame #0 {
                    n734 = call "Display Message to User13"() -> ()  [unwired: 10 in, 2 out]
                  }
                  frame #1 {
                  }
                }
              }
            }
          }
          frame 95 {
          }
        }
        n735 = case shown="False" w1914 {
          tunnel: w1916 -> [w1956 w1968]
          tunnel: [w1960 w1968] -> w1915
          frame False {
            n736 = call "Boards S/N"("error in (no error)"=w1956) -> ("POWER Board S/N"=→"POWER Board S/N":string, "DSP Board S/N"=→"DSP Board S/N":string, "error out"=w1957:errorcluster)  [unwired: 15 in, 1 out]
            n737 = call "COM EvolutionBoard.vi"("error in (no error)"=w1957, "VISA resource name 2"=refnum<visa-resource-name> "COM1" ("VISA resource name")) -> ("error out"=w1966:errorcluster, "VISA resource name out"=w1965:refnum<visa-resource-name>)  [unwired: 8 in]
            n738 = call "TesterOption (SubVI).vi"("2 Options"=FALSE, "error in (no error)"=w1966, "On/Off"=FALSE, "Tester Option"=T12."Venable", "VISA Refnum in"=w1965) -> ("error out"=w1960:errorcluster, "VISA Refnum out"=→"VISA Tester":refnum<visa-resource-name>)  [unwired: 5 in]
          }
          frame True {
          }
        }
        n739 = Add(x=w1921, y=w1922) -> (x+y=→"Next SN":i32)
      }
      frame "Stop" {
        n740 = flat-sequence {
          tunnel: w2073 -> [w2111]
          tunnel: [w2110] -> w2066
          frame #0 {
            n741 = control-ref of="Pannel User Message"() -> (w2113:refnum<vi>)
            n742 = property class="Str"(reference=w2113, error in=w2111, "Value"="Program Stopped...\r\nPlease turn OFF All Power sinks") -> (error out=w2110:errorcluster)  [unwired: 1 out]
          }
        }
        n743 = control-ref of="VISA Tester"() -> (w2074:refnum<vi>)
        n744 = property class="VISAName"(reference=w2074, error in=w2066) -> ("Value"=w2072:refnum<visa-resource-name>)  [unwired: 2 out]
        n745 = disable-structure shown="Enabled" {
          disable-tunnel: w2066 -> [w2098 w2099]
          disable-tunnel: w2065 -> [w2096 _]
          disable-tunnel: [w2095 w2099] -> w2052
          frame Disabled {
            n746 = call "Clear CAN Buffer.vi"("error in (no error)"=w2098, "Cluster in"=w2096) -> ("error out"=w2097:errorcluster)  [unwired: 8 in, 1 out]
            n747 = call "Close CAN Device.vi"("error in (no error)"=w2097, "Cluster in"=w2096) -> ("error out"=w2095:errorcluster)  [unwired: 8 in, 1 out]
          }
          frame Enabled {
          }
        }
        n748 = VISA Close(VISA resource name=w2081, error in (no error)=w2066) -> (error out=w2075:errorcluster)
        n749 = property on="Stop Button" class="Bool (strict)"() -> ("Value"=w2044:bool)  [unwired: 2 in, 2 out]
        n750 = call "TesterOption (SubVI).vi"("2 Options"=FALSE, "On/Off"=FALSE, "Tester Option"=T12."Power", "VISA Refnum in"=w2072) -> ("error out"=w2061:errorcluster, "VISA Refnum out"=w2071:refnum<visa-resource-name>)  [unwired: 6 in]
        n751 = property on="ClosePanel" class="Bool (strict)"() -> ("Value"=w2045:bool)  [unwired: 2 in, 2 out]
        n752 = VISA Close(VISA resource name=w2071, error in (no error)=w2061) -> (error out=w2058:errorcluster)
        n753 = Or(x=w2045, y=w2044) -> (x .or. y?=w2043:bool)
        n754 = Flush Queue(queue=w2076, error in (no error)=w2075) -> (queue out=w2078:refnum<queue>, error out=w2077:errorcluster)  [unwired: 1 out]
        n755 = Flush Queue(queue=w2083, error in (no error)=w2075) -> (queue out=w2082:refnum<queue>, error out=w2084:errorcluster)  [unwired: 1 out]
        n756 = case shown="False" w2043 {
          tunnel: w2084 -> [w2086 w2094]
          tunnel: w2082 -> [w2088 w2090]
          tunnel: w2078 -> [w2087 w2089]
          tunnel: w2077 -> [w2085 w2093]
          tunnel: [w2086 w2092] -> w2060
          tunnel: [w2085 w2091] -> w2059
          tunnel: [w2088 w2090] -> w2042
          tunnel: [w2087 w2089] -> w2041
          frame False {
          }
          frame True {
            n757 = Release Queue(queue=w2089, error in (no error)=w2093) -> (error out=w2091:errorcluster)  [unwired: 1 in, 2 out]
            n758 = Release Queue(queue=w2090, error in (no error)=w2094) -> (error out=w2092:errorcluster)  [unwired: 1 in, 2 out]
          }
        }
        n759 = Merge Errors(w2060, w2059, w2058, w2052) -> (w2057:errorcluster)
        n760 = property on="Refresh Button" class="Bool (strict)"() -> ("Value"=w2046:bool)  [unwired: 2 in, 2 out]
        n761 = call <vilib>:"Clear Errors.vi"("error in (no error)"=w2057) -> ("error out"=w2056:errorcluster)  [unwired: 5 in, 1 out]
        n762 = property on="Stop Button" class="Bool (strict)"() -> ("Value"=w2050:bool)  [unwired: 2 in, 2 out]
        n763 = property on="ClosePanel" class="Bool (strict)"(error in=w2056) -> (error out=w2054:errorcluster, "Value"=w2055:bool)  [unwired: 1 in, 1 out]
        n764 = Not(x=w2046) -> (.not. x?=w2047:bool)
        n765 = Select(t=T10."Initialize", s=w2046, f=T10."Stop") -> (s? t:f=w2062:T10)
        n766 = Not(x=w2050) -> (.not. x?=w2049:bool)
        n767 = Compound Arithmetic op=AND(w2055, w2049, w2047) -> (w2051:bool)
        n768 = case shown="False" w2051 {
          tunnel: w2054 -> [w2102 w2106]
          tunnel: [w2102 w2106] -> w2053
          tunnel: [w2101 w2105] -> w2048
          tunnel: w2046 -> [w2100 _]
          frame False {
            n769 = case shown="False" w2100 {
              tunnel: [TRUE FALSE] -> w2101
              frame False {
              }
              frame True {
              }
            }
          }
          frame True {
            n770 = flat-sequence {
              tunnel: [TRUE] -> w2105
              frame #0 {
              }
              frame #1 {
                n771 = control-ref of="This VI"() -> (w2109:refnum<vi>)
                n772 = property class="VI"(reference=w2109, "FP.State"=T22."Closed" ("Front Panel Window:State")) -> ()  [unwired: 1 in, 2 out]
              }
            }
          }
        }
      }
      frame "MainProgram" {
        n773 = event shown="[0] Timeout" {
          selector: w2122 -> [_ _ _ _ _ _ _ _ _ _ _ _ _]
          dyn-events: _ -> [_ _ _ _ _ _ _ _ _ _ _ _ _]
          timeout: 70 -> [_ _ _ _ _ _ _ _ _ _ _ _ _]
          tunnel: [T10."MainProgram" T10."MainProgram" T10."MainProgram" T10."MainProgram" T10."MainProgram" T10."Stop" T10."MainProgram" w2759 T10."MainProgram" T10."MainProgram" T10."MainProgram" T10."Stop" T10."MainProgram"] -> w2135
          tunnel: [w2152 w2251 w2322 w2330 w2340 w2359 w2385 w2807 w2877 w2891 w2902 w2989 w2996] -> w2129
          tunnel: w2133 -> [w2164 w2251 w2321 w2332 w2340 w2359 w2392 w2807 w2878 w2890 w2898 w2989 w3001]
          tunnel: [w2172 w2245 w2323 w2331 w2341 w2357 w2381 w2764 w2875 w2888 w2903 w2987 w2994] -> w2130
          tunnel: w2131 -> [w2172 w2245 w2323 w2331 w2341 w2357 w2381 w2764 w2875 w2888 _ w2987 w2994]
          tunnel: w2128 -> [w2166 w2257 w2317 w2327 w2337 w2356 w2390 w2791 w2874 w2887 w2906 w2986 w2999]
          tunnel: w2127 -> [w2161 w2256 w2318 w2328 w2338 w2355 w2363 w2790 w2873 w2886 w2905 w2985 w2992]
          tunnel: [w2163 w2256 w2318 w2328 w2338 w2355 w2363 w2790 w2873 w2886 w2905 w2985 w2992] -> w2126
          tunnel: [w2165 w2257 w2317 w2327 w2337 w2356 w2390 w2791 w2874 w2887 w2906 w2986 w2999] -> w2125
          tunnel: w2124 -> [w2159 w2255 w2316 w2326 w2336 w2354 w2389 w2789 w2872 w2885 w2904 w2984 w2998]
          tunnel: [w2159 w2255 w2316 w2326 w2336 w2354 w2384 w2789 w2872 w2885 w2904 w2984 w2998] -> w2123
          tunnel: w2121 -> [_ _ _ _ _ _ _ w2732 _ _ _ _ _]
          tunnel: w2120 -> [w2160 w2254 w2315 w2325 w2335 w2352 w2379 w2768 w2871 w2884 w2900 w2983 w2997]
          tunnel: [w2160 w2254 w2315 w2325 w2335 w2352 w2379 w2767 w2871 w2884 w2900 w2983 w2997] -> w2119
          tunnel: w2118 -> [_ w2252 _ _ _ _ _ w2766 _ _ _ _ _]
          tunnel: w2117 -> [_ w2244 _ _ _ _ _ _ _ _ _ _ _]
          tunnel: w2116 -> [_ _ _ _ _ _ _ _ w2870 _ _ _ _]
          tunnel: w2115 -> [w2137 w2225 w2314 w2324 w2334 w2349 w2362 w2725 w2868 w2883 w2895 w2982 w2990]
          tunnel: [w2136 w2225 w2314 w2324 w2334 w2349 w2362 w2725 w2868 w2883 w2895 w2982 w2990] -> w2114
          event Timeout {
            n774 = event-data() -> ()  [unwired: 1 in, 3 out]
            n775 = property class="Clust (strict)"(reference=w2161, error in=w2164) -> (reference out=w2163:refnum<vi>, error out=w2162:errorcluster, "Value"=w2169:T7)
            n776 = Unbundle By Name(w2169) -> ("DevType"=w2170:T2, "CanIndex"=w2168:T1)
            n777 = property on="ClosePanel" class="Bool (strict)"("Value"=FALSE ("ClosePanel")) -> ()  [unwired: 2 in, 2 out]
            n778 = call "VCI_Receive.vi"("CANIndex"=w2168, "DevIndex"=u32 0, "DevType"=w2170) -> ("Recieve"=w2167:T26[])  [unwired: 3 in, 5 out]
            n779 = Empty Array?(array=w2167) -> (empty?=w2154:bool)
            n780 = case shown="True" w2154 {
              tunnel: w2168 -> [w2187 _]
              tunnel: w2163 -> [w2185 _]
              tunnel: w2166 -> [w2184 w2224]
              tunnel: w2162 -> [w2183 w2223]
              tunnel: w2167 -> [w2188 _]
              tunnel: [w2178 w2223] -> w2152
              tunnel: [w2177 w2224] -> w2165
              tunnel: [TRUE w2218] -> w2151
              tunnel: w2137 -> [_ w2222]
              tunnel: [0 w2221] -> w2136
              frame False {
                n781 = call "Demo_MakeDispBuff.vi"("Channel"=w2187, "Type"=enum16{"接收", "发送"}."接收", "OBJs"=w2188) -> ("Buffer"=w2186:T27)
                n782 = for {
                  N: 3 -> [_]
                  tunnel: w2186 -> [w2202]
                  tunnel: w2185 -> [w2201]
                  tunnel: w2184 -> [w2192]
                  tunnel: w2183 -> [w2191]
                  tunnel: [w2194] -> w2181 mode=indexing
                  tunnel: [w2192] -> w2180
                  tunnel: [w2191] -> w2179
                  i -> [w2190]
                  n783 = property class="Clust (strict)"(reference=w2201) -> ("Value"=w2199:T7)  [unwired: 1 in, 2 out]
                  n784 = Index Array(array=w2202, index=w2190) -> (element=w2195:T28)
                  n785 = Unbundle By Name(w2195) -> ("Channel"=w2197:T1, "VCI_CAN_OBJ"=w2200:T26)  [unwired: 2 out]
                  n786 = Unbundle By Name(w2199) -> ("CanIndex"=w2198:T1)
                  n787 = Equal?(x=w2198, y=w2197) -> (x = y?=w2196:bool)
                  n788 = case shown="True" w2196 {
                    tunnel: w2200 -> [_ w2213]
                    tunnel: [w2203 w2209] -> w2194
                    tunnel: T23 {"ID"=0, "MSGTYPE"=0, "LEN"=0, "aDATA"=[]} ("Msg") -> [w2203 w2208]
                    frame False {
                    }
                    frame True {
                      n789 = Unbundle By Name(w2213) -> ("ID"=w2207:u32, "DataLen"=w2212:u8, "Data"=w2210:u8[])
                      n790 = Bundle By Name(cluster=w2208, "ID"=w2207, "MSGTYPE"=u8 0, "LEN"=w2212, "aDATA"=w2210) -> (w2209:T23)
                      n791 = Unbundle By Name(w2209) -> ("ID"=w2205:u32)
                      n792 = Split Number(x=w2205) -> (lo(x)=w2206:u16)  [unwired: 1 out]
                      n793 = Split Number(x=w2206) -> (lo(x)=w2204:u8)  [unwired: 1 out]
                      n794 = case shown="63" w2204 {
                        tunnel: ["EBAY 5F" "" "AHU 3F" "AHU 2F"] -> _
                        frame 95 {
                        }
                        frame Default {
                        }
                        frame 63 {
                        }
                        frame 47 {
                        }
                      }
                    }
                  }
                }
                n795 = Enqueue Element(queue=w2180, element=w2181, error in (no error)=w2179) -> (queue out=w2177:refnum<queue>, error out=w2178:errorcluster)  [unwired: 2 out]
              }
              frame True {
                n796 = Increment(x=w2222) -> (x+1=w2221:i32)
                n797 = Greater Or Equal?(x=w2221, y=30 ("x")) -> (x >= y?=w2219:bool)
                n798 = Not(x=w2219) -> (.not. x?=w2218:bool)
              }
            }
            n799 = control-ref of="ATR"() -> (w2153:refnum<vi>)
            n800 = property on="CAN Status" class="Bool (strict)"("Value"=w2151) -> ()  [unwired: 2 in, 2 out]
            n801 = call <vilib>:"Application Directory.vi"() -> ("Application Directory"=w2145:path)
            n802 = call "PassFailUUT (SubVI).vi"("error in (no error)"=w2152, "Table in"=w2153) -> ("PassFaileUUTresult"=w2141:bool)  [unwired: 7 in, 2 out]
            n803 = Select(t="PASS" ("name or relative path"), s=w2141, f="FAIL" ("name or relative path")) -> (s? t:f=w2138:string)
            n804 = Build Path(base path=w2145, name or relative path="data\\TestResult.ini") -> (appended path=w2149:path)
            n805 = property on="Test Failed" class="Bool (strict)"("Value"=w2141) -> ()  [unwired: 2 in, 2 out]
            n806 = call <vilib>:"Open Config Data.vi"("configuration file path"=w2149) -> ("error out"=w2147:errorcluster, "refnum"=w2148:T11)  [unwired: 2 in, 7 out]
            n807 = property on="Automation" class="Bool (strict)"() -> ("Value"=w2156:bool)  [unwired: 2 in, 2 out]
            n808 = call-poly <vilib>:"Write Key.vi"("section"="Marvin", "error in (no error)"=w2147, "value"=w2138, "key"="Result", "refnum"=w2148) -> ("error out"=w2144:errorcluster, "refnum out"=w2143:T11)  [unwired: 4 in, 1 out]
            n809 = property on="Start" class="Bool (strict)"() -> ("Value"=w2158:bool)  [unwired: 2 in, 2 out]
            n810 = Or(x=w2156, y=w2158) -> (x .or. y?=w2157:bool)
            n811 = call <vilib>:"Close Config Data.vi"("error in (no error)"=w2144, "refnum"=w2143) -> ()  [unwired: 8 in, 2 out]
            n812 = case shown="False" w2157 {
              frame False {
                n813 = property on="Pannel User Message" class="Str"("Value"="You can press start to execute(s) test(s).") -> ()  [unwired: 2 in, 2 out]
              }
              frame True {
              }
            }
          }
          event "SetSN": Value Change {
            n814 = event-data() -> ()  [unwired: 1 in, 6 out]
            n815 = property on="UUT" class="DigNum (strict)"() -> ("Value"=w2235:u8)  [unwired: 2 in, 2 out]
            n816 = Equal?(x=w2235, y=u8 95) -> (x = y?=w2233:bool)
            n817 = control-ref of="ATR"() -> (w2236:refnum<vi>)
            n818 = Select(t=u8 50 ("y"), s=w2233, f=u8 36 ("y")) -> (s? t:f=w2228:u8)
            n819 = property on="Current SN" class="DigNum (strict)"(error in=w2251) -> (error out=w2230:errorcluster, "Value"=w2250:i32)  [unwired: 1 in, 1 out]
            n820 = call "PassFailUUT (SubVI).vi"("error in (no error)"=w2230, "Table in"=w2236) -> ("Total Pass"=w2229:u8)  [unwired: 7 in, 2 out]
            n821 = Equal To 0?(x=w2250) -> (x = 0?=w2247:bool)
            n822 = Equal?(x=w2250, y=-1) -> (x = y?=w2248:bool)
            n823 = Equal?(x=w2229, y=w2228) -> (x = y?=w2227:bool)
            n824 = Or(x=w2248, y=w2247) -> (x .or. y?=w2246:bool)
            n825 = property on="CAN Status" class="Bool (strict)"() -> ("Value"=w2237:bool)  [unwired: 2 in, 2 out]
            n826 = property on="Status" class="Bool (strict)"() -> ("Value"=w2242:bool)  [unwired: 2 in, 2 out]
            n827 = And(x=w2242, y=w2237) -> (x .and. y?=w2238:bool)
            n828 = case shown="True" w2238 {
              tunnel: w2252 -> [_ w2271]
              tunnel: w2246 -> [_ w2260]
              tunnel: w2245 -> [_ w2270]
              tunnel: w2244 -> [_ w2269]
              tunnel: [errorcluster {"status"=FALSE, "code"=0, "source"=""} ("error out") w2268] -> w2241
              tunnel: [w2258 w2267] -> w2243
              tunnel: w2227 -> [_ w2261]
              frame False {
                w2258 = FALSE ("Value")
                n829 = property on="SetSN" class="Bool (strict)"("Value"=w2258) -> ()  [unwired: 2 in, 2 out]
                n830 = call "Display Message to User10"() -> ()  [unwired: 10 in, 2 out]
              }
              frame True {
                n831 = property on="Test Failed" class="Bool (strict)"() -> ("Value"=w2265:bool)  [unwired: 2 in, 2 out]
                n832 = property on="Automation" class="Bool (strict)"() -> ("Value"=w2267:bool)  [unwired: 2 in, 2 out]
                n833 = Not(x=w2265) -> (.not. x?=w2266:bool)
                n834 = Select(t=w2266, s=w2267, f=w2269) -> (s? t:f=w2263:bool)
                n835 = Or(x=w2261, y=w2263) -> (x .or. y?=w2262:bool)
                n836 = And(x=w2260, y=w2262) -> (x .and. y?=w2264:bool)
                n837 = case shown="True" w2264 {
                  tunnel: w2271 -> [_ w2302]
                  tunnel: w2270 -> [_ w2295]
                  tunnel: [w2273 w2287] -> w2268
                  tunnel: w2260 -> [w2272 _]
                  frame False {
                    n838 = case shown="True" w2272 {
                      tunnel: [w2275 w2276] -> w2273
                      frame False {
                        n839 = call "Display Message to User9"() -> ("error out"=w2275:errorcluster)  [unwired: 10 in, 1 out]
                      }
                      frame True {
                        n840 = call "Display Message to User3"() -> ("error out"=w2276:errorcluster)  [unwired: 10 in, 1 out]
                      }
                    }
                    n841 = property on="Automation" class="Bool (strict)"(error in=w2273, "Value"=FALSE ("Automation")) -> ()  [unwired: 1 in, 2 out]
                  }
                  frame True {
                    w2294 = FALSE ("SetSN")
                    n842 = property on="Next SN" class="DigNum (strict)"() -> ("Value"=w2278:i32)  [unwired: 2 in, 2 out]
                    n843 = property on="VISA Tester" class="VISAName"() -> ("Value"=w2285:refnum<visa-resource-name>)  [unwired: 2 in, 2 out]
                    n844 = call "TesterOption (SubVI).vi"("2 Options"=FALSE, "On/Off"=FALSE, "Tester Option"=T12."Venable", "VISA Refnum in"=w2285) -> ("error out"=w2280:errorcluster)  [unwired: 6 in, 1 out]
                    n845 = call <vilib>:"Clear Errors.vi"("error in (no error)"=w2280) -> ("error out"=w2281:errorcluster)  [unwired: 5 in, 1 out]
                    n846 = Number To Decimal String(number=w2278) -> (decimal integer string=w2279:string)  [unwired: 1 in]
                    "UUT SN Report" <- w2279
                    n847 = Search and Replace String(input string="EP=1\r\nSN=0\r\n" ("write buffer"), search string="0", replace string=w2279) -> (result string=w2297:string)  [unwired: 5 in, 3 out]
                    n848 = call "SerialMarvinSendGet.vi"("error in (no error)"=w2281, "Clear Log"=FALSE, "write buffer"=w2297, "VISA resource name"=w2295) -> ("error out"=w2286:errorcluster)  [unwired: 6 in, 1 out]
                    n849 = property on="UUT" class="DigNum (strict)"(error in=w2286) -> ("Value"=w2303:u8)  [unwired: 1 in, 2 out]
                    n850 = case shown="47" w2303 {
                      tunnel: ["AHU R Serial Number" ("key") "AHU L Serial Number" ("key") "EBAY Serial Number" ("key")] -> w2306
                      tunnel: [2 2 1] -> w2277
                      frame 63, Default {
                      }
                      frame 47 {
                      }
                      frame 95 {
                      }
                    }
                    n851 = call <vilib>:"Open Config Data.vi"("create file if necessary (T)"=FALSE, "configuration file path"=w2302) -> ("error out"=w2300:errorcluster, "refnum"=w2301:T11)  [unwired: 1 in, 7 out]
                    n852 = call-poly <vilib>:"Write Key.vi"("section"="Marvin", "error in (no error)"=w2300, "value"=w2279, "key"=w2306, "refnum"=w2301) -> ("error out"=w2290:errorcluster, "refnum out"=w2289:T11)  [unwired: 4 in, 1 out]
                    n853 = call <vilib>:"Close Config Data.vi"("error in (no error)"=w2290, "refnum"=w2289) -> ("error out"=w2288:errorcluster)  [unwired: 8 in, 1 out]
                    n854 = property on="Current SN" class="DigNum (strict)"("Value"=w2278) -> ()  [unwired: 2 in, 2 out]
                    n855 = property on="SetSN" class="Bool (strict)"(error in=w2288, "Value"=w2294) -> (error out=w2293:errorcluster)  [unwired: 1 in, 1 out]
                    n856 = property on="Automation" class="Bool (strict)"(error in=w2293, "Value"=w2294) -> (error out=w2292:errorcluster)  [unwired: 1 in, 1 out]
                    n857 = Add(x=w2278, y=w2277) -> (x+y=w2291:i32)
                    n858 = property on="Next SN" class="DigNum (strict)"(error in=w2292, "Value"=w2291) -> (error out=w2287:errorcluster)  [unwired: 1 in, 1 out]
                  }
                }
              }
            }
            n859 = call <vilib>:"Clear Errors.vi"("error in (no error)"=w2241) -> ("error out"=w2226:errorcluster)  [unwired: 5 in, 1 out]
            n860 = property on="SetSN" class="Bool (strict)"(error in=w2226, "Value"=FALSE ("SetSN")) -> (error out=w2240:errorcluster)  [unwired: 1 in, 1 out]
            n861 = case shown="True" w2243 {
              tunnel: w2240 -> [_ _]
              frame False {
              }
              frame True {
                w2313 = TRUE ("Value (Signaling)")
                n862 = property on="Report" class="Bool (strict)"("Val(Sgnl)"=w2313, "Value"=w2313) -> ()  [unwired: 2 in, 2 out]
              }
            }
          }
          event "ATR": Mouse Enter {
            n863 = event-data() -> ()  [unwired: 1 in, 4 out]
            n864 = call-poly <vilib>:"Set Cursor.vi"("error in (no error)"=w2321, "icon"=u16 1) -> ("error out"=w2322:errorcluster)  [unwired: 8 in, 1 out]
          }
          event "ATR": Mouse Leave {
            n865 = event-data() -> ()  [unwired: 1 in, 4 out]
            n866 = call-poly <vilib>:"Set Cursor.vi"("error in (no error)"=w2332, "icon"=u16 0) -> ("error out"=w2330:errorcluster)  [unwired: 8 in, 1 out]
          }
          event "ATR": Mouse Down? {
            n867 = event-data() -> ("Coords"=w2348:T29)  [unwired: 1 in, 4 out]
            n868 = invoke on="ATR" class="Tbl (strict)" method="Point To Row Column"("Point"=w2348) -> ("InBounds"=w2344:bool, "CellPosition"=w2343:T21)  [unwired: 5 in, 4 out]
            n869 = Greater Than 0?(x=w2343) -> (x > 0?=w2347:cluster{"Row":bool, "Column":bool})
            n870 = Cluster To Array(cluster=w2347) -> (array=w2346:bool[])
            n871 = Or Array Elements(Boolean array=w2346) -> (logical OR=w2345:bool)
            n872 = Or(x=w2344, y=w2345) -> (x .or. y?=w2342:bool)
            n873 = event-data("Discard?"=w2342) -> ()  [unwired: 1 in, 1 out]
          }
          event Panel Close? {
            n874 = event-data() -> ("VIRef"=w2353:refnum<vi>)  [unwired: 1 in, 3 out]
            n875 = Close Reference(reference=w2353) -> ()  [unwired: 1 in, 1 out]
            n876 = disable-structure shown="Disabled" {
              frame Disabled {
                n877 = property on="Stop Button" class="Bool (strict)"("Val(Sgnl)"=TRUE ("Stop Button"), "Value"=FALSE ("Stop Button")) -> ()  [unwired: 2 in, 2 out]
              }
              frame Enabled {
              }
            }
            n878 = event-data("Discard?"=TRUE) -> ()  [unwired: 1 in, 1 out]
            "ClosePanel" <- TRUE ("ClosePanel")
          }
          event "Start": Value Change {
            w2380 = T17 [] items=["Auxiliary", "Temp Sens Cal", "Com Test", "Enable Test", "Speed Command", "Stop Time", "Temp Control", "Burn in", "Visual Inspec", "Empty"]
            n879 = event-data() -> ()  [unwired: 1 in, 2 out]
            n880 = property on="VISA Tester" class="VISAName"() -> ("Value"=w2378:refnum<visa-resource-name>)  [unwired: 2 in, 2 out]
            n881 = property on="UUT" class="Str"(error in=w2392) -> (error out=w2374:errorcluster, "Value"=w2391:string)  [unwired: 1 in, 1 out]
            n882 = control-ref of="Pannel User Message"() -> (w2371:refnum<vi>)
            n883 = control-ref of="Motor Speed RPM"() -> (w2366:refnum<vi>)
            n884 = call "TesterOption (SubVI).vi"("2 Options"=FALSE, "error in (no error)"=w2374, "On/Off"=FALSE, "Tester Option"=T12."Venable", "VISA Refnum in"=w2378) -> ("error out"=w2373:errorcluster)  [unwired: 5 in, 1 out]
            n885 = control-ref of="Stop Burn-in"() -> (w2369:refnum<vi>)
            n886 = control-ref of="Stop Button"() -> (w2370:refnum<vi>)
            n887 = call "Write panel message (SubVI).vi"("Stop BurnIn"=w2369, 4:"rpm"=w2366, 5:"rpm"=FALSE ("rpm"), "PrintTime"=TRUE, "Stop"=w2370, "error in (no error)"=w2373, "Time to wait"=5.0, "Strin"="TESTER BIT TEST OPERATION IN PROCESS", "String in"=w2371) -> ("error out"=w2372:errorcluster)  [unwired: 2 in]
            n888 = while {
              tunnel: w2391 -> [w2420]
              tunnel: [w2419] -> w2387
              tunnel: [w2418] -> w2386
              shift-right: [w2415] -> _
              shift-left: enum16{"Stop", "Tests", "Bit test", "Start"}."Start" -> [w2417]
              tunnel: w2381 -> [w2416]
              tunnel: w2380 -> [w2414]
              tunnel: w2372 -> [w2399]
              tunnel: w2370 -> [w2408]
              tunnel: w2369 -> [w2407]
              tunnel: w2371 -> [w2406]
              tunnel: w2366 -> [w2405]
              tunnel: w2363 -> [w2398]
              stop <- w2413 stop-if-true
              n889 = property class="Clust (strict)"(reference=w2398, error in=w2399) -> ("Value"=w2401:T7)  [unwired: 2 out]
              n890 = Unbundle By Name(w2401) -> ("DevType"=w2403:T2, "CanIndex"=w2402:T1)
              n891 = property on="VISA Tester" class="VISAName"() -> ("Value"=w2411:refnum<visa-resource-name>)  [unwired: 2 in, 2 out]
              n892 = call "VCI_Receive.vi"("CANIndex"=w2402, "DevIndex"=u32 0, "DevType"=w2403) -> ("Recieve"=w2404:T26[])  [unwired: 3 in, 5 out]
              n893 = Empty Array?(array=w2404) -> (empty?=w2397:bool)
              n894 = Not(x=w2397) -> (.not. x?=w2396:bool)
              n895 = property on="CAN Status" class="Bool (strict)"("Value"=w2396) -> (error out=w2395:errorcluster)  [unwired: 2 in, 1 out]
              n896 = property on="CAN Status" class="Bool (strict)"(error in=w2395) -> (error out=w2394:errorcluster, "Value"=w2409:bool)  [unwired: 1 in, 1 out]
              n897 = property on="Status" class="Bool (strict)"(error in=w2394) -> (error out=w2410:errorcluster, "Value"=w2412:bool)  [unwired: 1 in, 1 out]
              n898 = case shown="\"Bit test\"" w2417 {
                tunnel: w2420 -> [_ w2436 w2556 _]
                tunnel: [w2425 w2435 w2584 w2691] -> w2419
                tunnel: [w2421 w2434 w2554 w2683] -> w2418
                tunnel: w2416 -> [_ _ w2569 w2696]
                tunnel: w2406 -> [_ _ _ w2695]
                tunnel: w2408 -> [_ _ _ w2694]
                tunnel: w2407 -> [_ _ _ w2693]
                tunnel: w2405 -> [_ _ _ w2692]
                tunnel: [w2424 w2433 w2559 w2687] -> w2415
                tunnel: w2414 -> [w2425 _ w2584 w2691]
                tunnel: [w2423 w2432 FALSE FALSE] -> w2413
                tunnel: w2412 -> [_ _ _ w2689]
                tunnel: w2411 -> [_ _ w2570 _]
                tunnel: w2410 -> [w2421 _ _ _]
                tunnel: w2409 -> [_ _ _ w2684]
                frame "Stop", Default {
                  n899 = property on="Start" class="Bool (strict)"(error in=w2421, "Value"=FALSE ("Start")) -> ()  [unwired: 1 in, 2 out]
                  n900 = flat-sequence {
                    tunnel: [enum16{"Stop", "Tests", "Bit test", "Start"}."Stop"] -> w2424
                    tunnel: w2421 -> [_]
                    tunnel: [TRUE] -> w2423
                    frame #0 {
                    }
                  }
                }
                frame "Tests" {
                  w2430 = FALSE ("Stop Burn-in")
                  w2431 = T20."Disabled and Grayed Out" ("Disabled")
                  n901 = case shown="\"AHU\", Default" w2436 {
                    tunnel: [w2452 w2501] -> w2435
                    tunnel: [w2451 w2500] -> w2434
                    tunnel: [w2440 w2488] -> w2428
                    frame "AHU", Default {
                      n902 = call "Load Program Process AHU.vi"() -> ("Speed Command Test"=w2445:bool, "Enable Test"=w2446:bool, "Burn-in Test"=w2443:bool, "Auxiliary"=w2441:bool, "Temperature Sensor Calibration Test"=w2448:bool, "Communication Test"=w2447:bool, "Stop Time Test"=w2444:bool, "Visual Inspection"=w2442:bool, "OK"=w2449:bool, "Automation"=w2440:bool, "error out"=w2451:errorcluster)  [unwired: 8 in, 9 out]
                      n903 = Or(x=w2449, y=w2440) -> (x .or. y?=w2450:bool)
                      n904 = case shown="True" w2450 {
                        tunnel: [w2453 w2463] -> w2452
                        tunnel: w2440 -> [_ w2462]
                        tunnel: w2448 -> [_ w2461]
                        tunnel: w2447 -> [_ w2460]
                        tunnel: w2446 -> [_ w2459]
                        tunnel: w2445 -> [_ w2458]
                        tunnel: w2444 -> [_ w2457]
                        tunnel: w2443 -> [_ w2456]
                        tunnel: w2442 -> [_ w2455]
                        tunnel: w2441 -> [_ w2454]
                        frame False {
                          w2453 = T17 [] items=["Auxiliary", "Temp Sens Cal", "Com Test", "Enable Test", "Speed Command", "Stop Time", "Temp Control", "Burn in", "Visual Inspec", "Empty"]
                        }
                        frame True {
                          n905 = case shown="False" w2462 {
                            tunnel: [w2486 w2487] -> w2463
                            tunnel: w2461 -> [w2468 _]
                            tunnel: w2460 -> [w2467 _]
                            tunnel: w2459 -> [w2469 _]
                            tunnel: w2458 -> [w2466 _]
                            tunnel: w2457 -> [w2465 _]
                            tunnel: w2456 -> [w2479 _]
                            tunnel: w2455 -> [w2464 _]
                            tunnel: w2454 -> [_ _]
                            frame False {
                              w2472 = T24."Empty" ("f")
                              n906 = Select(t=T24."Com Test" ("f"), s=w2467, f=w2472) -> (s? t:f=w2478:T24)
                              n907 = Select(t=T24."Temp Sens Cal" ("f"), s=w2468, f=w2472) -> (s? t:f=w2477:T24)
                              n908 = Select(t=T24."Stop Time" ("f"), s=w2465, f=w2472) -> (s? t:f=w2476:T24)
                              n909 = Select(t=T24."Enable Test" ("f"), s=w2469, f=w2472) -> (s? t:f=w2475:T24)
                              n910 = Select(t=T24."Speed Command" ("f"), s=w2466, f=w2472) -> (s? t:f=w2474:T24)
                              n911 = Select(t=T24."Burn in" ("f"), s=w2479, f=w2472) -> (s? t:f=w2473:T24)
                              n912 = Select(t=T24."Visual Inspec" ("f"), s=w2464, f=w2472) -> (s? t:f=w2470:T24)
                              n913 = Build Array(w2478, w2477, w2476, w2475, w2474, w2473, w2470) -> (w2486:T17)
                            }
                            frame True {
                              w2487 = T17 [enum."Com Test", enum."Temp Sens Cal", enum."Stop Time", enum."Enable Test", enum."Speed Command", enum."Burn in", enum."Visual Inspec"] items=["Auxiliary", "Temp Sens Cal", "Com Test", "Enable Test", "Speed Command", "Stop Time", "Temp Control", "Burn in", "Visual Inspec", "Empty"]
                            }
                          }
                        }
                      }
                    }
                    frame "EBAY" {
                      n914 = call "Load Program Process EBAY.vi"() -> ("Speed Command Test"=w2494:bool, "Enable Test"=w2495:bool, "Burn-in Test"=w2492:bool, "Temperature Control Algorithm Test"=w2491:bool, "Auxiliary"=w2489:bool, "Temperature Sensor Calibration Test"=w2497:bool, "Communication Test"=w2496:bool, "Stop Time Test"=w2493:bool, "Visual Inspection"=w2490:bool, "OK"=w2498:bool, "Automation"=w2488:bool, "error out"=w2500:errorcluster)  [unwired: 8 in, 8 out]
                      n915 = Or(x=w2498, y=w2488) -> (x .or. y?=w2499:bool)
                      n916 = case shown="True" w2499 {
                        tunnel: [w2502 w2513] -> w2501
                        tunnel: w2488 -> [_ w2512]
                        tunnel: w2497 -> [_ w2511]
                        tunnel: w2496 -> [_ w2510]
                        tunnel: w2495 -> [_ w2509]
                        tunnel: w2494 -> [_ w2508]
                        tunnel: w2493 -> [_ w2507]
                        tunnel: w2492 -> [_ w2506]
                        tunnel: w2491 -> [_ w2505]
                        tunnel: w2490 -> [_ w2504]
                        tunnel: w2489 -> [_ w2503]
                        frame False {
                          w2502 = T17 [] items=["Auxiliary", "Temp Sens Cal", "Com Test", "Enable Test", "Speed Command", "Stop Time", "Temp Control", "Burn in", "Visual Inspec", "Empty"]
                        }
                        frame True {
                          n917 = case shown="False" w2512 {
                            tunnel: [w2542 w2543] -> w2513
                            tunnel: w2511 -> [w2518 _]
                            tunnel: w2510 -> [w2517 _]
                            tunnel: w2509 -> [w2516 _]
                            tunnel: w2508 -> [w2515 _]
                            tunnel: w2507 -> [w2514 _]
                            tunnel: w2506 -> [w2520 _]
                            tunnel: w2505 -> [w2519 _]
                            tunnel: w2504 -> [w2533 _]
                            tunnel: w2503 -> [w2524 _]
                            frame False {
                              w2522 = T24."Empty" ("f")
                              n918 = Select(t=T24."Com Test" ("f"), s=w2517, f=w2522) -> (s? t:f=w2532:T24)
                              n919 = Select(t=T24."Temp Sens Cal" ("f"), s=w2518, f=w2522) -> (s? t:f=w2531:T24)
                              n920 = Select(t=T24."Stop Time" ("f"), s=w2514, f=w2522) -> (s? t:f=w2530:T24)
                              n921 = Select(t=T24."Enable Test" ("f"), s=w2516, f=w2522) -> (s? t:f=w2529:T24)
                              n922 = Select(t=T24."Speed Command" ("f"), s=w2515, f=w2522) -> (s? t:f=w2528:T24)
                              n923 = Select(t=T24."Temp Control" ("f"), s=w2519, f=w2522) -> (s? t:f=w2527:T24)
                              n924 = Select(t=T24."Burn in" ("f"), s=w2520, f=w2522) -> (s? t:f=w2526:T24)
                              n925 = Select(t=T24."Visual Inspec" ("f"), s=w2533, f=w2522) -> (s? t:f=w2525:T24)
                              n926 = Select(t=T24."Auxiliary" ("f"), s=w2524, f=w2522) -> (s? t:f=w2521:T24)
                              n927 = Build Array(w2532, w2531, w2530, w2529, w2528, w2527, w2526, w2521, w2525) -> (w2542:T17)
                            }
                            frame True {
                              w2543 = T17 [enum."Com Test", enum."Temp Sens Cal", enum."Stop Time", enum."Enable Test", enum."Speed Command", enum."Temp Control", enum."Burn in", enum."Auxiliary", enum."Visual Inspec"] items=["Auxiliary", "Temp Sens Cal", "Com Test", "Enable Test", "Speed Command", "Stop Time", "Temp Control", "Burn in", "Visual Inspec", "Empty"]
                            }
                          }
                        }
                      }
                    }
                  }
                  "Automation" <- w2428
                  n928 = control-ref of="ATR"() -> (w2429:refnum<vi>)
                  n929 = flat-sequence {
                    tunnel: [enum16{"Stop", "Tests", "Bit test", "Start"}."Tests"] -> w2433
                    tunnel: [TRUE] -> w2432
                    frame #0 {
                    }
                  }
                  n930 = case shown="True" w2428 {
                    tunnel: w2429 -> [_ w2437]
                    frame False {
                    }
                    frame True {
                      n931 = call "ResetTable Result (SubVI).vi"("Table in"=w2437) -> ()  [unwired: 11 in]
                    }
                  }
                  n932 = property on="Stop Button" class="Bool (strict)"("Value"=w2430) -> ()  [unwired: 2 in, 2 out]
                  n933 = property on="Stop Burn-in" class="Bool (strict)"("Value"=w2430) -> ()  [unwired: 2 in, 2 out]
                  n934 = property on="Start" class="Bool (strict)"("DisabledEnum"=w2431) -> ()  [unwired: 2 in, 2 out]
                  n935 = property on="Report" class="Bool (strict)"("DisabledEnum"=w2431) -> ()  [unwired: 2 in, 2 out]
                }
                frame "Bit test" {
                  # "Stop"
                  n936 = call "SerialMarvinSendGet.vi"("write buffer"="TA[1]\r\n", "VISA resource name"=w2569) -> ("error out"=w2580:errorcluster, "read buffer"=w2581:string)  [unwired: 8 in]
                  n937 = Fract/Exp String To Number(string=w2581) -> (number=w2549:dbl)  [unwired: 3 in, 1 out]
                  n938 = call "TAs StartTest (SubVI).vi"("Numeric"=w2549, "Enum"=enum16{"TA3", "TA2", "TA1"}."TA1") -> ("String Out"=w2548:string, "Result"=w2550:bool)  [unwired: 7 in, 1 out]
                  n939 = call "TesterOption (SubVI).vi"("On/Off 2"=FALSE, "Tester Option 2"=T12."Venable", "2 Options"=TRUE, "error in (no error)"=w2580, "On/Off"=TRUE, "Tester Option"=T12."25C", "VISA Refnum in"=w2570) -> ("error out"=w2572:errorcluster)  [unwired: 3 in, 1 out]
                  n940 = call "Time Delay5"("error in (no error)"=w2572) -> ("error out"=w2571:errorcluster)  [unwired: 10 in]
                  n941 = call "SerialMarvinSendGet.vi"("error in (no error)"=w2571, "write buffer"="TA[2]\r\n", "VISA resource name"=w2569) -> ("error out"=w2568:errorcluster, "read buffer"=w2574:string)  [unwired: 7 in]
                  n942 = case shown="\"EBAY\"" w2556 {
                    tunnel: w2570 -> [w2614 _ w2645]
                    tunnel: w2569 -> [_ _ w2648]
                    tunnel: w2568 -> [w2615 w2632 w2647]
                    tunnel: [w2608 w2632 w2643] -> w2558
                    tunnel: [w2605 "" w2640] -> w2565
                    tunnel: [w2604 bool[] [] w2639] -> w2563
                    frame "AHU" {
                      n943 = call "TesterOption (SubVI).vi"("On/Off 2"=FALSE, "Tester Option 2"=T12."Venable", "2 Options"=TRUE, "error in (no error)"=w2615, "On/Off"=TRUE, "Tester Option"=T12."K17", "VISA Refnum in"=w2614) -> ("error out"=w2617:errorcluster)  [unwired: 3 in, 1 out]
                      n944 = call "Time Delay7"("error in (no error)"=w2617) -> ("error out"=w2616:errorcluster)  [unwired: 10 in]
                      n945 = call "GetADCTester (SubVI).vi"("error in (no error)"=w2616, "GetADCTester"=T14."Current", "TimeToGet"=5, "VISA Refnum in"=w2614) -> ("error out"=w2608:errorcluster, "ADCValOutput Single"=w2610:dbl)  [unwired: 5 in, 1 out]
                      n946 = Less Or Equal?(x=w2610, y=50.0) -> (x <= y?=w2609:bool)
                      n947 = Build Array(w2609) -> (w2604:bool[])
                      n948 = for {
                        tunnel: w2604 -> [w2629] mode=indexing
                        tunnel: string[] ["Current sensor not connected!"] -> [w2626] mode=indexing
                        shift-right: [w2627] -> w2605
                        shift-left: "" -> [w2623]
                        n949 = Concatenate Strings(w2626, "\r\n") -> (w2624:string)
                        n950 = Select(t=w2623, s=w2629, f=w2624) -> (s? t:f=w2628:string)
                        n951 = Concatenate Strings(w2623, w2628) -> (w2627:string)
                      }
                    }
                    frame Default {
                    }
                    frame "EBAY" {
                      w2646 = T30 [enum."Fan", enum."Current"] items=["Term1", "Term2", "Current", "Fan", "TempCPU"]
                      n952 = call "TesterOption (SubVI).vi"("On/Off 2"=FALSE, "Tester Option 2"=T12."Venable", "2 Options"=TRUE, "error in (no error)"=w2647, "On/Off"=TRUE, "Tester Option"=T12."K17", "VISA Refnum in"=w2645) -> ("error out"=w2650:errorcluster)  [unwired: 3 in, 1 out]
                      n953 = call "Time Delay6"("error in (no error)"=w2650) -> ("error out"=w2649:errorcluster)  [unwired: 10 in]
                      n954 = call "SerialMarvinSendGet.vi"("error in (no error)"=w2649, "write buffer"="TA[3]\r\n", "VISA resource name"=w2648) -> ("error out"=w2644:errorcluster, "read buffer"=w2652:string)  [unwired: 7 in]
                      n955 = Fract/Exp String To Number(string=w2652) -> (number=w2637:dbl)  [unwired: 3 in, 1 out]
                      n956 = for {
                        tunnel: w2646 -> [w2675] mode=indexing
                        tunnel: w2645 -> [w2674]
                        tunnel: w2644 -> [w2672]
                        tunnel: [w2671] -> w2643
                        tunnel: [w2668] -> w2642 mode=indexing
                        i -> [w2669]
                        n957 = call "GetADCTester (SubVI).vi"("error in (no error)"=w2672, "GetADCTester"=w2675, "TimeToGet"=0, "VISA Refnum in"=w2674) -> ("error out"=w2671:errorcluster, "ADCValOutput Single"=w2670:dbl)  [unwired: 5 in, 1 out]
                        n958 = case shown="1" w2669 {
                          tunnel: w2670 -> [w2678 w2681 _]
                          tunnel: [w2676 w2679 FALSE] -> w2668
                          frame 1 {
                            n959 = Less Or Equal?(x=w2678, y=50.0) -> (x <= y?=w2676:bool)
                          }
                          frame 0 {
                            n960 = Greater Or Equal?(x=w2681, y=2200.0) -> (x >= y?=w2679:bool)
                          }
                          frame Default {
                          }
                        }
                      }
                      n961 = call "TAs StartTest (SubVI).vi"("Numeric"=w2637, "Enum"=enum16{"TA3", "TA2", "TA1"}."TA3") -> ("String Out"=w2635:string, "Result"=w2636:bool)  [unwired: 7 in, 1 out]
                      n962 = Build Array (concatenate)(w2636, w2642) -> (w2639:bool[])
                      n963 = Build Array (concatenate)(w2635, string[] ["AUX Fan not connected!", "Current sensor not connected!"]) -> (w2633:string[])
                      n964 = for {
                        tunnel: w2639 -> [w2658] mode=indexing
                        tunnel: w2633 -> [w2661] mode=indexing
                        shift-right: [w2663] -> w2640
                        shift-left: "" -> [w2662]
                        n965 = Concatenate Strings(w2661, "\r\n") -> (w2659:string)
                        n966 = case shown="True" w2658 {
                          tunnel: [w2666 w2667] -> w2663
                          tunnel: w2662 -> [w2665 w2667]
                          tunnel: w2659 -> [w2664 _]
                          frame False {
                            n967 = Concatenate Strings(w2665, w2664) -> (w2666:string)
                          }
                          frame True {
                          }
                        }
                      }
                    }
                  }
                  n968 = Fract/Exp String To Number(string=w2574) -> (number=w2547:dbl)  [unwired: 3 in, 1 out]
                  n969 = call "TAs StartTest (SubVI).vi"("Numeric"=w2547, "Enum"=enum16{"TA3", "TA2", "TA1"}."TA2") -> ("String Out"=w2546:string, "Result"=w2545:bool)  [unwired: 7 in, 1 out]
                  n970 = Build Array(w2548, w2546) -> (w2544:string[])
                  n971 = Build Array(w2550, w2545) -> (w2564:bool[])
                  n972 = for {
                    tunnel: w2564 -> [w2593] mode=indexing
                    tunnel: w2544 -> [w2597] mode=indexing
                    shift-right: [w2599] -> w2566
                    shift-left: "" -> [w2598]
                    tunnel: w2558 -> [w2594]
                    tunnel: [w2594] -> w2557
                    n973 = Concatenate Strings(w2597, "\r\n") -> (w2595:string)
                    n974 = case shown="False" w2593 {
                      tunnel: [w2602 w2603] -> w2599
                      tunnel: w2598 -> [w2601 w2603]
                      tunnel: w2595 -> [w2600 _]
                      frame False {
                        n975 = Concatenate Strings(w2601, w2600) -> (w2602:string)
                      }
                      frame True {
                      }
                    }
                  }
                  n976 = Build Array (concatenate)(w2564, w2563) -> (w2562:bool[])
                  n977 = And Array Elements(Boolean array=w2562) -> (logical AND=w2553:bool)
                  n978 = case shown="False" w2553 {
                    tunnel: w2566 -> [w2591 _]
                    tunnel: w2565 -> [w2590 _]
                    tunnel: w2557 -> [w2588 w2592]
                    tunnel: [w2588 w2592] -> w2555
                    frame False {
                      n979 = Concatenate Strings(w2591, w2590) -> (w2589:string)
                      n980 = One Button Dialog(message=w2589) -> ()  [unwired: 1 in, 1 out]
                    }
                    frame True {
                    }
                  }
                  n981 = case shown="False" w2553 {
                    tunnel: w2555 -> [w2586 w2587]
                    tunnel: [w2585 w2587] -> w2554
                    frame False {
                      n982 = call "Display Message to User6"("error in (no error)"=w2586) -> ("error out"=w2585:errorcluster)  [unwired: 9 in, 1 out]
                    }
                    frame True {
                    }
                  }
                  n983 = Select(t=enum16{"Stop", "Tests", "Bit test", "Start"}."Tests", s=w2553, f=enum16{"Stop", "Tests", "Bit test", "Start"}."Stop") -> (s? t:f=w2559:enum16{"Stop", "Tests", "Bit test", "Start"})
                }
                frame "Start" {
                  n984 = And(x=w2684, y=w2689) -> (x .and. y?=w2685:bool)
                  n985 = case shown="True" w2685 {
                    tunnel: w2696 -> [_ w2723]
                    tunnel: w2695 -> [_ w2714]
                    tunnel: w2694 -> [_ w2710]
                    tunnel: w2693 -> [_ w2708]
                    tunnel: w2692 -> [_ w2707]
                    tunnel: [FALSE w2706] -> w2688
                    tunnel: [w2702 w2705] -> w2683
                    tunnel: [FALSE TRUE] -> w2686
                    frame False {
                      n986 = call "Display Message to User5"() -> ("error out"=w2702:errorcluster)  [unwired: 10 in, 1 out]
                    }
                    frame True {
                      n987 = property on="VISA Tester" class="VISAName"() -> (error out=w2721:errorcluster, "Value"=w2720:refnum<visa-resource-name>)  [unwired: 2 in, 1 out]
                      n988 = call "TesterOption (SubVI).vi"("2 Options"=FALSE, "error in (no error)"=w2721, "On/Off"=FALSE, "Tester Option"=T12."Venable", "VISA Refnum in"=w2720) -> ("error out"=w2716:errorcluster)  [unwired: 5 in, 1 out]
                      n989 = call "Write panel message (SubVI).vi"("Stop BurnIn"=w2708, 4:"rpm"=w2707, 5:"rpm"=FALSE ("rpm"), "PrintTime"=FALSE, "Stop"=w2710, "error in (no error)"=w2716, "Time to wait"=3.0, "Strin"="TESTER BIT TEST OPERATION IN PROCESS\nPlease wait...", "String in"=w2714) -> ("error out"=w2715:errorcluster)  [unwired: 2 in]
                      n990 = property on="UUT SoftwareVer" class="Str"() -> ("Value"=w2704:string)  [unwired: 2 in, 2 out]
                      n991 = call "SerialMarvinSendGet.vi"("error in (no error)"=w2715, "write buffer"="VR\r\n", "VISA resource name"=w2723) -> ("error out"=w2705:errorcluster, "read buffer"=w2722:string)  [unwired: 7 in]
                      n992 = Equal?(x=w2722, y=w2704) -> (x = y?=w2706:bool)
                    }
                  }
                  n993 = case shown="False" w2688 {
                    tunnel: [enum16{"Stop", "Tests", "Bit test", "Start"}."Stop" enum16{"Stop", "Tests", "Bit test", "Start"}."Bit test"] -> w2687
                    tunnel: w2686 -> [w2697 _]
                    frame False {
                      n994 = case shown="True" w2697 {
                        frame False {
                        }
                        frame True {
                          n995 = call "Display Message to User4"() -> ()  [unwired: 10 in, 2 out]
                        }
                      }
                    }
                    frame True {
                    }
                  }
                }
              }
            }
            n996 = Bundle By Name(cluster=T8 {"VISA"="COM1", "Array Test"=[]}, "VISA"=w2381, "Array Test"=w2387) -> (w2383:T8)
            n997 = Enqueue Element(queue=w2389, element=w2383, error in (no error)=w2386) -> (queue out=w2384:refnum<queue>, error out=w2385:errorcluster)  [unwired: 2 out]
          }
          event "Report", "Stop Button": Value Change {
            w2739 = T31 1 items=["User Home"=0, "User Desktop"=1, "User Documents"=2, "User Application Data"=3, "User Preferences"=4, "User Temporary"=5, "Public Documents"=6, "Public Application Data"=7, "Public Preferences"=8, "Public Cache"=13, "System Core Libraries"=9, "System Installed Libraries"=10, "Application Files"=11, "Boot Volume Root"=12] ("system directory type")
            w2771 = "Marvin" ("section")
            n998 = event-data() -> ("CtlRef"=w2763:refnum<vi>)  [unwired: 1 in]
            n999 = local read "UUT"() -> (w2731:string)
            n1000 = call <vilib>:"Get System Directory.vi"("system directory type"=w2739) -> ("system directory"=w2738:path)  [unwired: 10 in]
            n1001 = Build Path(base path=w2738, name or relative path="MarvinReports") -> (appended path=w2800:path)
            n1002 = property on="CAN Status" class="Bool (strict)"() -> ("Value"=w2742:bool)  [unwired: 2 in, 2 out]
            n1003 = property on="Status" class="Bool (strict)"() -> ("Value"=w2743:bool)  [unwired: 2 in, 2 out]
            n1004 = case shown="\"AHU\"" w2731 {
              tunnel: ["REV EBAY" ("key") "REV AHU" ("key")] -> w2769
              frame "EBAY", Default {
              }
              frame "AHU" {
              }
            }
            n1005 = call <vilib>:"Check if File or Folder Exists.vi"("path"=w2800) -> ("error out"=w2798:errorcluster, "file or folder exists?"=w2801:bool, "dup path"=w2799:path)  [unwired: 8 in]
            n1006 = And(x=w2743, y=w2742) -> (x .and. y?=w2744:bool)
            n1007 = case shown="False" w2801 {
              tunnel: w2798 -> [w2865 w2866]
              tunnel: w2799 -> [w2864 w2867]
              tunnel: [w2863 w2867] -> w2741
              tunnel: [w2862 w2866] -> w2803
              frame False {
                n1008 = Create Folder(path (use dialog)=w2864, error in=w2865) -> (created path=w2863:path, error out=w2862:errorcluster)  [unwired: 1 in, 1 out]
              }
              frame True {
              }
            }
            n1009 = case shown="True" w2744 {
              tunnel: [w2810 w2830] -> w2787
              tunnel: [w2810 w2829] -> w2734
              tunnel: w2764 -> [_ w2818]
              tunnel: [w2810 w2823] -> w2733
              tunnel: [w2810 w2822] -> w2730
              tunnel: [w2810 w2826] -> w2757
              tunnel: [w2810 w2825] -> w2736
              tunnel: [w2810 w2814] -> w2737
              frame False {
                (unwired) "47"
                (unwired) " 413-8005_47_AHU"
                (unwired) "413-8005-1-47"
                (unwired) "5.3.9" ("read buffer")
                (unwired) "95"
                (unwired) "414-8005_95_EBAY_"
                (unwired) "414-8005-95"
                (unwired) "414-8005-95   "
                w2810 = "N_A" ("read buffer")
                n1010 = disable-structure shown="Disabled" {
                  frame Disabled {
                    n1011 = call "Display Message to User7"() -> ()  [unwired: 10 in, 2 out]
                  }
                  frame Enabled {
                  }
                }
                n1012 = Decimal String To Number(string="1" ("Value")) -> (number=w2811:i32)  [unwired: 2 in, 1 out]
                n1013 = Number To Decimal String(number=w2811, width (-)=i16 4) -> ()  [unwired: 1 out]
              }
              frame True {
                n1014 = call "SerialMarvinSendGet.vi"("write buffer"="SN\r\n", "VISA resource name"=w2818) -> ("error out"=w2817:errorcluster, "read buffer"=w2820:string)  [unwired: 8 in]
                n1015 = call "Time Delay2"("error in (no error)"=w2817) -> ("error out"=w2816:errorcluster)  [unwired: 10 in]
                n1016 = Decimal String To Number(string=w2820) -> (number=w2819:i32)  [unwired: 2 in, 1 out]
                n1017 = Number To Decimal String(number=w2819, width (-)=i16 4) -> (decimal integer string=w2823:string)
                n1018 = call "SerialMarvinSendGet.vi"("error in (no error)"=w2816, "write buffer"="VR\r\n", "VISA resource name"=w2818) -> ("error out"=w2827:errorcluster, "read buffer"=w2822:string)  [unwired: 7 in]
                n1019 = property on="UUT" class="DigNum (strict)"(error in=w2827) -> ("Value"=w2815:u8)  [unwired: 1 in, 2 out]
                n1020 = call "SentenceFromFile (SubVI).vi"("UUT"=w2815) -> ("Sentence"=w2814:string)  [unwired: 9 in, 1 out]
                n1021 = case shown="95, Default" w2815 {
                  tunnel: ["414-8005_95_EBAY_" " 413-8005_47_AHU" " 413-8005_63_AHU"] -> w2830
                  tunnel: ["414-8005-95   " w2836 w2839] -> w2829
                  tunnel: ["414-8005-95" w2836 w2839] -> w2826
                  tunnel: ["95" "47" "63"] -> w2825
                  frame 95, Default {
                  }
                  frame 47 {
                    w2836 = "413-8005-1-47"
                    (unwired) "AHU-L (47) 413-8005-1"
                  }
                  frame 63 {
                    w2839 = "413-8005-2-63"
                    (unwired) "AHU-R (63) 413-8005-2"
                  }
                }
              }
            }
            n1022 = Get Date/Time String(want seconds? (F)=TRUE) -> (date string=w2802:string)  [unwired: 2 in, 1 out]
            n1023 = call <vilib>:"Open Config Data.vi"("create file if necessary (T)"=FALSE, "configuration file path"=w2766) -> ("refnum"=w2778:T11)  [unwired: 1 in, 8 out]
            n1024 = property on="Logger Path" class="Path"(error in=w2803, "Value"=w2741, "StartPath"=w2741) -> (error out=w2781:errorcluster)  [unwired: 1 in, 1 out]
            n1025 = Search and Replace String(replace all?=TRUE ("replace all? (F)"), input string=w2802, search string="/") -> (result string=w2784:string)  [unwired: 5 in, 3 out]
            n1026 = call-poly <vilib>:"Read Key.vi"("section"=w2771, "key"=w2769, "refnum"=w2778) -> ("error out"=w2773:errorcluster, "value"=w2776:string, "refnum out"=w2775:T11)  [unwired: 5 in, 1 out]
            n1027 = call-poly <vilib>:"Read Key.vi"("section"=w2771, "error in (no error)"=w2773, "key"="Tester Software Ver", "refnum"=w2775) -> ("error out"=w2770:errorcluster, "value"=w2735:string, "refnum out"=w2774:T11)  [unwired: 4 in, 1 out]
            n1028 = Concatenate Strings("ATR" ("string"), w2787, w2733, "_", w2784, ".docx" ("string")) -> (w2782:string)
            n1029 = call <vilib>:"Close Config Data.vi"("error in (no error)"=w2770, "refnum"=w2774) -> ()  [unwired: 8 in, 2 out]
            n1030 = Build Path(base path=w2741, name or relative path=w2782) -> (appended path=w2783:path)
            n1031 = Concatenate Strings("  Rev-" ("string"), w2776) -> (w2765:string)
            n1032 = while {
              tunnel: w2782 -> [w2847]
              tunnel: w2741 -> [w2844]
              shift-right: [w2846] -> w2780
              shift-left: w2783 -> [w2845]
              shift-right: [w2842] -> w2767
              shift-left: w2768 -> [w2843]
              tunnel: w2781 -> [w2848]
              tunnel: [w2849] -> w2740
              stop <- w2841 continue-if-true
              n1033 = call <vilib>:"Check if File or Folder Exists.vi"("error in (no error)"=w2848, "path"=w2845) -> ("error out"=w2849:errorcluster, "file or folder exists?"=w2841:bool)  [unwired: 7 in, 1 out]
              n1034 = case shown="True" w2841 {
                tunnel: w2847 -> [_ w2861]
                tunnel: w2843 -> [_ w2853]
                tunnel: [w2851 w2858] -> w2846
                tunnel: w2845 -> [w2851 _]
                tunnel: w2844 -> [_ w2859]
                tunnel: [1 w2852] -> w2842
                frame False {
                }
                frame True {
                  w2854 = ".docx" ("search string")
                  n1035 = Search and Replace String(input string=w2861, search string=w2854) -> (result string=w2860:string)  [unwired: 6 in, 3 out]
                  n1036 = Number To Decimal String(number=w2853) -> (decimal integer string=w2856:string)  [unwired: 1 in]
                  n1037 = call <vilib>:"Space Constant.vi"() -> ("String"=w2855:string)
                  n1038 = Concatenate Strings(w2860, w2855, w2856, w2854) -> (w2857:string)
                  n1039 = Build Path(base path=w2859, name or relative path=w2857) -> (appended path=w2858:path)
                  n1040 = Increment(x=w2853) -> (x+1=w2852:i32)
                }
              }
            }
            n1041 = property on="DSP Board S/N" class="Str"() -> ("Value"=w2729:string)  [unwired: 2 in, 2 out]
            n1042 = property on="POWER Board S/N" class="Str"() -> ("Value"=w2728:string)  [unwired: 2 in, 2 out]
            n1043 = call "HeaderBis.vi"("UUTHeader"=w2731, "UA"=w2736, "POWER SN"=w2728, "Revision Param"=w2737, "P/N UUT"=w2734, "DSP SN"=w2729, "Driver S/N"=w2733, "VR"=w2730, "Oper."=w2732, "Tester Software Ver"=w2735) -> ("table header"=w2727:string, "Array"=w2726:string[][])  [unwired: 3 in, 1 out]
            n1044 = Open/Create/Replace File(file path (use dialog)=w2780, error in=w2740, operation (0:open)=T25."create") -> (error out=w2793:errorcluster)  [unwired: 3 in, 2 out]
            n1045 = control-ref of="ATR"() -> (w2805:refnum<vi>)
            n1046 = property class="Tbl (strict)"(reference=w2805, error in=w2793) -> ("Value"=w2806:string[][])  [unwired: 2 out]
            n1047 = call "MarvinReport.vi"("HEADER1"=w2727, "ATR Or"=w2805, "Steps   pfull"=w2806, "Footer UUT"=w2757, "pageNum"=3, "InputHeaderArray"=w2726, "FILE NAME"=w2782, "Report Folder"=w2780, "REV"=w2765, "Test-Conductor"=w2732) -> ("error out"=w2752:errorcluster)  [unwired: 4 in, 1 out]
            n1048 = call <vilib>:"Clear Errors.vi"("error in (no error)"=w2752) -> ("error out"=w2751:errorcluster)  [unwired: 5 in, 1 out]
            n1049 = property class="Bool (strict)"(reference=w2763, error in=w2751) -> ("BoolText.Text"=w2762:string)  [unwired: 2 out]
            n1050 = Equal?(x=w2762, y="Report") -> (x = y?=w2756:bool)
            n1051 = Select(t=T10."MainProgram", s=w2756, f=T10."Stop") -> (s? t:f=w2759:T10)
            n1052 = Select(t="Save Report...", s=w2756, f="Program Stopped...\r\nPlease turn OFF All Power sinks") -> (s? t:f=w2754:string)
            n1053 = property on="Report" class="Bool (strict)"(error in=w2751, "Value"=FALSE ("Report")) -> (error out=w2745:errorcluster)  [unwired: 1 in, 1 out]
            n1054 = property on="VISA Tester" class="VISAName"() -> ("Value"=w2749:refnum<visa-resource-name>)  [unwired: 2 in, 2 out]
            n1055 = property on="Pannel User Message" class="Str"("Value"=w2754) -> ()  [unwired: 2 in, 2 out]
            n1056 = call "TesterOption (SubVI).vi"("2 Options"=FALSE, "error in (no error)"=w2745, "On/Off"=FALSE, "Tester Option"=T12."Venable", "VISA Refnum in"=w2749) -> ()  [unwired: 5 in, 2 out]
          }
          event "Help Button": Value Change {
            n1057 = event-data() -> ()  [unwired: 1 in, 6 out]
            n1058 = vi-ref "Help.vi"() -> (w2880:refnum<vi>)
            n1059 = invoke class="VI" method="FP.Open"(reference=w2880, error in=w2878, "Activate"=TRUE ("Activate?"), "State"=T22."Standard") -> (error out=w2879:errorcluster)  [unwired: 1 in, 4 out]
            n1060 = call "Help.vi"("error in"=w2879, "TesterSWVersion"=w2870) -> ("error out"=w2877:errorcluster)  [unwired: 6 in]
            n1061 = property on="Help Button" class="Bool (strict)"("Value"=FALSE ("Help Button")) -> ()  [unwired: 2 in, 2 out]
          }
          event "Serial Com": Value Change {
            n1062 = event-data() -> ()  [unwired: 1 in, 6 out]
            n1063 = property on="Serial Com" class="Bool"(error in=w2890, "Visible"=FALSE) -> (error out=w2894:errorcluster)  [unwired: 1 in, 1 out]
            n1064 = property on="VISA Marvin" class="VISAName"(error in=w2894, "Visible"=TRUE) -> (error out=w2891:errorcluster)  [unwired: 1 in, 1 out]
          }
          event "VISA Marvin": Value Change {
            n1065 = event-data() -> ()  [unwired: 1 in, 6 out]
            n1066 = property on="Serial Com" class="Bool"(error in=w2898, "Visible"=FALSE) -> (error out=w2897:errorcluster)  [unwired: 1 in, 1 out]
            n1067 = control-ref of="This VI"() -> (w2909:refnum<vi>)
            n1068 = property on="Pannel User Message" class="Str"(error in=w2898, "Value"="Serial connection in process" ("Pannel User Message")) -> ()  [unwired: 1 in, 2 out]
            n1069 = call "Serial InitMarvin.vi"("error in (no error)"=w2897, "VI reference (current VI)"=w2909, "VISA Refnum in"="VISA Marvin") -> ("error out"=w2901:errorcluster, "Boolean"=w2899:bool)  [unwired: 7 in]
            n1070 = property on="VISA Marvin" class="VISAName"(error in=w2901, "Visible"=FALSE) -> (error out=w2912:errorcluster)  [unwired: 1 in, 1 out]
            n1071 = property on="Serial Com" class="Bool"(error in=w2912, "Visible"=TRUE) -> (error out=w2908:errorcluster)  [unwired: 1 in, 1 out]
            n1072 = case shown="True" w2899 {
              tunnel: w2908 -> [w2915 w2927]
              tunnel: "VISA Marvin" -> [w2916 w2924]
              tunnel: [w2916 w2923] -> w2903
              tunnel: [w2915 w2922] -> w2902
              frame False {
              }
              frame True {
                n1073 = call "SerialMarvinSendGet.vi"("error in (no error)"=w2927, "Clear Log"=FALSE, "write buffer"="VC\r\n", "VISA resource name"=w2924) -> ("error out"=w2926:errorcluster, "read buffer"=w2920:string)  [unwired: 6 in]
                n1074 = Decimal String To Number(string=w2920) -> (number=w2919:i32)  [unwired: 2 in, 1 out]
                n1075 = Less Or Equal?(x=w2919, y=50) -> (x <= y?=w2917:bool)
                n1076 = property on="Status" class="Bool (strict)"("Value"=w2917) -> ()  [unwired: 2 in, 2 out]
                n1077 = case shown="True" w2917 {
                  tunnel: w2926 -> [w2928 w2957]
                  tunnel: w2924 -> [w2929 w2956]
                  tunnel: [w2929 w2947] -> w2923
                  tunnel: [w2928 w2930] -> w2922
                  frame False {
                  }
                  frame True {
                    n1078 = call <vilib>:"Clear Errors.vi"("error in (no error)"=w2957) -> ("error out"=w2958:errorcluster)  [unwired: 5 in, 1 out]
                    n1079 = control-ref of="ATR"() -> (w2944:refnum<vi>)
                    n1080 = VISA Flush I/O Buffer(VISA resource name=w2956, error in (no error)=w2958) -> (VISA resource name out=w2947:refnum<visa-resource-name>, error out=w2955:errorcluster)  [unwired: 1 in]
                    n1081 = call "Display Message to User2"("error in (no error)"=w2955) -> ("error out"=w2954:errorcluster, "Yes"=w2953:bool)  [unwired: 9 in]
                    n1082 = case shown="True" w2953 {
                      tunnel: w2954 -> [w2959 w2981]
                      tunnel: [w2959 w2960] -> w2952
                      tunnel: w2947 -> [_ w2978]
                      frame False {
                      }
                      frame True {
                        w2966 = FALSE ("2 Options")
                        n1083 = property on="UUT" class="DigNum (strict)"() -> ("Value"=w2980:u8)  [unwired: 2 in, 2 out]
                        n1084 = call "SetParam.vi"("RS"=TRUE, "error in (no error)"=w2981, "Param to Set in"=w2980, "Visa"=w2978) -> ("error out"=w2961:errorcluster)  [unwired: 7 in]
                        n1085 = control-ref of="Pannel User Message"() -> (w2977:refnum<vi>)
                        n1086 = control-ref of="Stop Burn-in"() -> (w2975:refnum<vi>)
                        n1087 = control-ref of="Stop Button"() -> (w2976:refnum<vi>)
                        n1088 = control-ref of="Motor Speed RPM"() -> (w2974:refnum<vi>)
                        n1089 = property on="VISA Tester" class="VISAName"() -> ("Value"=w2970:refnum<visa-resource-name>)  [unwired: 2 in, 2 out]
                        n1090 = call "TesterOption (SubVI).vi"("2 Options"=w2966, "error in (no error)"=w2961, "On/Off"=FALSE, "Tester Option"=T12."Power", "VISA Refnum in"=w2970) -> ("error out"=w2971:errorcluster, "VISA Refnum out"=w2973:refnum<visa-resource-name>)  [unwired: 5 in]
                        n1091 = call "Write panel message (SubVI).vi"("Stop BurnIn"=w2975, "rpm"=w2974, "PrintTime"=TRUE, "Stop"=w2976, "error in (no error)"=w2971, "Time to wait"=20.0, "Strin"="Restart the UUT\nPlease wait...", "String in"=w2977) -> ("error out"=w2972:errorcluster)  [unwired: 3 in]
                        n1092 = call "TesterOption (SubVI).vi"("2 Options"=w2966, "error in (no error)"=w2972, "On/Off"=FALSE, "Tester Option"=T12."Venable", "VISA Refnum in"=w2973) -> ("error out"=w2960:errorcluster)  [unwired: 5 in, 1 out]
                      }
                    }
                    n1093 = call "Find_Number_LineMARVIN from number.vi"("Test Paragraph"="2.1", "TableIn"=w2944) -> ("Line number"=w2945:i32)  [unwired: 3 in, 3 out]
                    n1094 = call "SerialMarvinSendGet.vi"("error in (no error)"=w2952, "write buffer"="SN\r\n", "VISA resource name"=w2947) -> ("error out"=w2948:errorcluster, "read buffer"=w2937:string)  [unwired: 7 in]
                    n1095 = call "SerialMarvinSendGet.vi"("error in (no error)"=w2948, "write buffer"="AO[1]\r\n", "VISA resource name"=w2947) -> ("error out"=w2942:errorcluster, "read buffer"=w2943:string)  [unwired: 7 in]
                    n1096 = Fract/Exp String To Number(string=w2943) -> (number=w2939:dbl)  [unwired: 3 in, 1 out]
                    n1097 = In Range and Coerce(upper limit=0.1 ("x"), x=w2939, lower limit=-0.1) -> (In Range?=w2938:bool)  [unwired: 1 out]
                    n1098 = call "PassOrFail (SubVI).vi"("Test#"="2", "index (row)"=w2945, "error in (no error)"=w2942, "Data in"=w2939, "Pass?Fail"=w2938, "Table in"=w2944) -> ("error out"=w2931:errorcluster)  [unwired: 5 in]
                    n1099 = property on="VISA Marvin" class="VISAName"(error in=w2931) -> (error out=w2934:errorcluster, "Value"=w2935:refnum<visa-resource-name>)  [unwired: 1 in, 1 out]
                    n1100 = call "SerialMarvinSendGet.vi"("error in (no error)"=w2934, "Clear Log"=FALSE, "write buffer"="EP=1\r\nMD[1]=1\r\n", "VISA resource name"=w2935) -> ("error out"=w2930:errorcluster)  [unwired: 6 in, 1 out]
                    n1101 = property on="UUT SN Report" class="Str"("Value"=w2937) -> ()  [unwired: 2 in, 2 out]
                    n1102 = Decimal String To Number(string=w2937) -> (number=→"Current SN":i32)  [unwired: 2 in, 1 out]
                  }
                }
              }
            }
          }
          event "Refresh Button": Value Change {
            n1103 = event-data() -> ()  [unwired: 1 in, 6 out]
          }
          event "Settings": Value Change {
            n1104 = event-data() -> ()  [unwired: 1 in, 6 out]
            n1105 = control-ref of="VISA Tester"() -> (w2993:refnum<vi>)
            n1106 = control-ref of="UUT"() -> (w2991:refnum<vi>)
            n1107 = property on="Status" class="Bool (strict)"() -> ("Value"=w2995:bool)  [unwired: 2 in, 2 out]
            n1108 = case shown="True" w2995 {
              tunnel: w3001 -> [_ w3013]
              tunnel: [w3002 w3008] -> w2996
              tunnel: w2994 -> [_ w3007]
              tunnel: w2993 -> [_ w3006]
              tunnel: w2992 -> [_ w3005]
              tunnel: w2991 -> [_ w3004]
              frame False {
                n1109 = call "Display Message to User8"() -> ("error out"=w3002:errorcluster)  [unwired: 10 in, 1 out]
              }
              frame True {
                n1110 = vi-ref "Calibration (SubVI).vi"() -> (w3012:refnum<vi>)
                n1111 = invoke class="VI" method="FP.Open"(reference=w3012, error in=w3013, "Activate"=TRUE ("Activate?"), "State"=T22."Standard") -> (error out=w3009:errorcluster)  [unwired: 1 in, 4 out]
                n1112 = call "Calibration (SubVI).vi"("VISA UUT"=w3007, "error constant"=w3009, "UUT"=w3004, "CAN Cluster in"=w3005, "Visa Tester"=w3006) -> ("error constant 2"=w3008:errorcluster, "AO[1]Meas"=→"Cal":dbl)  [unwired: 5 in]
              }
            }
          }
        }
      }
      frame "Initialize" {
        w3019 = FALSE ("Visible")
        w3020 = FALSE ("Visible")
        w3021 = FALSE ("Visible")
        w3022 = FALSE ("Visible")
        w3033 = refnum<visa-resource-name> "COM1" ("VISA resource name")
        w3024 = FALSE ("Visible")
        w3017 = FALSE ("Serial Status")
        n1113 = property on="ComTestResult" class="Bool (strict)"("Value"=w3022) -> ()  [unwired: 2 in, 2 out]
        n1114 = property on="VenableResult" class="Bool (strict)"("Value"=w3022) -> ()  [unwired: 2 in, 2 out]
        n1115 = property on="VenableDirectionResult" class="Bool (strict)"("Value"=w3022) -> ()  [unwired: 2 in, 2 out]
        n1116 = property on="SpeedResult" class="Bool (strict)"("Value"=w3022) -> ()  [unwired: 2 in, 2 out]
        n1117 = property on="Serial Com" class="Bool"(error in=errorcluster {"status"=FALSE, "code"=0, "source"=""} ("error out"), "Visible"=TRUE) -> (error out=w3035:errorcluster)  [unwired: 1 in, 1 out]
        n1118 = property on="AuxiOFFResult" class="Bool (strict)"("Value"=w3021) -> ()  [unwired: 2 in, 2 out]
        n1119 = property on="AuxiONResult" class="Bool (strict)"("Value"=w3021) -> ()  [unwired: 2 in, 2 out]
        n1120 = property on="VisualInspectionResult" class="Bool (strict)"("Value"=w3021) -> ()  [unwired: 2 in, 2 out]
        n1121 = property on="SensCalResult" class="Bool (strict)"("Value"=w3021) -> ()  [unwired: 2 in, 2 out]
        n1122 = property on="VISA Marvin" class="VISAName"(error in=w3035, "Visible"=w3024, "Value"=w3033) -> (error out=w3025:errorcluster)  [unwired: 1 in, 1 out]
        n1123 = property on="Stop Burn-in" class="Bool (strict)"(error in=w3025, "Visible"=w3024) -> (error out=w3018:errorcluster)  [unwired: 1 in, 1 out]
        n1124 = property on="BurnDC" class="Bool (strict)"("Value"=w3020) -> ()  [unwired: 2 in, 2 out]
        n1125 = property on="BurnTemp" class="Bool (strict)"("Value"=w3020) -> ()  [unwired: 2 in, 2 out]
        n1126 = property on="BurnSpeed" class="Bool (strict)"("Value"=w3020) -> ()  [unwired: 2 in, 2 out]
        n1127 = property on="BurnResult" class="Bool (strict)"("Value"=w3020) -> ()  [unwired: 2 in, 2 out]
        n1128 = property on="Refresh Button" class="Bool (strict)"(error in=w3018, "Value"=FALSE ("Refresh Button")) -> ()  [unwired: 1 in, 2 out]
        n1129 = property on="StopTimeResult" class="Bool (strict)"("Value"=w3019) -> ()  [unwired: 2 in, 2 out]
        n1130 = property on="MotorTempResult" class="Bool (strict)"("Value"=w3019) -> ()  [unwired: 2 in, 2 out]
        n1131 = property on="TempControlResult" class="Bool (strict)"("Value"=w3019) -> ()  [unwired: 2 in, 2 out]
        n1132 = property on="Automation" class="Bool (strict)"("Value"=w3019) -> ()  [unwired: 2 in, 2 out]
        n1133 = flat-sequence {
          tunnel: w3018 -> [w3037]
          tunnel: [w3037] -> w3015
          tunnel: [w3039] -> w3031
          tunnel: w3015 -> [w3039]
          tunnel: [w3051] -> w3030
          tunnel: w3031 -> [w3052]
          tunnel: [w3052] -> w3029
          frame #0 {
          }
          frame #1 {
            w3042 = u32 4294967295  # AccMask
            w3038 = T4 0 items=["使用Flash参数", "使用界面设置参数"] ("InitFlag")
            w3040 = T6 0 items=["normal operation", "Listen-only mode", "test mode"]  # Mode
            w3041 = T5 3 items=["接收所有类型"=1, "只接收标准帧"=2, "只接收扩展帧"=3] ("Fliter")
            w3046 = u8 10 items=["5k bps"=1, "10k bps"=2, "20k bps"=3, "40k bps"=4, "50k bps"=5, "80k bps"=6, "100k bps"=7, "125k bps"=8, "200k bps"=9, "250k bps"=10, "400k bps"=11, "500k bps"=12, "666k bps"=13, "800k bps"=14, "1000k bps"=15, "33.33k bps"=16, "66.66k bps"=17, "83.33k bps"=18]  # kBaudRate
            w3043 = u32 0  # AccCode
            w3044 = T2 4 items=["USB-CAN"=3, "USB-CAN2"=4] ("DevType")
            w3045 = T7 {"DevType"=3, "DevIndex"=0, "CanIndex"=0, "VCI_INIT_CONFIG"={"AccCode"=0, "AccMask"=0, "InitFlag"=1, "Fliter"=7, "Timing0"=0, "Timing1"=0, "Mode"=0}}  # Config
            # "CANalystII"
            n1134 = call "Demo_GetT0T1.vi"("kBaudRate"=w3046) -> ("Timing0"=w3048:u8, "Timing1"=w3049:u8)
            n1135 = Bundle By Name(cluster=w3045, "DevType"=w3044, "CanIndex"="Channel 2", "VCI_INIT_CONFIG.AccCode"=w3043, "VCI_INIT_CONFIG.AccMask"=w3042, "VCI_INIT_CONFIG.InitFlag"=w3038, "VCI_INIT_CONFIG.Fliter"=w3041, "VCI_INIT_CONFIG.Timing0"=w3048, "VCI_INIT_CONFIG.Timing1"=w3049, "VCI_INIT_CONFIG.Mode"=w3040) -> (→"Config_CANAT":T7)
          }
          frame #2 {
            w3053 = u16 284 items=["1M"=20, "500K"=28, "250K"=284, "125K"=796, "100K"=17199, "50K"=18223, "20K"=21295, "10K"=26415, "5K"=32639] ("baud in")
            n1136 = control-ref of="Config_CANAT"() -> (w3051:refnum<vi>)
            n1137 = call "InitCAN_ATII.vi"("Config"=w3051) -> ("Sts"=→"CAN Status":bool)
            n1138 = call "ChangeCANBaud.vi"("baud in"=w3053, "reference"=w3051) -> ()
          }
        }
        "Status" <- w3017
        "Test Failed" <- w3017
      }
    }
  }
  n1139 = property on="Settings" class="Bool (strict)"("Visible"=w20) -> ()  [unwired: 2 in, 2 out]
  n1140 = property on="Cal" class="DigNum (strict)"("Visible"=w20) -> ()  [unwired: 2 in, 2 out]
  n1141 = disable-structure shown="Disabled" {
    frame Disabled {
      w3055 = T20."Disabled and Grayed Out" ("Disabled")
      w3056 = FALSE ("Start")
      n1142 = property on="VISA Tester" class="VISAName" props=["Value"]() -> ()  [unwired: 2 in, 3 out]
      n1143 = property on="Current SN" class="DigNum (strict)" props=["Value"]() -> ()  [unwired: 2 in, 3 out]
      n1144 = property on="UUT" class="DigNum (strict)" props=["Value"]() -> ()  [unwired: 2 in, 3 out]
      n1145 = property on="Status" class="Bool (strict)" props=["Value"]() -> ()  [unwired: 2 in, 3 out]
      n1146 = property on="UUT SoftwareVer" class="Str" props=["Value"]() -> ()  [unwired: 2 in, 3 out]
      n1147 = property on="Next SN" class="DigNum (strict)" props=["Value"]() -> ()  [unwired: 3 in, 2 out]
      n1148 = property on="Start" class="Bool (strict)"("Value"=w3056, "DisabledEnum"=w3055) -> ()  [unwired: 2 in, 2 out]
      n1149 = property on="Report" class="Bool (strict)"("Value"=w3056, "DisabledEnum"=w3055) -> ()  [unwired: 2 in, 2 out]
    }
    frame Enabled {
    }
  }
  n1150 = disable-structure shown="Disabled" {
    frame Disabled {
      (unwired) 0.02003173828125 ("x")
      n1151 = control-ref of="Stop Burn-in"() -> ()  [unwired: 1 out]
      n1152 = control-ref of="Stop Button"() -> ()  [unwired: 1 out]
      n1153 = control-ref of="Motor Speed RPM"() -> ()  [unwired: 1 out]
      n1154 = control-ref of="Config_CANAT"() -> ()  [unwired: 1 out]
      n1155 = control-ref of="UUT"() -> ()  [unwired: 1 out]
      n1156 = call "GetADCTester (SubVI).vi"() -> ()  [unwired: 9 in, 3 out]
      n1157 = call "CANSendMotorSpeed.vi"() -> ()  [unwired: 11 in, 1 out]
      n1158 = control-ref of="Config_CANAT"() -> ()  [unwired: 1 out]
      n1159 = call "Find_Number_LineMARVIN from number.vi"() -> ()  [unwired: 5 in, 4 out]
      n1160 = property on="UUT" class="DigNum (strict)" props=["Value"]() -> ()  [unwired: 2 in, 3 out]
      n1161 = control-ref of="UUT"() -> ()  [unwired: 1 out]
      n1162 = call "DegToDAC (SubVI).vi"() -> ()  [unwired: 10 in, 2 out]
      n1163 = call "Write panel message (SubVI).vi"() -> ()  [unwired: 11 in, 1 out]
      n1164 = property on="VISA Tester" class="VISAName" props=["Value"]() -> ()  [unwired: 2 in, 3 out]
      n1165 = control-ref of="ATR"() -> ()  [unwired: 1 out]
      n1166 = call "TesterOption (SubVI).vi"() -> ()  [unwired: 10 in, 2 out]
      n1167 = call "TesterOption (SubVI).vi"() -> ()  [unwired: 10 in, 2 out]
      n1168 = call "PassOrFail (SubVI).vi"() -> ()  [unwired: 11 in, 1 out]
    }
    frame Enabled {
    }
  }
  n1169 = disable-structure shown="Disabled" {
    frame Disabled {
      n1170 = flat-sequence {
        frame #0 {
          n1171 = call "CANSendMotorSpeed.vi"("Remote"=TRUE, "Motor Speed RPM"=u16 0) -> ("error out"=w3058:errorcluster, "UUT"=w3061:refnum<vi>)  [unwired: 8 in]
          n1172 = property on="VISA Tester" class="VISAName"() -> ("Value"=w3057:refnum<visa-resource-name>)  [unwired: 2 in, 2 out]
          n1173 = call "TesterOption (SubVI).vi"("error in (no error)"=w3058, "On/Off"=FALSE, "Tester Option"=T12."Power", "VISA Refnum in"=w3057) -> ()  [unwired: 6 in, 2 out]
        }
      }
    }
    frame Enabled {
    }
  }
  "Pannel User Message" <- w19
